vi "Parse BOM Raw Data Array.vi"(8 "Error in":errorcluster caption="Error in (no error)", 11 "BOM JSON String":string="[\n  {\n    \"id\":57,\n    \"order\":\"2.00000000000000000000\",\n    \"Full PN\":\"40-00000 Rev.A\",\n    \"External Part Number\":\"RRJTLR\",\n    \"Manufacturer\":[\n      {\n        \"id\":2,\n        \"value\":\"Schlegel Electrokontakt GMBH\",\n        \"order\":\"2.00000000000000000000\"\n      }\n    ],\n    \"System\":{\n      \"id\":2963,\n      \"value\":\"DC Power Supply\",\n      \"color\":\"orange\"\n    },\n    \"Item description\":\"Silver pushbutton with illuminated ring\",\n    \"Price per unit\":\"0.00\",\n    \"Image\":[\n      {\n        \"url\":\"http://localhost/media/user_files/vs8lqWLDz7IiCZOwmtUNUbGmxWH526uQ_3725ba00b9b12365f0e4d102f8b4c18b09270bde56499f1310e5468db4989185.jpg\",\n        \"thumbnails\":{\n          \"tiny\":{\n            \"url\":\"http://localhost/media/thumbnails/tiny/vs8lqWLDz7IiCZOwmtUNUbGmxWH526uQ_3725ba00b9b12365f0e4d102f8b4c18b09270bde56499f1310e5468db4989185.jpg\",\n            \"width\":null,\n            \"height\":21\n          },\n          \"small\":{\n            \"url\":\"http://localhost/media/thumbnails/small/vs8lqWLDz7IiCZOwmtUNUbGmxWH526uQ_3725ba00b9b12365f0e4d102f8b4c18b09270bde56499f1310e5468db4989185.jpg\",\n            \"width\":48,\n            \"height\":48\n          },\n          \"card_cover\":{\n            \"url\":\"http://localhost/media/thumbnails/card_cover/vs8lqWLDz7IiCZOwmtUNUbGmxWH526uQ_3725ba00b9b12365f0e4d102f8b4c18b09270bde56499f1310e5468db4989185.jpg\",\n            \"width\":300,\n            \"height\":160\n          }\n        },\n        \"visible_name\":\"2XATeTQaoip3EBPiJcHf6fjdvHM94na...de56499f1310e5468db4989185.jpg\",\n        \"name\":\"vs8lqWLDz7IiCZOwmtUNUbGmxWH526uQ_3725ba00b9b12365f0e4d102f8b4c18b09270bde56499f1310e5468db4989185.jpg\",\n        \"size\":3722,\n        \"mime_type\":\"image/jpeg\",\n        \"is_image\":true,\n        \"image_width\":300,\n        \"image_height\":168,\n        \"uploaded_at\":\"2025-05-04T14:40:33.054106+00:00\"\n      }\n    ],\n    \"Source\":\"kahane.co.il\",\n    \"Order Items\":[\n      {\n        \"id\":1,\n        \"value\":\"8e1b2002-0c82-4bb7-87aa-3665b154ad1b\",\n        \"order\":\"1.00000000000000000000\"\n      }\n    ],\n    \"Datasheet\":[],\n    \"Part of a set\":[\n      {\n        \"id\":57,\n        \"value\":\"40-00000 Rev.A\",\n        \"order\":\"2.00000000000000000000\"\n      },\n      {\n        \"id\":58,\n        \"value\":\"40-00001 Rev.A\",\n        \"order\":\"3.00000000000000000000\"\n      },\n      {\n        \"id\":59,\n        \"value\":\"40-00002 Rev.A\",\n        \"order\":\"4.00000000000000000000\"\n      }\n    ],\n    \"State\":{\n      \"id\":3001,\n      \"value\":\"Unknown\",\n      \"color\":\"dark-orange\"\n    },\n    \"Part Number\":\"40-00000\",\n    \"Revision\":\"A\",\n    \"Notes\":null,\n    \"Sourced By\":null,\n    \"Containing\":[],\n    \"Contained by\":[]\n  },\n  {\n    \"id\":58,\n    \"order\":\"3.00000000000000000000\",\n    \"Full PN\":\"40-00001 Rev.A\",\n    \"External Part Number\":\"BFL5\",\n    \"Manufacturer\":[\n      {\n        \"id\":2,\n        \"value\":\"Schlegel Electrokontakt GMBH\",\n        \"order\":\"2.00000000000000000000\"\n      }\n    ],\n    \"System\":{\n      \"id\":2963,\n      \"value\":\"DC Power Supply\",\n      \"color\":\"orange\"\n    },\n    \"Item description\":\"lluminated contact block, maintained (latching), fits W2x4,6d light bulb\",\n    \"Price per unit\":\"0.00\",\n    \"Image\":[\n      {\n        \"url\":\"http://localhost/media/user_files/xij9XnHAyoORm72XwG7yoW01mk4UuKpd_da0cb6cb7c3498cd2d6cf9448262cb0dac37b09af222fbe05ff221e70527cfe5.jpg\",\n        \"thumbnails\":{\n          \"tiny\":{\n            \"url\":\"http://localhost/media/thumbnails/tiny/xij9XnHAyoORm72XwG7yoW01mk4UuKpd_da0cb6cb7c3498cd2d6cf9448262cb0dac37b09af222fbe05ff221e70527cfe5.jpg\",\n            \"width\":null,\n            \"height\":21\n          },\n          \"small\":{\n            \"url\":\"http://localhost/media/thumbnails/small/xij9XnHAyoORm72XwG7yoW01mk4UuKpd_da0cb6cb7c3498cd2d6cf9448262cb0dac37b09af222fbe05ff221e70527cfe5.jpg\",\n            \"width\":48,\n            \"height\":48\n          },\n          \"card_cover\":{\n            \"url\":\"http://localhost/media/thumbnails/card_cover/xij9XnHAyoORm72XwG7yoW01mk4UuKpd_da0cb6cb7c3498cd2d6cf9448262cb0dac37b09af222fbe05ff221e70527cfe5.jpg\",\n            \"width\":300,\n            \"height\":160\n          }\n        },\n        \"visible_name\":\"YoEUw7VMUVzghdb1WstSkFV6s8zxhqv...9af222fbe05ff221e70527cfe5.jpg\",\n        \"name\":\"xij9XnHAyoORm72XwG7yoW01mk4UuKpd_da0cb6cb7c3498cd2d6cf9448262cb0dac37b09af222fbe05ff221e70527cfe5.jpg\",\n        \"size\":91279,\n        \"mime_type\":\"image/jpeg\",\n        \"is_image\":true,\n        \"image_width\":1500,\n        \"image_height\":1500,\n        \"uploaded_at\":\"2025-05-04T14:40:36.115953+00:00\"\n      }\n    ],\n    \"Source\":\"kahane.co.il\",\n    \"Order Items\":[\n      {\n        \"id\":1,\n        \"value\":\"8e1b2002-0c82-4bb7-87aa-3665b154ad1b\",\n        \"order\":\"1.00000000000000000000\"\n      }\n    ],\n    \"Datasheet\":[],\n    \"Part of a set\":[\n      {\n        \"id\":57,\n        \"value\":\"40-00000 Rev.A\",\n        \"order\":\"2.00000000000000000000\"\n      },\n      {\n        \"id\":58,\n        \"value\":\"40-00001 Rev.A\",\n        \"order\":\"3.00000000000000000000\"\n      },\n      {\n        \"id\":59,\n        \"value\":\"40-00002 Rev.A\",\n        \"order\":\"4.00000000000000000000\"\n      }\n    ],\n    \"State\":{\n      \"id\":3001,\n      \"value\":\"Unknown\",\n      \"color\":\"dark-orange\"\n    },\n    \"Part Number\":\"40-00001\",\n    \"Revision\":\"A\",\n    \"Notes\":null,\n    \"Sourced By\":null,\n    \"Containing\":[\n      {\n        \"id\":1,\n        \"value\":\"1\",\n        \"order\":\"1.00000000000000000000\"\n      }\n    ],\n    \"Contained by\":[]\n  },\n  {\n    \"id\":60,\n    \"order\":\"5.00000000000000000000\",\n    \"Full PN\":\"40-00003 Rev.A\",\n    \"External Part Number\":\"DD11.0124.1111\",\n    \"Manufacturer\":[\n      {\n        \"id\":12,\n        \"value\":\"SCHURTER Inc.\",\n        \"order\":\"12.00000000000000000000\"\n      }\n    ],\n    \"System\":{\n      \"id\":2964,\n      \"value\":\"AC-Mains Compartment\",\n      \"color\":\"dark-gray\"\n    },\n    \"Item description\":\"PEM (Power Entry Module)\",\n    \"Price per unit\":\"22.34\",\n    \"Image\":[\n      {\n        \"url\":\"http://localhost/media/user_files/pcnZZdvA6PzNm2eRl6mPykJmRlUZAuwe_2c494bbc853f7bcd2029a34fd083a93657d536910bba6dd04ab3ca52d19aafe1.jpg\",\n        \"thumbnails\":{\n          \"tiny\":{\n            \"url\":\"http://localhost/media/thumbnails/tiny/pcnZZdvA6PzNm2eRl6mPykJmRlUZAuwe_2c494bbc853f7bcd2029a34fd083a93657d536910bba6dd04ab3ca52d19aafe1.jpg\",\n            \"width\":null,\n            \"height\":21\n          },\n          \"small\":{\n            \"url\":\"http://localhost/media/thumbnails/small/pcnZZdvA6PzNm2eRl6mPykJmRlUZAuwe_2c494bbc853f7bcd2029a34fd083a93657d536910bba6dd04ab3ca52d19aafe1.jpg\",\n            \"width\":48,\n            \"height\":48\n          },\n          \"card_cover\":{\n            \"url\":\"http://localhost/media/thumbnails/card_cover/pcnZZdvA6PzNm2eRl6mPykJmRlUZAuwe_2c494bbc853f7bcd2029a34fd083a93657d536910bba6dd04ab3ca52d19aafe1.jpg\",\n            \"width\":300,\n            \"height\":160\n          }\n        },\n        \"visible_name\":\"X6i6bjQqts9wxYk1SHMpfwGuSOBZfP8...910bba6dd04ab3ca52d19aafe1.jpg\",\n        \"name\":\"pcnZZdvA6PzNm2eRl6mPykJmRlUZAuwe_2c494bbc853f7bcd2029a34fd083a93657d536910bba6dd04ab3ca52d19aafe1.jpg\",\n        \"size\":155114,\n        \"mime_type\":\"image/jpeg\",\n        \"is_image\":true,\n        \"image_width\":640,\n        \"image_height\":640,\n        \"uploaded_at\":\"2025-05-04T14:42:05.140492+00:00\"\n      }\n    ],\n    \"Source\":\"https://www.mouser.co.il/ProductDetail/Schurter/DD11.0124.1111?qs=PdaBPmf3Bciq6aQ7pgA2rg%3D%3D\",\n    \"Order Items\":[\n      {\n        \"id\":4,\n        \"value\":\"d10ecc9b-78da-4c78-a469-db714dbc25c0\",\n        \"order\":\"4.00000000000000000000\"\n      }\n    ],\n    \"Datasheet\":[\n      {\n        \"url\":\"http://localhost/media/user_files/vbbFIILhHm3KXHES6rOyYGhSZbqZZKmr_1db97cff0daf3ff16140aba71b86a4556479dc26ed8a657b23d7a6a0d3ea0fe7.pdf\",\n        \"thumbnails\":null,\n        \"visible_name\":\"typ_DD11.pdf\",\n        \"name\":\"vbbFIILhHm3KXHES6rOyYGhSZbqZZKmr_1db97cff0daf3ff16140aba71b86a4556479dc26ed8a657b23d7a6a0d3ea0fe7.pdf\",\n        \"size\":450651,\n        \"mime_type\":\"application/pdf\",\n        \"is_image\":false,\n        \"image_width\":null,\n        \"image_height\":null,\n        \"uploaded_at\":\"2025-09-16T13:54:47.399442+00:00\"\n      }\n    ],\n    \"Part of a set\":[\n      {\n        \"id\":88,\n        \"value\":\"40-00004 Rev.A\",\n        \"order\":\"5.50000000000000000000\"\n      },\n      {\n        \"id\":106,\n        \"value\":\"40-00036 Rev.A\",\n        \"order\":\"49.00000000000000000000\"\n      }\n    ],\n    \"State\":{\n      \"id\":3004,\n      \"value\":\"Not Used\",\n      \"color\":\"darker-red\"\n    },\n    \"Part Number\":\"40-00003\",\n    \"Revision\":\"A\",\n    \"Notes\":\"https://www.schurter.com/en/datasheet/DD11\",\n    \"Sourced By\":null,\n    \"Containing\":[],\n    \"Contained by\":[]\n  },\n  {\n    \"id\":88,\n    \"order\":\"5.50000000000000000000\",\n    \"Full PN\":\"40-00004 Rev.A\",\n    \"External Part Number\":\"4301.1403\",\n    \"Manufacturer\":[\n      {\n        \"id\":12,\n        \"value\":\"SCHURTER Inc.\",\n        \"order\":\"12.00000000000000000000\"\n      }\n    ],\n    \"System\":{\n      \"id\":2964,\n      \"value\":\"AC-Mains Compartment\",\n      \"color\":\"dark-gray\"\n    },\n    \"Item description\":\"X-SAFE - fuse drawer for PEM, with a safety latch\",\n    \"Price per unit\":\"5.92\",\n    \"Image\":[\n      {\n        \"url\":\"http://localhost/media/user_files/b9PQ9D2agU90lk8fiJHKVdbJgYuHDrxA_0a269b6470f77db68892e544b9f09636c05bce2a87623908e77a63c21f095bb1.jpg\",\n        \"thumbnails\":{\n          \"tiny\":{\n            \"url\":\"http://localhost/media/thumbnails/tiny/b9PQ9D2agU90lk8fiJHKVdbJgYuHDrxA_0a269b6470f77db68892e544b9f09636c05bce2a87623908e77a63c21f095bb1.jpg\",\n            \"width\":null,\n            \"height\":21\n          },\n          \"small\":{\n            \"url\":\"http://localhost/media/thumbnails/small/b9PQ9D2agU90lk8fiJHKVdbJgYuHDrxA_0a269b6470f77db68892e544b9f09636c05bce2a87623908e77a63c21f095bb1.jpg\",\n            \"width\":48,\n            \"height\":48\n          },\n          \"card_cover\":{\n            \"url\":\"http://localhost/media/thumbnails/card_cover/b9PQ9D2agU90lk8fiJHKVdbJgYuHDrxA_0a269b6470f77db68892e544b9f09636c05bce2a87623908e77a63c21f095bb1.jpg\",\n            \"width\":300,\n            \"height\":160\n          }\n        },\n        \"visible_name\":\"zSFjHSVLACFgVfaKKjybtbyaMGODCr1...2a87623908e77a63c21f095bb1.jpg\",\n        \"name\":\"b9PQ9D2agU90lk8fiJHKVdbJgYuHDrxA_0a269b6470f77db68892e544b9f09636c05bce2a87623908e77a63c21f095bb1.jpg\",\n        \"size\":36754,\n        \"mime_type\":\"image/jpeg\",\n        \"is_image\":true,\n        \"image_width\":640,\n        \"image_height\":640,\n        \"uploaded_at\":\"2025-05-04T14:42:13.530897+00:00\"\n      }\n    ],\n    \"Source\":\"https://www.mouser.co.il/ProductDetail/Schurter/43011403?qs=fxxZwZgTYwA8B4fs8Del4g%3D%3D\",\n    \"Order Items\":[\n      {\n        \"id\":26,\n        \"value\":\"ed936862-b2ea-4a92-bcf3-415caf9fd1b8\",\n        \"order\":\"24.00000000000000000000\"\n      }\n    ],\n    \"Datasheet\":[\n      {\n        \"url\":\"http://localhost/media/user_files/IaXoEoXXF770q5qdPQ7veQXPOSUxfc2Z_c8cd0e02514c181b789db27b58a6af8b96eac526016ed074cd766ec4178ae1ca.pdf\",\n        \"thumbnails\":null,\n        \"visible_name\":\"typ_Fusedrawer_2.pdf\",\n        \"name\":\"IaXoEoXXF770q5qdPQ7veQXPOSUxfc2Z_c8cd0e02514c181b789db27b58a6af8b96eac526016ed074cd766ec4178ae1ca.pdf\",\n        \"size\":324458,\n        \"mime_type\":\"application/pdf\",\n        \"is_image\":false,\n        \"image_width\":null,\n        \"image_height\":null,\n        \"uploaded_at\":\"2025-04-21T07:07:31.672129+00:00\"\n      }\n    ],\n    \"Part of a set\":[\n      {\n        \"id\":60,\n        \"value\":\"40-00003 Rev.A\",\n        \"order\":\"5.00000000000000000000\"\n      }\n    ],\n    \"State\":{\n      \"id\":3004,\n      \"value\":\"Not Used\",\n      \"color\":\"darker-red\"\n    },\n    \"Part Number\":\"40-00004\",\n    \"Revision\":\"A\",\n    \"Notes\":null,\n    \"Sourced By\":null,\n    \"Containing\":[],\n    \"Contained by\":[]\n  },\n  {\n    \"id\":89,\n    \"order\":\"5.66666666666666696273\",\n    \"Full PN\":\"40-00005 Rev.A\",\n    \"External Part Number\":\"4301.1401\",\n    \"Manufacturer\":[\n      {\n        \"id\":12,\n        \"value\":\"SCHURTER Inc.\",\n        \"order\":\"12.00000000000000000000\"\n      }\n    ],\n    \"System\":{\n      \"id\":2964,\n      \"value\":\"AC-Mains Compartment\",\n      \"color\":\"dark-gray\"\n    },\n    \"Item description\":\"Regular fuse drawer for PEM\",\n    \"Price per unit\":\"5.92\",\n    \"Image\":[\n      {\n        \"url\":\"http://localhost/media/user_files/TiX48LEpV2v5fHHt86AamKWUkJS227LT_4736367127e316354bec99c45b1098f4beba6f8b61afc6189c041e5d23bb62d5.jpg\",\n        \"thumbnails\":{\n          \"tiny\":{\n            \"url\":\"http://localhost/media/thumbnails/tiny/TiX48LEpV2v5fHHt86AamKWUkJS227LT_4736367127e316354bec99c45b1098f4beba6f8b61afc6189c041e5d23bb62d5.jpg\",\n            \"width\":null,\n            \"height\":21\n          },\n          \"small\":{\n            \"url\":\"http://localhost/media/thumbnails/small/TiX48LEpV2v5fHHt86AamKWUkJS227LT_4736367127e316354bec99c45b1098f4beba6f8b61afc6189c041e5d23bb62d5.jpg\",\n            \"width\":48,\n            \"height\":48\n          },\n          \"card_cover\":{\n            \"url\":\"http://localhost/media/thumbnails/card_cover/TiX48LEpV2v5fHHt86AamKWUkJS227LT_4736367127e316354bec99c45b1098f4beba6f8b61afc6189c041e5d23bb62d5.jpg\",\n            \"width\":300,\n            \"height\":160\n          }\n        },\n        \"visible_name\":\"782JdDNozjC5G03DKBOyyDdqBnQ7tux...8b61afc6189c041e5d23bb62d5.jpg\",\n        \"name\":\"TiX48LEpV2v5fHHt86AamKWUkJS227LT_4736367127e316354bec99c45b1098f4beba6f8b61afc6189c041e5d23bb62d5.jpg\",\n        \"size\":135847,\n        \"mime_type\":\"image/jpeg\",\n        \"is_image\":true,\n        \"image_width\":640,\n        \"image_height\":640,\n        \"uploaded_at\":\"2025-05-04T14:42:23.334111+00:00\"\n      }\n    ],\n    \"Source\":\"https://www.digikey.com/en/products/detail/schurter-inc/4301-1401/569920\",\n    \"Order Items\":[],\n    \"Datasheet\":[\n      {\n        \"url\":\"http://localhost/media/user_files/IaXoEoXXF770q5qdPQ7veQXPOSUxfc2Z_c8cd0e02514c181b789db27b58a6af8b96eac526016ed074cd766ec4178ae1ca.pdf\",\n        \"thumbnails\":null,\n        \"visible_name\":\"typ_Fusedrawer_2.pdf\",\n        \"name\":\"IaXoEoXXF770q5qdPQ7veQXPOSUxfc2Z_c8cd0e02514c181b789db27b58a6af8b96eac526016ed074cd766ec4178ae1ca.pdf\",\n        \"size\":324458,\n        \"mime_type\":\"application/pdf\",\n        \"is_image\":false,\n        \"image_width\":null,\n        \"image_height\":null,\n        \"uploaded_at\":\"2025-04-21T07:07:31.672129+00:00\"\n      }\n    ],\n    \"Part of a set\":[\n      {\n        \"id\":60,\n        \"value\":\"40-00003 Rev.A\",\n        \"order\":\"5.00000000000000000000\"\n      }\n    ],\n    \"State\":{\n      \"id\":3004,\n      \"value\":\"Not Used\",\n      \"color\":\"darker-red\"\n    },\n    \"Part Number\":\"40-00005\",\n    \"Revision\":\"A\",\n    \"Notes\":null,\n    \"Sourced By\":null,\n    \"Containing\":[],\n    \"Contained by\":[]\n  },\n  {\n    \"id\":61,\n    \"order\":\"6.00000000000000000000\",\n    \"Full PN\":\"40-00006 Rev.A\",\n    \"External Part Number\":\"7-6609089-9\",\n    \"Manufacturer\":[\n      {\n        \"id\":7,\n        \"value\":\"Corcom\",\n        \"order\":\"7.00000000000000000000\"\n      }\n    ],\n    \"System\":{\n      \"id\":2964,\n      \"value\":\"AC-Mains Compartment\",\n      \"color\":\"dark-gray\"\n    },\n    \"Item description\":\"Power Line Filters 16WGD3=F8248C\",\n    \"Price per unit\":\"8.51\",\n    \"Image\":[\n      {\n        \"url\":\"http://localhost/media/user_files/6RdTE1D7KRHhgbWpSWzu2EscwZCoaqpR_46837f9a5495f70d14a252a3a134dac612f8d6cae1d84484480ca4b83f8fd42c.jpg\",\n        \"thumbnails\":{\n          \"tiny\":{\n            \"url\":\"http://localhost/media/thumbnails/tiny/6RdTE1D7KRHhgbWpSWzu2EscwZCoaqpR_46837f9a5495f70d14a252a3a134dac612f8d6cae1d84484480ca4b83f8fd42c.jpg\",\n            \"width\":null,\n            \"height\":21\n          },\n          \"small\":{\n            \"url\":\"http://localhost/media/thumbnails/small/6RdTE1D7KRHhgbWpSWzu2EscwZCoaqpR_46837f9a5495f70d14a252a3a134dac612f8d6cae1d84484480ca4b83f8fd42c.jpg\",\n            \"width\":48,\n            \"height\":48\n          },\n          \"card_cover\":{\n            \"url\":\"http://localhost/media/thumbnails/card_cover/6RdTE1D7KRHhgbWpSWzu2EscwZCoaqpR_46837f9a5495f70d14a252a3a134dac612f8d6cae1d84484480ca4b83f8fd42c.jpg\",\n            \"width\":300,\n            \"height\":160\n          }\n        },\n        \"visible_name\":\"YG0CuAis4PEFZ6jV2wikXzNOD9JQJj9...cae1d84484480ca4b83f8fd42c.jpg\",\n        \"name\":\"6RdTE1D7KRHhgbWpSWzu2EscwZCoaqpR_46837f9a5495f70d14a252a3a134dac612f8d6cae1d84484480ca4b83f8fd42c.jpg\",\n        \"size\":13433,\n        \"mime_type\":\"image/jpeg\",\n        \"is_image\":true,\n        \"image_width\":200,\n        \"image_height\":200,\n        \"uploaded_at\":\"2025-05-04T14:42:28.459727+00:00\"\n      }\n    ],\n    \"Source\":\"\",\n    \"Order Items\":[\n      {\n        \"id\":5,\n        \"value\":\"24f0c6de-95f2-4a56-a6d7-d3f0d7cedeeb\",\n        \"order\":\"5.00000000000000000000\"\n      }\n    ],\n    \"Datasheet\":[],\n    \"Part of a set\":[],\n    \"State\":{\n      \"id\":3003,\n      \"value\":\"EOL\",\n      \"color\":\"darker-red\"\n    },\n    \"Part Number\":\"40-00006\",\n    \"Revision\":\"A\",\n    \"Notes\":null,\n    \"Sourced By\":null,\n    \"Containing\":[],\n    \"Contained by\":[]\n  },\n  {\n    \"id\":62,\n    \"order\":\"7.00000000000000000000\",\n    \"Full PN\":\"20-00005 Rev.A\",\n    \"External Part Number\":\"6225-NAAA-BZZZ-000\",\n    \"Manufacturer\":[\n      {\n        \"id\":3,\n        \"value\":\"Herga\",\n        \"order\":\"3.00000000000000000000\"\n      }\n    ],\n    \"System\":{\n      \"id\":2965,\n      \"value\":\"Foot Switch\",\n      \"color\":\"deep-dark-orange\"\n    },\n    \"Item description\":\"Herga IPX2 Foot switch & Cover\",\n    \"Price per unit\":\"130.00\",\n    \"Image\":[\n      {\n        \"url\":\"http://localhost/media/user_files/Ur7CwAS4qUFcIgKpFr5Ltb20DF3wbEPg_2bdf504d87814b9a76fd2f3ceaa877b83abc5920820db879d613f6fb6b1b03dd.png\",\n        \"thumbnails\":{\n          \"tiny\":{\n            \"url\":\"http://localhost/media/thumbnails/tiny/Ur7CwAS4qUFcIgKpFr5Ltb20DF3wbEPg_2bdf504d87814b9a76fd2f3ceaa877b83abc5920820db879d613f6fb6b1b03dd.png\",\n            \"width\":null,\n            \"height\":21\n          },\n          \"small\":{\n            \"url\":\"http://localhost/media/thumbnails/small/Ur7CwAS4qUFcIgKpFr5Ltb20DF3wbEPg_2bdf504d87814b9a76fd2f3ceaa877b83abc5920820db879d613f6fb6b1b03dd.png\",\n            \"width\":48,\n            \"height\":48\n          },\n          \"card_cover\":{\n            \"url\":\"http://localhost/media/thumbnails/card_cover/Ur7CwAS4qUFcIgKpFr5Ltb20DF3wbEPg_2bdf504d87814b9a76fd2f3ceaa877b83abc5920820db879d613f6fb6b1b03dd.png\",\n            \"width\":300,\n            \"height\":160\n          }\n        },\n        \"visible_name\":\"image.png\",\n        \"name\":\"Ur7CwAS4qUFcIgKpFr5Ltb20DF3wbEPg_2bdf504d87814b9a76fd2f3ceaa877b83abc5920820db879d613f6fb6b1b03dd.png\",\n        \"size\":57867,\n        \"mime_type\":\"image/png\",\n        \"is_image\":true,\n        \"image_width\":308,\n        \"image_height\":271,\n        \"uploaded_at\":\"2025-05-04T14:44:15.118370+00:00\"\n      }\n    ],\n    \"Source\":\"https://amironic.co.il/products/footswitches/medical/62256-footswitch/\",\n    \"Order Items\":[\n      {\n        \"id\":9,\n        \"value\":\"e004d451-8317-4ca6-9c7c-2ea5634e1e14\",\n        \"order\":\"7.00000000000000000000\"\n      }\n    ],\n    \"Datasheet\":[],\n    \"Part of a set\":[],\n    \"State\":{\n      \"id\":3001,\n      \"value\":\"Unknown\",\n      \"color\":\"dark-orange\"\n    },\n    \"Part Number\":\"20-00005\",\n    \"Revision\":\"A\",\n    \"Notes\":null,\n    \"Sourced By\":null,\n    \"Containing\":[],\n    \"Contained by\":[]\n  },\n  {\n    \"id\":63,\n    \"order\":\"8.00000000000000000000\",\n    \"Full PN\":\"40-00015 Rev.A\",\n    \"External Part Number\":\"NC3FP-1\",\n    \"Manufacturer\":[\n      {\n        \"id\":4,\n        \"value\":\"Neutrik\",\n        \"order\":\"4.00000000000000000000\"\n      }\n    ],\n    \"System\":{\n      \"id\":2965,\n      \"value\":\"Foot Switch\",\n      \"color\":\"deep-dark-orange\"\n    },\n    \"Item description\":\"Neutrik XLR Connector,\\n3 Contacts,\\nSocket,\\nPanel Mount,\\nSilver Plated Contacts,\\nMetal Body,\\nP Series\",\n    \"Price per unit\":\"4.25\",\n    \"Image\":[\n      {\n        \"url\":\"http://localhost/media/user_files/gUVNeCX8zQ8SSPJcR9UdpAhg1PoZhF7d_56a38d39cc9a2180d9773965e248738ecdbe8260c8f2740c123a37b2e6af85eb.jpg\",\n        \"thumbnails\":{\n          \"tiny\":{\n            \"url\":\"http://localhost/media/thumbnails/tiny/gUVNeCX8zQ8SSPJcR9UdpAhg1PoZhF7d_56a38d39cc9a2180d9773965e248738ecdbe8260c8f2740c123a37b2e6af85eb.jpg\",\n            \"width\":null,\n            \"height\":21\n          },\n          \"small\":{\n            \"url\":\"http://localhost/media/thumbnails/small/gUVNeCX8zQ8SSPJcR9UdpAhg1PoZhF7d_56a38d39cc9a2180d9773965e248738ecdbe8260c8f2740c123a37b2e6af85eb.jpg\",\n            \"width\":48,\n            \"height\":48\n          },\n          \"card_cover\":{\n            \"url\":\"http://localhost/media/thumbnails/card_cover/gUVNeCX8zQ8SSPJcR9UdpAhg1PoZhF7d_56a38d39cc9a2180d9773965e248738ecdbe8260c8f2740c123a37b2e6af85eb.jpg\",\n            \"width\":300,\n            \"height\":160\n          }\n        },\n        \"visible_name\":\"lbjyVtrCSiIL4WZBQ6F2smMsktHr2Wk...60c8f2740c123a37b2e6af85eb.jpg\",\n        \"name\":\"gUVNeCX8zQ8SSPJcR9UdpAhg1PoZhF7d_56a38d39cc9a2180d9773965e248738ecdbe8260c8f2740c123a37b2e6af85eb.jpg\",\n        \"size\":3574,\n        \"mime_type\":\"image/jpeg\",\n        \"is_image\":true,\n        \"image_width\":260,\n        \"image_height\":194,\n        \"uploaded_at\":\"2025-05-04T14:44:26.977753+00:00\"\n      }\n    ],\n    \"Source\":\"https://il.farnell.com/neutrik/nc3fp1/socket-xlr-panel-3pole/dp/308780\",\n    \"Order Items\":[\n      {\n        \"id\":6,\n        \"value\":\"75dcac69-1638-43b1-99f2-3190100396e9\",\n        \"order\":\"6.00000000000000000000\"\n      }\n    ],\n    \"Datasheet\":[],\n    \"Part of a set\":[],\n    \"State\":{\n      \"id\":3004,\n      \"value\":\"Not Used\",\n      \"color\":\"darker-red\"\n    },\n    \"Part Number\":\"40-00015\",\n    \"Revision\":\"A\",\n    \"Notes\":null,\n    \"Sourced By\":null,\n    \"Containing\":[],\n    \"Contained by\":[]\n  },\n  {\n    \"id\":64,\n    \"order\":\"9.00000000000000000000\",\n    \"Full PN\":\"40-00016 Rev.A\",\n    \"External Part Number\":\"NC3MX-B-D\",\n    \"Manufacturer\":[\n      {\n        \"id\":4,\n        \"value\":\"Neutrik\",\n        \"order\":\"4.00000000000000000000\"\n      }\n    ],\n    \"System\":{\n      \"id\":2965,\n      \"value\":\"Foot Switch\",\n      \"color\":\"deep-dark-orange\"\n    },\n    \"Item description\":\"Neutrik XLR Connector,\\n3 Contacts,\\nPlug,\\nCable Mount,\\nBrass solder contacts\\nZinc Body,\\nX Series?\",\n    \"Price per unit\":\"5.90\",\n    \"Image\":[\n      {\n        \"url\":\"http://localhost/media/user_files/0QC5oIpDGIjk3EeU0WKW3j5PQFF4XAyD_67d096909fd028081e4a59b945eb0190b656a8a284d6ee2babffa76f1e448c43.jpg\",\n        \"thumbnails\":{\n          \"tiny\":{\n            \"url\":\"http://localhost/media/thumbnails/tiny/0QC5oIpDGIjk3EeU0WKW3j5PQFF4XAyD_67d096909fd028081e4a59b945eb0190b656a8a284d6ee2babffa76f1e448c43.jpg\",\n            \"width\":null,\n            \"height\":21\n          },\n          \"small\":{\n            \"url\":\"http://localhost/media/thumbnails/small/0QC5oIpDGIjk3EeU0WKW3j5PQFF4XAyD_67d096909fd028081e4a59b945eb0190b656a8a284d6ee2babffa76f1e448c43.jpg\",\n            \"width\":48,\n            \"height\":48\n          },\n          \"card_cover\":{\n            \"url\":\"http://localhost/media/thumbnails/card_cover/0QC5oIpDGIjk3EeU0WKW3j5PQFF4XAyD_67d096909fd028081e4a59b945eb0190b656a8a284d6ee2babffa76f1e448c43.jpg\",\n            \"width\":300,\n            \"height\":160\n          }\n        },\n        \"visible_name\":\"rnl7CYMo71cGT2v9kbxSgXmQtQuDqv5...a284d6ee2babffa76f1e448c43.jpg\",\n        \"name\":\"0QC5oIpDGIjk3EeU0WKW3j5PQFF4XAyD_67d096909fd028081e4a59b945eb0190b656a8a284d6ee2babffa76f1e448c43.jpg\",\n        \"size\":21672,\n        \"mime_type\":\"image/jpeg\",\n        \"is_image\":true,\n        \"image_width\":500,\n        \"image_height\":338,\n        \"uploaded_at\":\"2025-05-04T14:44:37.621115+00:00\"\n      }\n    ],\n    \"Source\":\"https://il.farnell.com/neutrik/nc3mx/conn-xlr-audio-plug-3pos-cable/dp/308766\",\n    \"Order Items\":[\n      {\n        \"id\":28,\n        \"value\":\"c19f1736-8a8a-433e-970a-e07ab82f5ef1\",\n        \"order\":\"26.00000000000000000000\"\n      }\n    ],\n    \"Datasheet\":[\n      {\n        \"url\":\"http://localhost/media/user_files/5kcFh2mTKdRSIZxGYdAHyUonOHY6sHbP_988d346e9c249430ca176266ef5fa3d7a70e07d4628adfdcac1a2db683ca6182.pdf\",\n        \"thumbnails\":null,\n        \"visible_name\":\"NC3MX-B-D.pdf\",\n        \"name\":\"5kcFh2mTKdRSIZxGYdAHyUonOHY6sHbP_988d346e9c249430ca176266ef5fa3d7a70e07d4628adfdcac1a2db683ca6182.pdf\",\n        \"size\":110744,\n        \"mime_type\":\"application/pdf\",\n        \"is_image\":false,\n        \"image_width\":null,\n        \"image_height\":null,\n        \"uploaded_at\":\"2025-04-22T07:41:51.422070+00:00\"\n      }\n    ],\n    \"Part of a set\":[],\n    \"State\":{\n      \"id\":3003,\n      \"value\":\"EOL\",\n      \"color\":\"darker-red\"\n    },\n    \"Part Number\":\"40-00016\",\n    \"Revision\":\"A\",\n    \"Notes\":null,\n    \"Sourced By\":null,\n    \"Containing\":[],\n    \"Contained by\":[]\n  },\n  {\n    \"id\":67,\n    \"order\":\"12.00000000000000000000\",\n    \"Full PN\":\"20-00006 Rev.A\",\n    \"External Part Number\":\"PC4-M6M\",\n    \"Manufacturer\":[\n      {\n        \"id\":6,\n        \"value\":\"Pisco\",\n        \"order\":\"6.00000000000000000000\"\n      }\n    ],\n    \"System\":{\n      \"id\":2966,\n      \"value\":\"Gas supply\",\n      \"color\":\"darker-brown\"\n    },\n    \"Item description\":\"Straight Fitting M6\",\n    \"Price per unit\":\"1.62\",\n    \"Image\":[\n      {\n        \"url\":\"http://localhost/media/user_files/Zv7h0kB5KKhKWky0H3PHyZQLJB1n8Z99_9309ddc96dedec59da725e14ca74acc95e98e5a36262b77648ca3188cbea6f6e.jpg\",\n        \"thumbnails\":{\n          \"tiny\":{\n            \"url\":\"http://localhost/media/thumbnails/tiny/Zv7h0kB5KKhKWky0H3PHyZQLJB1n8Z99_9309ddc96dedec59da725e14ca74acc95e98e5a36262b77648ca3188cbea6f6e.jpg\",\n            \"width\":null,\n            \"height\":21\n          },\n          \"small\":{\n            \"url\":\"http://localhost/media/thumbnails/small/Zv7h0kB5KKhKWky0H3PHyZQLJB1n8Z99_9309ddc96dedec59da725e14ca74acc95e98e5a36262b77648ca3188cbea6f6e.jpg\",\n            \"width\":48,\n            \"height\":48\n          },\n          \"card_cover\":{\n            \"url\":\"http://localhost/media/thumbnails/card_cover/Zv7h0kB5KKhKWky0H3PHyZQLJB1n8Z99_9309ddc96dedec59da725e14ca74acc95e98e5a36262b77648ca3188cbea6f6e.jpg\",\n            \"width\":300,\n            \"height\":160\n          }\n        },\n        \"visible_name\":\"LtvSOv4XvnJ3XiuAteI39jNUG1nJKE1...a36262b77648ca3188cbea6f6e.jpg\",\n        \"name\":\"Zv7h0kB5KKhKWky0H3PHyZQLJB1n8Z99_9309ddc96dedec59da725e14ca74acc95e98e5a36262b77648ca3188cbea6f6e.jpg\",\n        \"size\":65155,\n        \"mime_type\":\"image/jpeg\",\n        \"is_image\":true,\n        \"image_width\":768,\n        \"image_height\":768,\n        \"uploaded_at\":\"2025-05-04T14:45:03.166187+00:00\"\n      }\n    ],\n    \"Source\":\"https://www.conlog.co.il/pisco/\",\n    \"Order Items\":[\n      {\n        \"id\":10,\n        \"value\":\"b36e1465-c33b-4277-b59c-cc84afdc6479\",\n        \"order\":\"8.00000000000000000000\"\n      }\n    ],\n    \"Datasheet\":[],\n    \"Part of a set\":[],\n    \"State\":{\n      \"id\":3002,\n      \"value\":\"Production & Used\",\n      \"color\":\"darker-green\"\n    },\n    \"Part Number\":\"20-00006\",\n    \"Revision\":\"A\",\n    \"Notes\":null,\n    \"Sourced By\":null,\n    \"Containing\":[],\n    \"Contained by\":[]\n  },\n  {\n    \"id\":68,\n    \"order\":\"13.00000000000000000000\",\n    \"Full PN\":\"20-00007 Rev.A\",\n    \"External Part Number\":\"PC4-M5M\",\n    \"Manufacturer\":[\n      {\n        \"id\":6,\n        \"value\":\"Pisco\",\n        \"order\":\"6.00000000000000000000\"\n      }\n    ],\n    \"System\":{\n      \"id\":2966,\n      \"value\":\"Gas supply\",\n      \"color\":\"darker-brown\"\n    },\n    \"Item description\":\"Straight Fitting M5\",\n    \"Price per unit\":\"1.33\",\n    \"Image\":[\n      {\n        \"url\":\"http://localhost/media/user_files/Zv7h0kB5KKhKWky0H3PHyZQLJB1n8Z99_9309ddc96dedec59da725e14ca74acc95e98e5a36262b77648ca3188cbea6f6e.jpg\",\n        \"thumbnails\":{\n          \"tiny\":{\n            \"url\":\"http://localhost/media/thumbnails/tiny/Zv7h0kB5KKhKWky0H3PHyZQLJB1n8Z99_9309ddc96dedec59da725e14ca74acc95e98e5a36262b77648ca3188cbea6f6e.jpg\",\n            \"width\":null,\n            \"height\":21\n          },\n          \"small\":{\n            \"url\":\"http://localhost/media/thumbnails/small/Zv7h0kB5KKhKWky0H3PHyZQLJB1n8Z99_9309ddc96dedec59da725e14ca74acc95e98e5a36262b77648ca3188cbea6f6e.jpg\",\n            \"width\":48,\n            \"height\":48\n          },\n          \"card_cover\":{\n            \"url\":\"http://localhost/media/thumbnails/card_cover/Zv7h0kB5KKhKWky0H3PHyZQLJB1n8Z99_9309ddc96dedec59da725e14ca74acc95e98e5a36262b77648ca3188cbea6f6e.jpg\",\n            \"width\":300,\n            \"height\":160\n          }\n        },\n        \"visible_name\":\"LtvSOv4XvnJ3XiuAteI39jNUG1nJKE1...a36262b77648ca3188cbea6f6e.jpg\",\n        \"name\":\"Zv7h0kB5KKhKWky0H3PHyZQLJB1n8Z99_9309ddc96dedec59da725e14ca74acc95e98e5a36262b77648ca3188cbea6f6e.jpg\",\n        \"size\":65155,\n        \"mime_type\":\"image/jpeg\",\n        \"is_image\":true,\n        \"image_width\":768,\n        \"image_height\":768,\n        \"uploaded_at\":\"2025-05-04T14:45:03.166187+00:00\"\n      }\n    ],\n    \"Source\":\"\",\n    \"Order Items\":[],\n    \"Datasheet\":[],\n    \"Part of a set\":[],\n    \"State\":{\n      \"id\":3002,\n      \"value\":\"Production & Used\",\n      \"color\":\"darker-green\"\n    },\n    \"Part Number\":\"20-00007\",\n    \"Revision\":\"A\",\n    \"Notes\":null,\n    \"Sourced By\":null,\n    \"Containing\":[],\n    \"Contained by\":[]\n  },\n  {\n    \"id\":69,\n    \"order\":\"14.00000000000000000000\",\n    \"Full PN\":\"20-00008 Rev.A\",\n    \"External Part Number\":\"PC4-01M\",\n    \"Manufacturer\":[\n      {\n        \"id\":6,\n        \"value\":\"Pisco\",\n        \"order\":\"6.00000000000000000000\"\n      }\n    ],\n    \"System\":{\n      \"id\":2966,\n      \"value\":\"Gas supply\",\n      \"color\":\"darker-brown\"\n    },\n    \"Item description\":\"Straight Fitting 1/8\\\"\",\n    \"Price per unit\":\"1.05\",\n    \"Image\":[\n      {\n        \"url\":\"http://localhost/media/user_files/Zv7h0kB5KKhKWky0H3PHyZQLJB1n8Z99_9309ddc96dedec59da725e14ca74acc95e98e5a36262b77648ca3188cbea6f6e.jpg\",\n        \"thumbnails\":{\n          \"tiny\":{\n            \"url\":\"http://localhost/media/thumbnails/tiny/Zv7h0kB5KKhKWky0H3PHyZQLJB1n8Z99_9309ddc96dedec59da725e14ca74acc95e98e5a36262b77648ca3188cbea6f6e.jpg\",\n            \"width\":null,\n            \"height\":21\n          },\n          \"small\":{\n            \"url\":\"http://localhost/media/thumbnails/small/Zv7h0kB5KKhKWky0H3PHyZQLJB1n8Z99_9309ddc96dedec59da725e14ca74acc95e98e5a36262b77648ca3188cbea6f6e.jpg\",\n            \"width\":48,\n            \"height\":48\n          },\n          \"card_cover\":{\n            \"url\":\"http://localhost/media/thumbnails/card_cover/Zv7h0kB5KKhKWky0H3PHyZQLJB1n8Z99_9309ddc96dedec59da725e14ca74acc95e98e5a36262b77648ca3188cbea6f6e.jpg\",\n            \"width\":300,\n            \"height\":160\n          }\n        },\n        \"visible_name\":\"LtvSOv4XvnJ3XiuAteI39jNUG1nJKE1...a36262b77648ca3188cbea6f6e.jpg\",\n        \"name\":\"Zv7h0kB5KKhKWky0H3PHyZQLJB1n8Z99_9309ddc96dedec59da725e14ca74acc95e98e5a36262b77648ca3188cbea6f6e.jpg\",\n        \"size\":65155,\n        \"mime_type\":\"image/jpeg\",\n        \"is_image\":true,\n        \"image_width\":768,\n        \"image_height\":768,\n        \"uploaded_at\":\"2025-05-04T14:45:03.166187+00:00\"\n      }\n    ],\n    \"Source\":\"https://www.conlog.co.il/pisco/\",\n    \"Order Items\":[\n      {\n        \"id\":12,\n        \"value\":\"b9ae33d0-c356-41b4-ad98-58e00620cdd5\",\n        \"order\":\"10.00000000000000000000\"\n      }\n    ],\n    \"Datasheet\":[],\n    \"Part of a set\":[],\n    \"State\":{\n      \"id\":3001,\n      \"value\":\"Unknown\",\n      \"color\":\"dark-orange\"\n    },\n    \"Part Number\":\"20-00008\",\n    \"Revision\":\"A\",\n    \"Notes\":null,\n    \"Sourced By\":null,\n    \"Containing\":[],\n    \"Contained by\":[]\n  },\n  {\n    \"id\":70,\n    \"order\":\"15.00000000000000000000\",\n    \"Full PN\":\"20-00009 Rev.A\",\n    \"External Part Number\":\"PL4-M6M\",\n    \"Manufacturer\":[\n      {\n        \"id\":6,\n        \"value\":\"Pisco\",\n        \"order\":\"6.00000000000000000000\"\n      }\n    ],\n    \"System\":{\n      \"id\":2966,\n      \"value\":\"Gas supply\",\n      \"color\":\"darker-brown\"\n    },\n    \"Item description\":\"Elbow Fitting\",\n    \"Price per unit\":null,\n    \"Image\":[\n      {\n        \"url\":\"http://localhost/media/user_files/bO8U2MHvSWluVp6JKOM11SakLzF0VktS_b377f4e44014f155d52983b2813253a6bedd0bd1a78d4001d422339f4dc3835e.jpg\",\n        \"thumbnails\":{\n          \"tiny\":{\n            \"url\":\"http://localhost/media/thumbnails/tiny/bO8U2MHvSWluVp6JKOM11SakLzF0VktS_b377f4e44014f155d52983b2813253a6bedd0bd1a78d4001d422339f4dc3835e.jpg\",\n            \"width\":null,\n            \"height\":21\n          },\n          \"small\":{\n            \"url\":\"http://localhost/media/thumbnails/small/bO8U2MHvSWluVp6JKOM11SakLzF0VktS_b377f4e44014f155d52983b2813253a6bedd0bd1a78d4001d422339f4dc3835e.jpg\",\n            \"width\":48,\n            \"height\":48\n          },\n          \"card_cover\":{\n            \"url\":\"http://localhost/media/thumbnails/card_cover/bO8U2MHvSWluVp6JKOM11SakLzF0VktS_b377f4e44014f155d52983b2813253a6bedd0bd1a78d4001d422339f4dc3835e.jpg\",\n            \"width\":300,\n            \"height\":160\n          }\n        },\n        \"visible_name\":\"lVhAuvaaN2wSqESE9vW6hTyExEgLUS0...d1a78d4001d422339f4dc3835e.jpg\",\n        \"name\":\"bO8U2MHvSWluVp6JKOM11SakLzF0VktS_b377f4e44014f155d52983b2813253a6bedd0bd1a78d4001d422339f4dc3835e.jpg\",\n        \"size\":71988,\n        \"mime_type\":\"image/jpeg\",\n        \"is_image\":true,\n        \"image_width\":768,\n        \"image_height\":768,\n        \"uploaded_at\":\"2025-05-04T14:45:13.916154+00:00\"\n      }\n    ],\n    \"Source\":\"https://www.conlog.co.il/pisco/\",\n    \"Order Items\":[],\n    \"Datasheet\":[],\n    \"Part of a set\":[],\n    \"State\":{\n      \"id\":3002,\n      \"value\":\"Production & Used\",\n      \"color\":\"darker-green\"\n    },\n    \"Part Number\":\"20-00009\",\n    \"Revision\":\"A\",\n    \"Notes\":null,\n    \"Sourced By\":null,\n    \"Containing\":[],\n    \"Contained by\":[]\n  },\n  {\n    \"id\":71,\n    \"order\":\"16.00000000000000000000\",\n    \"Full PN\":\"20-00010 Rev.A\",\n    \"External Part Number\":\"PML4\",\n    \"Manufacturer\":[\n      {\n        \"id\":6,\n        \"value\":\"Pisco\",\n        \"order\":\"6.00000000000000000000\"\n      }\n    ],\n    \"System\":{\n      \"id\":2966,\n      \"value\":\"Gas supply\",\n      \"color\":\"darker-brown\"\n    },\n    \"Item description\":\"Bulkhead Union Elbow\",\n    \"Price per unit\":\"2.95\",\n    \"Image\":[\n      {\n        \"url\":\"http://localhost/media/user_files/lHUcxxfYUYcOKvDWhmyyR4uhcV11PER7_e6feb76d2cfc05650132bc8ee7d9cd88ef38a73993dd5498a4522857ca901533.png\",\n        \"thumbnails\":{\n          \"tiny\":{\n            \"url\":\"http://localhost/media/thumbnails/tiny/lHUcxxfYUYcOKvDWhmyyR4uhcV11PER7_e6feb76d2cfc05650132bc8ee7d9cd88ef38a73993dd5498a4522857ca901533.png\",\n            \"width\":null,\n            \"height\":21\n          },\n          \"small\":{\n            \"url\":\"http://localhost/media/thumbnails/small/lHUcxxfYUYcOKvDWhmyyR4uhcV11PER7_e6feb76d2cfc05650132bc8ee7d9cd88ef38a73993dd5498a4522857ca901533.png\",\n            \"width\":48,\n            \"height\":48\n          },\n          \"card_cover\":{\n            \"url\":\"http://localhost/media/thumbnails/card_cover/lHUcxxfYUYcOKvDWhmyyR4uhcV11PER7_e6feb76d2cfc05650132bc8ee7d9cd88ef38a73993dd5498a4522857ca901533.png\",\n            \"width\":300,\n            \"height\":160\n          }\n        },\n        \"visible_name\":\"image.png\",\n        \"name\":\"lHUcxxfYUYcOKvDWhmyyR4uhcV11PER7_e6feb76d2cfc05650132bc8ee7d9cd88ef38a73993dd5498a4522857ca901533.png\",\n        \"size\":353161,\n        \"mime_type\":\"image/png\",\n        \"is_image\":true,\n        \"image_width\":768,\n        \"image_height\":768,\n        \"uploaded_at\":\"2025-05-11T10:08:09.284107+00:00\"\n      }\n    ],\n    \"Source\":\"https://www.conlog.co.il/pisco/\",\n    \"Order Items\":[\n      {\n        \"id\":13,\n        \"value\":\"4355c0fa-c579-4d59-a138-8f60a6995b23\",\n        \"order\":\"11.00000000000000000000\"\n      }\n    ],\n    \"Datasheet\":[],\n    \"Part of a set\":[],\n    \"State\":{\n      \"id\":3001,\n      \"value\":\"Unknown\",\n      \"color\":\"dark-orange\"\n    },\n    \"Part Number\":\"20-00010\",\n    \"Revision\":\"A\",\n    \"Notes\":null,\n    \"Sourced By\":null,\n    \"Containing\":[],\n    \"Contained by\":[]\n  },\n  {\n    \"id\":72,\n    \"order\":\"17.00000000000000000000\",\n    \"Full PN\":\"20-00011 Rev.A\",\n    \"External Part Number\":\"PLJ4M\",\n    \"Manufacturer\":[\n      {\n        \"id\":6,\n        \"value\":\"Pisco\",\n        \"order\":\"6.00000000000000000000\"\n      }\n    ],\n    \"System\":{\n      \"id\":2966,\n      \"value\":\"Gas supply\",\n      \"color\":\"darker-brown\"\n    },\n    \"Item description\":\"Plug-in Elbow\",\n    \"Price per unit\":\"1.47\",\n    \"Image\":[\n      {\n        \"url\":\"http://localhost/media/user_files/31DmbNws9U3eVgrNsfB1BTZBnLl6Jt3o_e3889edc2ff59571da4e5a5823c3f01ccd6dff270370fe4022895388b9dfd390.jpg\",\n        \"thumbnails\":{\n          \"tiny\":{\n            \"url\":\"http://localhost/media/thumbnails/tiny/31DmbNws9U3eVgrNsfB1BTZBnLl6Jt3o_e3889edc2ff59571da4e5a5823c3f01ccd6dff270370fe4022895388b9dfd390.jpg\",\n            \"width\":null,\n            \"height\":21\n          },\n          \"small\":{\n            \"url\":\"http://localhost/media/thumbnails/small/31DmbNws9U3eVgrNsfB1BTZBnLl6Jt3o_e3889edc2ff59571da4e5a5823c3f01ccd6dff270370fe4022895388b9dfd390.jpg\",\n            \"width\":48,\n            \"height\":48\n          },\n          \"card_cover\":{\n            \"url\":\"http://localhost/media/thumbnails/card_cover/31DmbNws9U3eVgrNsfB1BTZBnLl6Jt3o_e3889edc2ff59571da4e5a5823c3f01ccd6dff270370fe4022895388b9dfd390.jpg\",\n            \"width\":300,\n            \"height\":160\n          }\n        },\n        \"visible_name\":\"kX7jHKKvLz7kX0kWmItB2MRWsASLFih...270370fe4022895388b9dfd390.jpg\",\n        \"name\":\"31DmbNws9U3eVgrNsfB1BTZBnLl6Jt3o_e3889edc2ff59571da4e5a5823c3f01ccd6dff270370fe4022895388b9dfd390.jpg\",\n        \"size\":46270,\n        \"mime_type\":\"image/jpeg\",\n        \"is_image\":true,\n        \"image_width\":768,\n        \"image_height\":768,\n        \"uploaded_at\":\"2025-05-04T14:46:18.078725+00:00\"\n      }\n    ],\n    \"Source\":\"https://www.conlog.co.il/pisco/\",\n    \"Order Items\":[\n      {\n        \"id\":14,\n        \"value\":\"1e903c1b-479d-4931-8050-c251507ccecf\",\n        \"order\":\"12.00000000000000000000\"\n      }\n    ],\n    \"Datasheet\":[],\n    \"Part of a set\":[],\n    \"State\":{\n      \"id\":3002,\n      \"value\":\"Production & Used\",\n      \"color\":\"darker-green\"\n    },\n    \"Part Number\":\"20-00011\",\n    \"Revision\":\"A\",\n    \"Notes\":null,\n    \"Sourced By\":null,\n    \"Containing\":[],\n    \"Contained by\":[]\n  },\n  {\n    \"id\":73,\n    \"order\":\"18.00000000000000000000\",\n    \"Full PN\":\"40-00007 Rev.A\",\n    \"External Part Number\":\"KP43P-030-F1\",\n    \"Manufacturer\":[\n      {\n        \"id\":8,\n        \"value\":\"Kita\",\n        \"order\":\"8.00000000000000000000\"\n      }\n    ],\n    \"System\":{\n      \"id\":2966,\n      \"value\":\"Gas supply\",\n      \"color\":\"darker-brown\"\n    },\n    \"Item description\":\"Electronic pressure gauge (R1/8\\\" or M5 thread, PNP + 1v~5v output)\",\n    \"Price per unit\":\"39.00\",\n    \"Image\":[\n      {\n        \"url\":\"http://localhost/media/user_files/Ytrsu9SIBU6Yy3yx86ldD9PEGmiLfTgV_77db93f3110563fc330a2ec70130aa94bdbaeb8579d8575764ab6fd001926dde.webp\",\n        \"thumbnails\":{\n          \"tiny\":{\n            \"url\":\"http://localhost/media/thumbnails/tiny/Ytrsu9SIBU6Yy3yx86ldD9PEGmiLfTgV_77db93f3110563fc330a2ec70130aa94bdbaeb8579d8575764ab6fd001926dde.webp\",\n            \"width\":null,\n            \"height\":21\n          },\n          \"small\":{\n            \"url\":\"http://localhost/media/thumbnails/small/Ytrsu9SIBU6Yy3yx86ldD9PEGmiLfTgV_77db93f3110563fc330a2ec70130aa94bdbaeb8579d8575764ab6fd001926dde.webp\",\n            \"width\":48,\n            \"height\":48\n          },\n          \"card_cover\":{\n            \"url\":\"http://localhost/media/thumbnails/card_cover/Ytrsu9SIBU6Yy3yx86ldD9PEGmiLfTgV_77db93f3110563fc330a2ec70130aa94bdbaeb8579d8575764ab6fd001926dde.webp\",\n            \"width\":300,\n            \"height\":160\n          }\n        },\n        \"visible_name\":\"ehW3H4PECOm4Jmdhk82JgFl6KYn5Yx7...579d8575764ab6fd001926dde.webp\",\n        \"name\":\"Ytrsu9SIBU6Yy3yx86ldD9PEGmiLfTgV_77db93f3110563fc330a2ec70130aa94bdbaeb8579d8575764ab6fd001926dde.webp\",\n        \"size\":11728,\n        \"mime_type\":\"image/webp\",\n        \"is_image\":true,\n        \"image_width\":515,\n        \"image_height\":303,\n        \"uploaded_at\":\"2025-05-04T14:50:31.097919+00:00\"\n      }\n    ],\n    \"Source\":\"https://www.conlog.co.il/kita-sensor-tech/\",\n    \"Order Items\":[\n      {\n        \"id\":15,\n        \"value\":\"d8c27e36-8f10-452d-b8fb-41abeb87284a\",\n        \"order\":\"13.00000000000000000000\"\n      }\n    ],\n    \"Datasheet\":[\n      {\n        \"url\":\"http://localhost/media/user_files/z58VjyTRNDXL3p9D0P7RHxZBbcXRJUc6_49661d864c4038f4b67a4e350ecf9f2d03aebfa4dd057b0664d1dfdbdf01ccd9.pdf\",\n        \"thumbnails\":null,\n        \"visible_name\":\"KP43+Catalog.pdf\",\n        \"name\":\"z58VjyTRNDXL3p9D0P7RHxZBbcXRJUc6_49661d864c4038f4b67a4e350ecf9f2d03aebfa4dd057b0664d1dfdbdf01ccd9.pdf\",\n        \"size\":487545,\n        \"mime_type\":\"application/pdf\",\n        \"is_image\":false,\n        \"image_width\":null,\n        \"image_height\":null,\n        \"uploaded_at\":\"2025-09-09T08:59:37.612163+00:00\"\n      }\n    ],\n    \"Part of a set\":[],\n    \"State\":{\n      \"id\":3001,\n      \"value\":\"Unknown\",\n      \"color\":\"dark-orange\"\n    },\n    \"Part Number\":\"40-00007\",\n    \"Revision\":\"A\",\n    \"Notes\":null,\n    \"Sourced By\":null,\n    \"Containing\":[],\n    \"Contained by\":[]\n  },\n  {\n    \"id\":74,\n    \"order\":\"19.00000000000000000000\",\n    \"Full PN\":\"20-00012 Rev.A\",\n    \"External Part Number\":\"PB4-01M\",\n    \"Manufacturer\":[\n      {\n        \"id\":6,\n        \"value\":\"Pisco\",\n        \"order\":\"6.00000000000000000000\"\n      }\n    ],\n    \"System\":{\n      \"id\":2966,\n      \"value\":\"Gas supply\",\n      \"color\":\"darker-brown\"\n    },\n    \"Item description\":\"Branch Tee with r1/8 male thread tail\",\n    \"Price per unit\":null,\n    \"Image\":[\n      {\n        \"url\":\"http://localhost/media/user_files/YkXq3jS38CHXYj1xSmYTYMUzvAKG4lFY_b9b6dd2db76c81dec8780a6b323401cfabf073d010a67408ad9abba35b957c01.png\",\n        \"thumbnails\":{\n          \"tiny\":{\n            \"url\":\"http://localhost/media/thumbnails/tiny/YkXq3jS38CHXYj1xSmYTYMUzvAKG4lFY_b9b6dd2db76c81dec8780a6b323401cfabf073d010a67408ad9abba35b957c01.png\",\n            \"width\":null,\n            \"height\":21\n          },\n          \"small\":{\n            \"url\":\"http://localhost/media/thumbnails/small/YkXq3jS38CHXYj1xSmYTYMUzvAKG4lFY_b9b6dd2db76c81dec8780a6b323401cfabf073d010a67408ad9abba35b957c01.png\",\n            \"width\":48,\n            \"height\":48\n          },\n          \"card_cover\":{\n            \"url\":\"http://localhost/media/thumbnails/card_cover/YkXq3jS38CHXYj1xSmYTYMUzvAKG4lFY_b9b6dd2db76c81dec8780a6b323401cfabf073d010a67408ad9abba35b957c01.png\",\n            \"width\":300,\n            \"height\":160\n          }\n        },\n        \"visible_name\":\"image.png\",\n        \"name\":\"YkXq3jS38CHXYj1xSmYTYMUzvAKG4lFY_b9b6dd2db76c81dec8780a6b323401cfabf073d010a67408ad9abba35b957c01.png\",\n        \"size\":539319,\n        \"mime_type\":\"image/png\",\n        \"is_image\":true,\n        \"image_width\":768,\n        \"image_height\":768,\n        \"uploaded_at\":\"2025-05-11T10:07:00.275994+00:00\"\n      }\n    ],\n    \"Source\":\"https://www.conlog.co.il/pisco/\",\n    \"Order Items\":[],\n    \"Datasheet\":[],\n    \"Part of a set\":[],\n    \"State\":{\n      \"id\":3002,\n      \"value\":\"Production & Used\",\n      \"color\":\"darker-green\"\n    },\n    \"Part Number\":\"20-00012\",\n    \"Revision\":\"A\",\n    \"Notes\":null,\n    \"Sourced By\":null,\n    \"Containing\":[],\n    \"Contained by\":[]\n  },\n  {\n    \"id\":75,\n    \"order\":\"20.00000000000000000000\",\n    \"Full PN\":\"20-00013 Rev.A\",\n    \"External Part Number\":\"04050 00 01 02 NB\",\n    \"Manufacturer\":[\n      {\n        \"id\":9,\n        \"value\":\"Aignep\",\n        \"order\":\"9.00000000000000000000\"\n      }\n    ],\n    \"System\":{\n      \"id\":2966,\n      \"value\":\"Gas supply\",\n      \"color\":\"darker-brown\"\n    },\n    \"Item description\":\"Off set male tee (MFF 1/8\\\")\",\n    \"Price per unit\":\"1.10\",\n    \"Image\":[\n      {\n        \"url\":\"http://localhost/media/user_files/lmrXolSKFr5cscXQZ5MpgGLI6KBFOmMF_e1c0518c28b31d63a52f4ff7f36dda38ddd09aabcf233b2335824103e8f65df2.jpg\",\n        \"thumbnails\":{\n          \"tiny\":{\n            \"url\":\"http://localhost/media/thumbnails/tiny/lmrXolSKFr5cscXQZ5MpgGLI6KBFOmMF_e1c0518c28b31d63a52f4ff7f36dda38ddd09aabcf233b2335824103e8f65df2.jpg\",\n            \"width\":null,\n            \"height\":21\n          },\n          \"small\":{\n            \"url\":\"http://localhost/media/thumbnails/small/lmrXolSKFr5cscXQZ5MpgGLI6KBFOmMF_e1c0518c28b31d63a52f4ff7f36dda38ddd09aabcf233b2335824103e8f65df2.jpg\",\n            \"width\":48,\n            \"height\":48\n          },\n          \"card_cover\":{\n            \"url\":\"http://localhost/media/thumbnails/card_cover/lmrXolSKFr5cscXQZ5MpgGLI6KBFOmMF_e1c0518c28b31d63a52f4ff7f36dda38ddd09aabcf233b2335824103e8f65df2.jpg\",\n            \"width\":300,\n            \"height\":160\n          }\n        },\n        \"visible_name\":\"hpA1mO6bBHopKOgs6FH1fTzSbpnkqDU...abcf233b2335824103e8f65df2.jpg\",\n        \"name\":\"lmrXolSKFr5cscXQZ5MpgGLI6KBFOmMF_e1c0518c28b31d63a52f4ff7f36dda38ddd09aabcf233b2335824103e8f65df2.jpg\",\n        \"size\":7735,\n        \"mime_type\":\"image/jpeg\",\n        \"is_image\":true,\n        \"image_width\":375,\n        \"image_height\":243,\n        \"uploaded_at\":\"2025-05-04T14:51:08.268754+00:00\"\n      },\n      {\n        \"url\":\"http://localhost/media/user_files/bzpSBAPvaIzsaWOqCU6cudkliE6ZDaxX_0e55e8f3dd2ef41333436613d9fdfce56de95c22c4d55736d4bfd285d163d46b.jpg\",\n        \"thumbnails\":{\n          \"tiny\":{\n            \"url\":\"http://localhost/media/thumbnails/tiny/bzpSBAPvaIzsaWOqCU6cudkliE6ZDaxX_0e55e8f3dd2ef41333436613d9fdfce56de95c22c4d55736d4bfd285d163d46b.jpg\",\n            \"width\":null,\n            \"height\":21\n          },\n          \"small\":{\n            \"url\":\"http://localhost/media/thumbnails/small/bzpSBAPvaIzsaWOqCU6cudkliE6ZDaxX_0e55e8f3dd2ef41333436613d9fdfce56de95c22c4d55736d4bfd285d163d46b.jpg\",\n            \"width\":48,\n            \"height\":48\n          },\n          \"card_cover\":{\n            \"url\":\"http://localhost/media/thumbnails/card_cover/bzpSBAPvaIzsaWOqCU6cudkliE6ZDaxX_0e55e8f3dd2ef41333436613d9fdfce56de95c22c4d55736d4bfd285d163d46b.jpg\",\n            \"width\":300,\n            \"height\":160\n          }\n        },\n        \"visible_name\":\"Aignep-04050000102NB-image.jpg\",\n        \"name\":\"bzpSBAPvaIzsaWOqCU6cudkliE6ZDaxX_0e55e8f3dd2ef41333436613d9fdfce56de95c22c4d55736d4bfd285d163d46b.jpg\",\n        \"size\":16260,\n        \"mime_type\":\"image/jpeg\",\n        \"is_image\":true,\n        \"image_width\":444,\n        \"image_height\":372,\n        \"uploaded_at\":\"2025-05-12T07:55:06.184150+00:00\"\n      }\n    ],\n    \"Source\":\"https://www.conlog.co.il/aignep/\",\n    \"Order Items\":[\n      {\n        \"id\":16,\n        \"value\":\"fc36026a-a828-4504-ae88-e0ef256fed5c\",\n        \"order\":\"14.00000000000000000000\"\n      }\n    ],\n    \"Datasheet\":[],\n    \"Part of a set\":[],\n    \"State\":{\n      \"id\":3002,\n      \"value\":\"Production & Used\",\n      \"color\":\"darker-green\"\n    },\n    \"Part Number\":\"20-00013\",\n    \"Revision\":\"A\",\n    \"Notes\":null,\n    \"Sourced By\":null,\n    \"Containing\":[],\n    \"Contained by\":[]\n  },\n  {\n    \"id\":76,\n    \"order\":\"21.00000000000000000000\",\n    \"Full PN\":\"20-00014 Rev.A\",\n    \"External Part Number\":\"04000 00 01 02 NB\",\n    \"Manufacturer\":[\n      {\n        \"id\":9,\n        \"value\":\"Aignep\",\n        \"order\":\"9.00000000000000000000\"\n      }\n    ],\n    \"System\":{\n      \"id\":2966,\n      \"value\":\"Gas supply\",\n      \"color\":\"darker-brown\"\n    },\n    \"Item description\":\"Female tee (FFF 1/8\\\")\",\n    \"Price per unit\":\"1.25\",\n    \"Image\":[\n      {\n        \"url\":\"http://localhost/media/user_files/VSaRYEZUhx7Tu5SkamOZsGm1VwmkIaTN_909788723c0ea56f0143d0ac4ad7e21892fb60d5c619c106a3dc19d8b79a94be.jpg\",\n        \"thumbnails\":{\n          \"tiny\":{\n            \"url\":\"http://localhost/media/thumbnails/tiny/VSaRYEZUhx7Tu5SkamOZsGm1VwmkIaTN_909788723c0ea56f0143d0ac4ad7e21892fb60d5c619c106a3dc19d8b79a94be.jpg\",\n            \"width\":null,\n            \"height\":21\n          },\n          \"small\":{\n            \"url\":\"http://localhost/media/thumbnails/small/VSaRYEZUhx7Tu5SkamOZsGm1VwmkIaTN_909788723c0ea56f0143d0ac4ad7e21892fb60d5c619c106a3dc19d8b79a94be.jpg\",\n            \"width\":48,\n            \"height\":48\n          },\n          \"card_cover\":{\n            \"url\":\"http://localhost/media/thumbnails/card_cover/VSaRYEZUhx7Tu5SkamOZsGm1VwmkIaTN_909788723c0ea56f0143d0ac4ad7e21892fb60d5c619c106a3dc19d8b79a94be.jpg\",\n            \"width\":300,\n            \"height\":160\n          }\n        },\n        \"visible_name\":\"Aignep-04000000102NB-image.jpg\",\n        \"name\":\"VSaRYEZUhx7Tu5SkamOZsGm1VwmkIaTN_909788723c0ea56f0143d0ac4ad7e21892fb60d5c619c106a3dc19d8b79a94be.jpg\",\n        \"size\":17064,\n        \"mime_type\":\"image/jpeg\",\n        \"is_image\":true,\n        \"image_width\":444,\n        \"image_height\":357,\n        \"uploaded_at\":\"2025-05-12T07:55:12.069450+00:00\"\n      }\n    ],\n    \"Source\":\"https://www.conlog.co.il/aignep/\",\n    \"Order Items\":[\n      {\n        \"id\":17,\n        \"value\":\"e70c65d6-975e-4434-9150-1fcc38942b28\",\n        \"order\":\"15.00000000000000000000\"\n      }\n    ],\n    \"Datasheet\":[],\n    \"Part of a set\":[],\n    \"State\":{\n      \"id\":3004,\n      \"value\":\"Not Used\",\n      \"color\":\"darker-red\"\n    },\n    \"Part Number\":\"20-00014\",\n    \"Revision\":\"A\",\n    \"Notes\":null,\n    \"Sourced By\":null,\n    \"Containing\":[],\n    \"Contained by\":[]\n  },\n  {\n    \"id\":77,\n    \"order\":\"22.00000000000000000000\",\n    \"Full PN\":\"20-00015 Rev.A\",\n    \"External Part Number\":\"01F 02 1 25 N0\",\n    \"Manufacturer\":[\n      {\n        \"id\":9,\n        \"value\":\"Aignep\",\n        \"order\":\"9.00000000000000000000\"\n      }\n    ],\n    \"System\":{\n      \"id\":2966,\n      \"value\":\"Gas supply\",\n      \"color\":\"darker-brown\"\n    },\n    \"Item description\":\"Solenoid Valve 2.5mm\",\n    \"Price per unit\":\"20.47\",\n    \"Image\":[],\n    \"Source\":\"https://www.conlog.co.il/aignep/\",\n    \"Order Items\":[\n      {\n        \"id\":18,\n        \"value\":\"75409d4b-c7c8-4272-874a-e2d7151c5300\",\n        \"order\":\"16.00000000000000000000\"\n      }\n    ],\n    \"Datasheet\":[],\n    \"Part of a set\":[],\n    \"State\":{\n      \"id\":3001,\n      \"value\":\"Unknown\",\n      \"color\":\"dark-orange\"\n    },\n    \"Part Number\":\"20-00015\",\n    \"Revision\":\"A\",\n    \"Notes\":null,\n    \"Sourced By\":null,\n    \"Containing\":[],\n    \"Contained by\":[]\n  },\n  {\n    \"id\":78,\n    \"order\":\"23.00000000000000000000\",\n    \"Full PN\":\"40-00008 Rev.A\",\n    \"External Part Number\":\"SOL10024C4000\",\n    \"Manufacturer\":[\n      {\n        \"id\":9,\n        \"value\":\"Aignep\",\n        \"order\":\"9.00000000000000000000\"\n      }\n    ],\n    \"System\":{\n      \"id\":2966,\n      \"value\":\"Gas supply\",\n      \"color\":\"darker-brown\"\n    },\n    \"Item description\":\"Solenoid Valve Coil 24v\",\n    \"Price per unit\":\"7.39\",\n    \"Image\":[\n      {\n        \"url\":\"http://localhost/media/user_files/cglmT3ontEC2BVvQqWLn59i5PEd7KITB_2178aa74bf7670e98a9fc782a13458d9d8748ba1d9ecd969f53c8f9968b10c20.jpg\",\n        \"thumbnails\":{\n          \"tiny\":{\n            \"url\":\"http://localhost/media/thumbnails/tiny/cglmT3ontEC2BVvQqWLn59i5PEd7KITB_2178aa74bf7670e98a9fc782a13458d9d8748ba1d9ecd969f53c8f9968b10c20.jpg\",\n            \"width\":null,\n            \"height\":21\n          },\n          \"small\":{\n            \"url\":\"http://localhost/media/thumbnails/small/cglmT3ontEC2BVvQqWLn59i5PEd7KITB_2178aa74bf7670e98a9fc782a13458d9d8748ba1d9ecd969f53c8f9968b10c20.jpg\",\n            \"width\":48,\n            \"height\":48\n          },\n          \"card_cover\":{\n            \"url\":\"http://localhost/media/thumbnails/card_cover/cglmT3ontEC2BVvQqWLn59i5PEd7KITB_2178aa74bf7670e98a9fc782a13458d9d8748ba1d9ecd969f53c8f9968b10c20.jpg\",\n            \"width\":300,\n            \"height\":160\n          }\n        },\n        \"visible_name\":\"Aignep-SOL10024C4000-image.jpg\",\n        \"name\":\"cglmT3ontEC2BVvQqWLn59i5PEd7KITB_2178aa74bf7670e98a9fc782a13458d9d8748ba1d9ecd969f53c8f9968b10c20.jpg\",\n        \"size\":18402,\n        \"mime_type\":\"image/jpeg\",\n        \"is_image\":true,\n        \"image_width\":322,\n        \"image_height\":444,\n        \"uploaded_at\":\"2025-05-12T07:55:49.240482+00:00\"\n      }\n    ],\n    \"Source\":\"https://www.conlog.co.il/aignep/\",\n    \"Order Items\":[\n      {\n        \"id\":19,\n        \"value\":\"e999bae5-1815-43ea-ae80-3ee181411b02\",\n        \"order\":\"17.00000000000000000000\"\n      }\n    ],\n    \"Datasheet\":[],\n    \"Part of a set\":[],\n    \"State\":{\n      \"id\":3001,\n      \"value\":\"Unknown\",\n      \"color\":\"dark-orange\"\n    },\n    \"Part Number\":\"40-00008\",\n    \"Revision\":\"A\",\n    \"Notes\":null,\n    \"Sourced By\":null,\n    \"Containing\":[],\n    \"Contained by\":[]\n  },\n  {\n    \"id\":79,\n    \"order\":\"24.00000000000000000000\",\n    \"Full PN\":\"40-00009 Rev.A\",\n    \"External Part Number\":\"CON02 024 00\",\n    \"Manufacturer\":[\n      {\n        \"id\":9,\n        \"value\":\"Aignep\",\n        \"order\":\"9.00000000000000000000\"\n      }\n    ],\n    \"System\":{\n      \"id\":2966,\n      \"value\":\"Gas supply\",\n      \"color\":\"darker-brown\"\n    },\n    \"Item description\":\"Solenoid terminals cover with LED\",\n    \"Price per unit\":\"6.25\",\n    \"Image\":[],\n    \"Source\":\"https://www.conlog.co.il/aignep/\",\n    \"Order Items\":[\n      {\n        \"id\":20,\n        \"value\":\"0dea69a4-39a9-4c0c-b85f-317e66b85b0e\",\n        \"order\":\"18.00000000000000000000\"\n      }\n    ],\n    \"Datasheet\":[],\n    \"Part of a set\":[],\n    \"State\":{\n      \"id\":3002,\n      \"value\":\"Production & Used\",\n      \"color\":\"darker-green\"\n    },\n    \"Part Number\":\"40-00009\",\n    \"Revision\":\"A\",\n    \"Notes\":null,\n    \"Sourced By\":null,\n    \"Containing\":[],\n    \"Contained by\":[]\n  },\n  {\n    \"id\":80,\n    \"order\":\"25.00000000000000000000\",\n    \"Full PN\":\"40-00010 Rev.A\",\n    \"External Part Number\":\"CON02 000 01\",\n    \"Manufacturer\":[\n      {\n        \"id\":9,\n        \"value\":\"Aignep\",\n        \"order\":\"9.00000000000000000000\"\n      }\n    ],\n    \"System\":{\n      \"id\":2966,\n      \"value\":\"Gas supply\",\n      \"color\":\"darker-brown\"\n    },\n    \"Item description\":\"Solenoid terminals cover\",\n    \"Price per unit\":null,\n    \"Image\":[],\n    \"Source\":\"https://www.conlog.co.il/aignep/\",\n    \"Order Items\":[],\n    \"Datasheet\":[],\n    \"Part of a set\":[],\n    \"State\":{\n      \"id\":3004,\n      \"value\":\"Not Used\",\n      \"color\":\"darker-red\"\n    },\n    \"Part Number\":\"40-00010\",\n    \"Revision\":\"A\",\n    \"Notes\":null,\n    \"Sourced By\":null,\n    \"Containing\":[],\n    \"Contained by\":[]\n  },\n  {\n    \"id\":81,\n    \"order\":\"26.00000000000000000000\",\n    \"Full PN\":\"20-00016 Rev.A\",\n    \"External Part Number\":\"111.12.40-10\",\n    \"Manufacturer\":[],\n    \"System\":{\n      \"id\":2966,\n      \"value\":\"Gas supply\",\n      \"color\":\"darker-brown\"\n    },\n    \"Item description\":\"Simple pressure gauge 10 bar 1/8\\\"\",\n    \"Price per unit\":\"13.65\",\n    \"Image\":[\n      {\n        \"url\":\"http://localhost/media/user_files/AoPGcRziSjFA46pH2r2ZdpLkZROG7g0A_f1d343ad61273ac0df18d1d30023bc13e8b25eb01df460f25c84088ea6259c8d.png\",\n        \"thumbnails\":{\n          \"tiny\":{\n            \"url\":\"http://localhost/media/thumbnails/tiny/AoPGcRziSjFA46pH2r2ZdpLkZROG7g0A_f1d343ad61273ac0df18d1d30023bc13e8b25eb01df460f25c84088ea6259c8d.png\",\n            \"width\":null,\n            \"height\":21\n          },\n          \"small\":{\n            \"url\":\"http://localhost/media/thumbnails/small/AoPGcRziSjFA46pH2r2ZdpLkZROG7g0A_f1d343ad61273ac0df18d1d30023bc13e8b25eb01df460f25c84088ea6259c8d.png\",\n            \"width\":48,\n            \"height\":48\n          },\n          \"card_cover\":{\n            \"url\":\"http://localhost/media/thumbnails/card_cover/AoPGcRziSjFA46pH2r2ZdpLkZROG7g0A_f1d343ad61273ac0df18d1d30023bc13e8b25eb01df460f25c84088ea6259c8d.png\",\n            \"width\":300,\n            \"height\":160\n          }\n        },\n        \"visible_name\":\"SjTJiRXxgPKHVJhUYq2G5Urg7IzqY3Q...b01df460f25c84088ea6259c8d.png\",\n        \"name\":\"AoPGcRziSjFA46pH2r2ZdpLkZROG7g0A_f1d343ad61273ac0df18d1d30023bc13e8b25eb01df460f25c84088ea6259c8d.png\",\n        \"size\":12534,\n        \"mime_type\":\"image/png\",\n        \"is_image\":true,\n        \"image_width\":103,\n        \"image_height\":92,\n        \"uploaded_at\":\"2025-05-04T14:46:38.288871+00:00\"\n      }\n    ],\n    \"Source\":\"https://www.conlog.co.il/aignep/\",\n    \"Order Items\":[\n      {\n        \"id\":22,\n        \"value\":\"44358639-80a0-4420-a170-4b5103a14f0e\",\n        \"order\":\"20.00000000000000000000\"\n      }\n    ],\n    \"Datasheet\":[],\n    \"Part of a set\":[],\n    \"State\":{\n      \"id\":3004,\n      \"value\":\"Not Used\",\n      \"color\":\"darker-red\"\n    },\n    \"Part Number\":\"20-00016\",\n    \"Revision\":\"A\",\n    \"Notes\":null,\n    \"Sourced By\":null,\n    \"Containing\":[],\n    \"Contained by\":[]\n  },\n  {\n    \"id\":82,\n    \"order\":\"27.00000000000000000000\",\n    \"Full PN\":\"20-00017 Rev.A\",\n    \"External Part Number\":\"111.12.40-4\",\n    \"Manufacturer\":[],\n    \"System\":{\n      \"id\":2966,\n      \"value\":\"Gas supply\",\n      \"color\":\"darker-brown\"\n    },\n    \"Item description\":\"Simple pressure gauge 4 bar 1/8\\\"\",\n    \"Price per unit\":\"13.65\",\n    \"Image\":[\n      {\n        \"url\":\"http://localhost/media/user_files/AoPGcRziSjFA46pH2r2ZdpLkZROG7g0A_f1d343ad61273ac0df18d1d30023bc13e8b25eb01df460f25c84088ea6259c8d.png\",\n        \"thumbnails\":{\n          \"tiny\":{\n            \"url\":\"http://localhost/media/thumbnails/tiny/AoPGcRziSjFA46pH2r2ZdpLkZROG7g0A_f1d343ad61273ac0df18d1d30023bc13e8b25eb01df460f25c84088ea6259c8d.png\",\n            \"width\":null,\n            \"height\":21\n          },\n          \"small\":{\n            \"url\":\"http://localhost/media/thumbnails/small/AoPGcRziSjFA46pH2r2ZdpLkZROG7g0A_f1d343ad61273ac0df18d1d30023bc13e8b25eb01df460f25c84088ea6259c8d.png\",\n            \"width\":48,\n            \"height\":48\n          },\n          \"card_cover\":{\n            \"url\":\"http://localhost/media/thumbnails/card_cover/AoPGcRziSjFA46pH2r2ZdpLkZROG7g0A_f1d343ad61273ac0df18d1d30023bc13e8b25eb01df460f25c84088ea6259c8d.png\",\n            \"width\":300,\n            \"height\":160\n          }\n        },\n        \"visible_name\":\"SjTJiRXxgPKHVJhUYq2G5Urg7IzqY3Q...b01df460f25c84088ea6259c8d.png\",\n        \"name\":\"AoPGcRziSjFA46pH2r2ZdpLkZROG7g0A_f1d343ad61273ac0df18d1d30023bc13e8b25eb01df460f25c84088ea6259c8d.png\",\n        \"size\":12534,\n        \"mime_type\":\"image/png\",\n        \"is_image\":true,\n        \"image_width\":103,\n        \"image_height\":92,\n        \"uploaded_at\":\"2025-05-04T14:46:38.288871+00:00\"\n      }\n    ],\n    \"Source\":\"https://www.conlog.co.il/aignep/\",\n    \"Order Items\":[\n      {\n        \"id\":23,\n        \"value\":\"7b9dfccd-e4fd-4ceb-b2ca-f615cd2064db\",\n        \"order\":\"21.00000000000000000000\"\n      }\n    ],\n    \"Datasheet\":[],\n    \"Part of a set\":[],\n    \"State\":{\n      \"id\":3004,\n      \"value\":\"Not Used\",\n      \"color\":\"darker-red\"\n    },\n    \"Part Number\":\"20-00017\",\n    \"Revision\":\"A\",\n    \"Notes\":null,\n    \"Sourced By\":null,\n    \"Containing\":[],\n    \"Contained by\":[]\n  },\n  {\n    \"id\":83,\n    \"order\":\"28.00000000000000000000\",\n    \"Full PN\":\"20-00018 Rev.A\",\n    \"External Part Number\":\"A14 - 3-7 bar - 1/8\\\"\",\n    \"Manufacturer\":[\n      {\n        \"id\":1,\n        \"value\":\"Nostrali\",\n        \"order\":\"1.00000000000000000000\"\n      }\n    ],\n    \"System\":{\n      \"id\":2966,\n      \"value\":\"Gas supply\",\n      \"color\":\"darker-brown\"\n    },\n    \"Item description\":\"Safety Valve 3bar ~ 7bar\",\n    \"Price per unit\":\"7.96\",\n    \"Image\":[],\n    \"Source\":\"https://www.conlog.co.il/\",\n    \"Order Items\":[\n      {\n        \"id\":24,\n        \"value\":\"375d9f3d-dd6a-4912-b759-397e9b373a87\",\n        \"order\":\"22.00000000000000000000\"\n      }\n    ],\n    \"Datasheet\":[],\n    \"Part of a set\":[],\n    \"State\":{\n      \"id\":3001,\n      \"value\":\"Unknown\",\n      \"color\":\"dark-orange\"\n    },\n    \"Part Number\":\"20-00018\",\n    \"Revision\":\"A\",\n    \"Notes\":null,\n    \"Sourced By\":null,\n    \"Containing\":[],\n    \"Contained by\":[]\n  },\n  {\n    \"id\":84,\n    \"order\":\"29.00000000000000000000\",\n    \"Full PN\":\"20-00019 Rev.A\",\n    \"External Part Number\":\"JNMU6\",\n    \"Manufacturer\":[\n      {\n        \"id\":6,\n        \"value\":\"Pisco\",\n        \"order\":\"6.00000000000000000000\"\n      }\n    ],\n    \"System\":{\n      \"id\":2966,\n      \"value\":\"Gas supply\",\n      \"color\":\"darker-brown\"\n    },\n    \"Item description\":\"Small Union Straight Throttle (Needle) Valve\",\n    \"Price per unit\":\"4.57\",\n    \"Image\":[\n      {\n        \"url\":\"http://localhost/media/user_files/CqhvkdMv1ydqwWtSZB6HT2ClLJxYWg1V_df4bbb22aa563bea1e684073dc0f97f996cfc454804fa13a4569133f3c5d7f50.png\",\n        \"thumbnails\":{\n          \"tiny\":{\n            \"url\":\"http://localhost/media/thumbnails/tiny/CqhvkdMv1ydqwWtSZB6HT2ClLJxYWg1V_df4bbb22aa563bea1e684073dc0f97f996cfc454804fa13a4569133f3c5d7f50.png\",\n            \"width\":null,\n            \"height\":21\n          },\n          \"small\":{\n            \"url\":\"http://localhost/media/thumbnails/small/CqhvkdMv1ydqwWtSZB6HT2ClLJxYWg1V_df4bbb22aa563bea1e684073dc0f97f996cfc454804fa13a4569133f3c5d7f50.png\",\n            \"width\":48,\n            \"height\":48\n          },\n          \"card_cover\":{\n            \"url\":\"http://localhost/media/thumbnails/card_cover/CqhvkdMv1ydqwWtSZB6HT2ClLJxYWg1V_df4bbb22aa563bea1e684073dc0f97f996cfc454804fa13a4569133f3c5d7f50.png\",\n            \"width\":300,\n            \"height\":160\n          }\n        },\n        \"visible_name\":\"image.png\",\n        \"name\":\"CqhvkdMv1ydqwWtSZB6HT2ClLJxYWg1V_df4bbb22aa563bea1e684073dc0f97f996cfc454804fa13a4569133f3c5d7f50.png\",\n        \"size\":16423,\n        \"mime_type\":\"image/png\",\n        \"is_image\":true,\n        \"image_width\":189,\n        \"image_height\":148,\n        \"uploaded_at\":\"2025-04-20T12:36:39.961423+00:00\"\n      }\n    ],\n    \"Source\":\"https://www.pisco.co.jp/media/pdf_en/b09-01.pdf\",\n    \"Order Items\":[\n      {\n        \"id\":25,\n        \"value\":\"7283c113-33af-44d2-a8d2-55cf2c30f9ec\",\n        \"order\":\"23.00000000000000000000\"\n      }\n    ],\n    \"Datasheet\":[\n      {\n        \"url\":\"http://localhost/media/user_files/HhPqR7Ufh3I9naJyUmoA0EVCiKeXYAbZ_e9da0d3523f5060d635560696f5003fd3d7d4b5e1646bcc0cb698ef25700aea4.pdf\",\n        \"thumbnails\":null,\n        \"visible_name\":\"JNMU.pdf\",\n        \"name\":\"HhPqR7Ufh3I9naJyUmoA0EVCiKeXYAbZ_e9da0d3523f5060d635560696f5003fd3d7d4b5e1646bcc0cb698ef25700aea4.pdf\",\n        \"size\":4927888,\n        \"mime_type\":\"application/pdf\",\n        \"is_image\":false,\n        \"image_width\":null,\n        \"image_height\":null,\n        \"uploaded_at\":\"2025-04-20T12:41:43.540787+00:00\"\n      }\n    ],\n    \"Part of a set\":[],\n    \"State\":{\n      \"id\":3002,\n      \"value\":\"Production & Used\",\n      \"color\":\"darker-green\"\n    },\n    \"Part Number\":\"20-00019\",\n    \"Revision\":\"A\",\n    \"Notes\":null,\n    \"Sourced By\":null,\n    \"Containing\":[],\n    \"Contained by\":[]\n  },\n  {\n    \"id\":85,\n    \"order\":\"30.00000000000000000000\",\n    \"Full PN\":\"40-00017 Rev.A\",\n    \"External Part Number\":\"MMBF 5486\",\n    \"Manufacturer\":[\n      {\n        \"id\":11,\n        \"value\":\"Onsemi\",\n        \"order\":\"11.00000000000000000000\"\n      }\n    ],\n    \"System\":{\n      \"id\":2967,\n      \"value\":\"Pre-amplifier\",\n      \"color\":\"dark-blue\"\n    },\n    \"Item description\":\"Q1 JFET\",\n    \"Price per unit\":null,\n    \"Image\":[\n      {\n        \"url\":\"http://localhost/media/user_files/cVPRnJU92oN82w9KxBTdfUwXtnrnmwps_24c65f362f804a7e6cbdc4a516fb1699a3b5ba31371eddd7ae367dd7b2a9862f.png\",\n        \"thumbnails\":{\n          \"tiny\":{\n            \"url\":\"http://localhost/media/thumbnails/tiny/cVPRnJU92oN82w9KxBTdfUwXtnrnmwps_24c65f362f804a7e6cbdc4a516fb1699a3b5ba31371eddd7ae367dd7b2a9862f.png\",\n            \"width\":null,\n            \"height\":21\n          },\n          \"small\":{\n            \"url\":\"http://localhost/media/thumbnails/small/cVPRnJU92oN82w9KxBTdfUwXtnrnmwps_24c65f362f804a7e6cbdc4a516fb1699a3b5ba31371eddd7ae367dd7b2a9862f.png\",\n            \"width\":48,\n            \"height\":48\n          },\n          \"card_cover\":{\n            \"url\":\"http://localhost/media/thumbnails/card_cover/cVPRnJU92oN82w9KxBTdfUwXtnrnmwps_24c65f362f804a7e6cbdc4a516fb1699a3b5ba31371eddd7ae367dd7b2a9862f.png\",\n            \"width\":300,\n            \"height\":160\n          }\n        },\n        \"visible_name\":\"Screenshot from 2025-04-20 16-00-28.png\",\n        \"name\":\"cVPRnJU92oN82w9KxBTdfUwXtnrnmwps_24c65f362f804a7e6cbdc4a516fb1699a3b5ba31371eddd7ae367dd7b2a9862f.png\",\n        \"size\":4027,\n        \"mime_type\":\"image/png\",\n        \"is_image\":true,\n        \"image_width\":119,\n        \"image_height\":83,\n        \"uploaded_at\":\"2025-04-20T13:01:01.307552+00:00\"\n      }\n    ],\n    \"Source\":\"http://www.onsemi.com/\",\n    \"Order Items\":[],\n    \"Datasheet\":[\n      {\n        \"url\":\"http://localhost/media/user_files/E3LGElXqSeBxejCnDa0wloo4TFLlbtJI_db8263db5968eb690e7d50a4b0e73ee7229157d2055ce384c7728b02cc1e1965.pdf\",\n        \"thumbnails\":null,\n        \"visible_name\":\"mmbf5486-d.pdf\",\n        \"name\":\"E3LGElXqSeBxejCnDa0wloo4TFLlbtJI_db8263db5968eb690e7d50a4b0e73ee7229157d2055ce384c7728b02cc1e1965.pdf\",\n        \"size\":266000,\n        \"mime_type\":\"application/pdf\",\n        \"is_image\":false,\n        \"image_width\":null,\n        \"image_height\":null,\n        \"uploaded_at\":\"2025-04-20T12:59:54.690046+00:00\"\n      }\n    ],\n    \"Part of a set\":[],\n    \"State\":{\n      \"id\":3001,\n      \"value\":\"Unknown\",\n      \"color\":\"dark-orange\"\n    },\n    \"Part Number\":\"40-00017\",\n    \"Revision\":\"A\",\n    \"Notes\":null,\n    \"Sourced By\":null,\n    \"Containing\":[],\n    \"Contained by\":[]\n  },\n  {\n    \"id\":86,\n    \"order\":\"31.00000000000000000000\",\n    \"Full PN\":\"40-00018 Rev.A\",\n    \"External Part Number\":\"MRF 134\",\n    \"Manufacturer\":[\n      {\n        \"id\":10,\n        \"value\":\"Macom\",\n        \"order\":\"10.00000000000000000000\"\n      }\n    ],\n    \"System\":{\n      \"id\":2967,\n      \"value\":\"Pre-amplifier\",\n      \"color\":\"dark-blue\"\n    },\n    \"Item description\":\"Q2 MOSFET\",\n    \"Price per unit\":null,\n    \"Image\":[],\n    \"Source\":\"\",\n    \"Order Items\":[],\n    \"Datasheet\":[],\n    \"Part of a set\":[],\n    \"State\":{\n      \"id\":3001,\n      \"value\":\"Unknown\",\n      \"color\":\"dark-orange\"\n    },\n    \"Part Number\":\"40-00018\",\n    \"Revision\":\"A\",\n    \"Notes\":null,\n    \"Sourced By\":null,\n    \"Containing\":[],\n    \"Contained by\":[]\n  },\n  {\n    \"id\":87,\n    \"order\":\"32.00000000000000000000\",\n    \"Full PN\":\"40-00019 Rev.A\",\n    \"External Part Number\":\"MRF 150\",\n    \"Manufacturer\":[\n      {\n        \"id\":10,\n        \"value\":\"Macom\",\n        \"order\":\"10.00000000000000000000\"\n      }\n    ],\n    \"System\":{\n      \"id\":2967,\n      \"value\":\"Pre-amplifier\",\n      \"color\":\"dark-blue\"\n    },\n    \"Item description\":\"Q3 MOSFET\",\n    \"Price per unit\":null,\n    \"Image\":[\n      {\n        \"url\":\"http://localhost/media/user_files/9TrjLzSark8ccBsZ8goKgU9SqfIM2w5Q_6625e1ad885d82b98a2285e3192ab2a1ee023686beffe81fd7072e2a7db8360f.png\",\n        \"thumbnails\":{\n          \"tiny\":{\n            \"url\":\"http://localhost/media/thumbnails/tiny/9TrjLzSark8ccBsZ8goKgU9SqfIM2w5Q_6625e1ad885d82b98a2285e3192ab2a1ee023686beffe81fd7072e2a7db8360f.png\",\n            \"width\":null,\n            \"height\":21\n          },\n          \"small\":{\n            \"url\":\"http://localhost/media/thumbnails/small/9TrjLzSark8ccBsZ8goKgU9SqfIM2w5Q_6625e1ad885d82b98a2285e3192ab2a1ee023686beffe81fd7072e2a7db8360f.png\",\n            \"width\":48,\n            \"height\":48\n          },\n          \"card_cover\":{\n            \"url\":\"http://localhost/media/thumbnails/card_cover/9TrjLzSark8ccBsZ8goKgU9SqfIM2w5Q_6625e1ad885d82b98a2285e3192ab2a1ee023686beffe81fd7072e2a7db8360f.png\",\n            \"width\":300,\n            \"height\":160\n          }\n        },\n        \"visible_name\":\"Screenshot from 2025-04-20 16-20-56.png\",\n        \"name\":\"9TrjLzSark8ccBsZ8goKgU9SqfIM2w5Q_6625e1ad885d82b98a2285e3192ab2a1ee023686beffe81fd7072e2a7db8360f.png\",\n        \"size\":9794,\n        \"mime_type\":\"image/png\",\n        \"is_image\":true,\n        \"image_width\":165,\n        \"image_height\":132,\n        \"uploaded_at\":\"2025-04-20T13:21:16.226326+00:00\"\n      }\n    ],\n    \"Source\":\"https://www.macom.com/products/product-detail/MRF150\",\n    \"Order Items\":[],\n    \"Datasheet\":[\n      {\n        \"url\":\"http://localhost/media/user_files/LMrK5NIqFdiuVDDtiNweVlZ8FOIr6bgV_1a34b5d222782b2efd20af6543442e306c497366c294672f9b4373bf8f1d5588.pdf\",\n        \"thumbnails\":null,\n        \"visible_name\":\"MRF150.pdf\",\n        \"name\":\"LMrK5NIqFdiuVDDtiNweVlZ8FOIr6bgV_1a34b5d222782b2efd20af6543442e306c497366c294672f9b4373bf8f1d5588.pdf\",\n        \"size\":742544,\n        \"mime_type\":\"application/pdf\",\n        \"is_image\":false,\n        \"image_width\":null,\n        \"image_height\":null,\n        \"uploaded_at\":\"2025-04-20T13:20:37.868448+00:00\"\n      }\n    ],\n    \"Part of a set\":[],\n    \"State\":{\n      \"id\":3001,\n      \"value\":\"Unknown\",\n      \"color\":\"dark-orange\"\n    },\n    \"Part Number\":\"40-00019\",\n    \"Revision\":\"A\",\n    \"Notes\":null,\n    \"Sourced By\":null,\n    \"Containing\":[],\n    \"Contained by\":[]\n  },\n  {\n    \"id\":90,\n    \"order\":\"33.00000000000000000000\",\n    \"Full PN\":\"40-00020 Rev.A\",\n    \"External Part Number\":\"Potentiometer 10kΩ\",\n    \"Manufacturer\":[],\n    \"System\":{\n      \"id\":2967,\n      \"value\":\"Pre-amplifier\",\n      \"color\":\"dark-blue\"\n    },\n    \"Item description\":\"PT1 SMT 0.5W\",\n    \"Price per unit\":null,\n    \"Image\":[],\n    \"Source\":\"\",\n    \"Order Items\":[],\n    \"Datasheet\":[],\n    \"Part of a set\":[],\n    \"State\":{\n      \"id\":3001,\n      \"value\":\"Unknown\",\n      \"color\":\"dark-orange\"\n    },\n    \"Part Number\":\"40-00020\",\n    \"Revision\":\"A\",\n    \"Notes\":null,\n    \"Sourced By\":null,\n    \"Containing\":[],\n    \"Contained by\":[]\n  },\n  {\n    \"id\":91,\n    \"order\":\"34.00000000000000000000\",\n    \"Full PN\":\"40-00021 Rev.A\",\n    \"External Part Number\":\"Potentiometer 11kΩ\",\n    \"Manufacturer\":[],\n    \"System\":{\n      \"id\":2967,\n      \"value\":\"Pre-amplifier\",\n      \"color\":\"dark-blue\"\n    },\n    \"Item description\":\"PT2 SMT 0.5W\",\n    \"Price per unit\":null,\n    \"Image\":[],\n    \"Source\":\"\",\n    \"Order Items\":[],\n    \"Datasheet\":[],\n    \"Part of a set\":[],\n    \"State\":{\n      \"id\":3001,\n      \"value\":\"Unknown\",\n      \"color\":\"dark-orange\"\n    },\n    \"Part Number\":\"40-00021\",\n    \"Revision\":\"A\",\n    \"Notes\":null,\n    \"Sourced By\":null,\n    \"Containing\":[],\n    \"Contained by\":[]\n  },\n  {\n    \"id\":92,\n    \"order\":\"35.00000000000000000000\",\n    \"Full PN\":\"40-00022 Rev.A\",\n    \"External Part Number\":\"Resistor 1MΩ\",\n    \"Manufacturer\":[],\n    \"System\":{\n      \"id\":2967,\n      \"value\":\"Pre-amplifier\",\n      \"color\":\"dark-blue\"\n    },\n    \"Item description\":\"R1 SMT 0.125W\",\n    \"Price per unit\":null,\n    \"Image\":[],\n    \"Source\":\"\",\n    \"Order Items\":[],\n    \"Datasheet\":[],\n    \"Part of a set\":[],\n    \"State\":{\n      \"id\":3001,\n      \"value\":\"Unknown\",\n      \"color\":\"dark-orange\"\n    },\n    \"Part Number\":\"40-00022\",\n    \"Revision\":\"A\",\n    \"Notes\":null,\n    \"Sourced By\":null,\n    \"Containing\":[],\n    \"Contained by\":[]\n  },\n  {\n    \"id\":93,\n    \"order\":\"36.00000000000000000000\",\n    \"Full PN\":\"40-00023 Rev.A\",\n    \"External Part Number\":\"Resistor 150Ω\",\n    \"Manufacturer\":[],\n    \"System\":{\n      \"id\":2967,\n      \"value\":\"Pre-amplifier\",\n      \"color\":\"dark-blue\"\n    },\n    \"Item description\":\"R2 SMT 0.125W\",\n    \"Price per unit\":null,\n    \"Image\":[],\n    \"Source\":\"\",\n    \"Order Items\":[],\n    \"Datasheet\":[],\n    \"Part of a set\":[],\n    \"State\":{\n      \"id\":3001,\n      \"value\":\"Unknown\",\n      \"color\":\"dark-orange\"\n    },\n    \"Part Number\":\"40-00023\",\n    \"Revision\":\"A\",\n    \"Notes\":null,\n    \"Sourced By\":null,\n    \"Containing\":[],\n    \"Contained by\":[]\n  },\n  {\n    \"id\":94,\n    \"order\":\"37.00000000000000000000\",\n    \"Full PN\":\"40-00024 Rev.A\",\n    \"External Part Number\":\"Resistor 22Ω\",\n    \"Manufacturer\":[],\n    \"System\":{\n      \"id\":2967,\n      \"value\":\"Pre-amplifier\",\n      \"color\":\"dark-blue\"\n    },\n    \"Item description\":\"R3 SMT 0.125W\",\n    \"Price per unit\":null,\n    \"Image\":[],\n    \"Source\":\"\",\n    \"Order Items\":[],\n    \"Datasheet\":[],\n    \"Part of a set\":[],\n    \"State\":{\n      \"id\":3001,\n      \"value\":\"Unknown\",\n      \"color\":\"dark-orange\"\n    },\n    \"Part Number\":\"40-00024\",\n    \"Revision\":\"A\",\n    \"Notes\":null,\n    \"Sourced By\":null,\n    \"Containing\":[],\n    \"Contained by\":[]\n  },\n  {\n    \"id\":95,\n    \"order\":\"38.00000000000000000000\",\n    \"Full PN\":\"40-00025 Rev.A\",\n    \"External Part Number\":\"Resistor 220Ω\",\n    \"Manufacturer\":[],\n    \"System\":{\n      \"id\":2967,\n      \"value\":\"Pre-amplifier\",\n      \"color\":\"dark-blue\"\n    },\n    \"Item description\":\"R4 SMT 0.25W\",\n    \"Price per unit\":null,\n    \"Image\":[],\n    \"Source\":\"\",\n    \"Order Items\":[],\n    \"Datasheet\":[],\n    \"Part of a set\":[],\n    \"State\":{\n      \"id\":3001,\n      \"value\":\"Unknown\",\n      \"color\":\"dark-orange\"\n    },\n    \"Part Number\":\"40-00025\",\n    \"Revision\":\"A\",\n    \"Notes\":null,\n    \"Sourced By\":null,\n    \"Containing\":[],\n    \"Contained by\":[]\n  },\n  {\n    \"id\":96,\n    \"order\":\"39.00000000000000000000\",\n    \"Full PN\":\"40-00026 Rev.A\",\n    \"External Part Number\":\"Resisitor 10kΩ\",\n    \"Manufacturer\":[],\n    \"System\":{\n      \"id\":2967,\n      \"value\":\"Pre-amplifier\",\n      \"color\":\"dark-blue\"\n    },\n    \"Item description\":\"R5 SMT 0.25W\",\n    \"Price per unit\":null,\n    \"Image\":[],\n    \"Source\":\"\",\n    \"Order Items\":[],\n    \"Datasheet\":[],\n    \"Part of a set\":[],\n    \"State\":{\n      \"id\":3001,\n      \"value\":\"Unknown\",\n      \"color\":\"dark-orange\"\n    },\n    \"Part Number\":\"40-00026\",\n    \"Revision\":\"A\",\n    \"Notes\":null,\n    \"Sourced By\":null,\n    \"Containing\":[],\n    \"Contained by\":[]\n  },\n  {\n    \"id\":97,\n    \"order\":\"40.00000000000000000000\",\n    \"Full PN\":\"40-00027 Rev.A\",\n    \"External Part Number\":\"Resistor 10Ω\",\n    \"Manufacturer\":[],\n    \"System\":{\n      \"id\":2967,\n      \"value\":\"Pre-amplifier\",\n      \"color\":\"dark-blue\"\n    },\n    \"Item description\":\"R6 SMT 0.5W\",\n    \"Price per unit\":null,\n    \"Image\":[],\n    \"Source\":\"\",\n    \"Order Items\":[],\n    \"Datasheet\":[],\n    \"Part of a set\":[],\n    \"State\":{\n      \"id\":3001,\n      \"value\":\"Unknown\",\n      \"color\":\"dark-orange\"\n    },\n    \"Part Number\":\"40-00027\",\n    \"Revision\":\"A\",\n    \"Notes\":null,\n    \"Sourced By\":null,\n    \"Containing\":[],\n    \"Contained by\":[]\n  },\n  {\n    \"id\":98,\n    \"order\":\"41.00000000000000000000\",\n    \"Full PN\":\"40-00028 Rev.A\",\n    \"External Part Number\":\"Resistor 220Ω\",\n    \"Manufacturer\":[],\n    \"System\":{\n      \"id\":2967,\n      \"value\":\"Pre-amplifier\",\n      \"color\":\"dark-blue\"\n    },\n    \"Item description\":\"R7 SMT 2W\",\n    \"Price per unit\":null,\n    \"Image\":[],\n    \"Source\":\"\",\n    \"Order Items\":[],\n    \"Datasheet\":[],\n    \"Part of a set\":[],\n    \"State\":{\n      \"id\":3001,\n      \"value\":\"Unknown\",\n      \"color\":\"dark-orange\"\n    },\n    \"Part Number\":\"40-00028\",\n    \"Revision\":\"A\",\n    \"Notes\":null,\n    \"Sourced By\":null,\n    \"Containing\":[],\n    \"Contained by\":[]\n  },\n  {\n    \"id\":99,\n    \"order\":\"42.00000000000000000000\",\n    \"Full PN\":\"40-00029 Rev.A\",\n    \"External Part Number\":\"Cap 1 nF\",\n    \"Manufacturer\":[],\n    \"System\":{\n      \"id\":2967,\n      \"value\":\"Pre-amplifier\",\n      \"color\":\"dark-blue\"\n    },\n    \"Item description\":\"C1 SMT\",\n    \"Price per unit\":null,\n    \"Image\":[],\n    \"Source\":\"\",\n    \"Order Items\":[],\n    \"Datasheet\":[],\n    \"Part of a set\":[],\n    \"State\":{\n      \"id\":3001,\n      \"value\":\"Unknown\",\n      \"color\":\"dark-orange\"\n    },\n    \"Part Number\":\"40-00029\",\n    \"Revision\":\"A\",\n    \"Notes\":null,\n    \"Sourced By\":null,\n    \"Containing\":[],\n    \"Contained by\":[]\n  },\n  {\n    \"id\":100,\n    \"order\":\"43.00000000000000000000\",\n    \"Full PN\":\"40-00030 Rev.A\",\n    \"External Part Number\":\"Variable Cap 4~25 nF\",\n    \"Manufacturer\":[],\n    \"System\":{\n      \"id\":2967,\n      \"value\":\"Pre-amplifier\",\n      \"color\":\"dark-blue\"\n    },\n    \"Item description\":\"C2 SMT\",\n    \"Price per unit\":null,\n    \"Image\":[],\n    \"Source\":\"\",\n    \"Order Items\":[],\n    \"Datasheet\":[],\n    \"Part of a set\":[],\n    \"State\":{\n      \"id\":3001,\n      \"value\":\"Unknown\",\n      \"color\":\"dark-orange\"\n    },\n    \"Part Number\":\"40-00030\",\n    \"Revision\":\"A\",\n    \"Notes\":null,\n    \"Sourced By\":null,\n    \"Containing\":[],\n    \"Contained by\":[]\n  },\n  {\n    \"id\":101,\n    \"order\":\"44.00000000000000000000\",\n    \"Full PN\":\"40-00031 Rev.A\",\n    \"External Part Number\":\"Cap 100 pF\",\n    \"Manufacturer\":[],\n    \"System\":{\n      \"id\":2967,\n      \"value\":\"Pre-amplifier\",\n      \"color\":\"dark-blue\"\n    },\n    \"Item description\":\"C3 SMT\",\n    \"Price per unit\":null,\n    \"Image\":[],\n    \"Source\":\"\",\n    \"Order Items\":[],\n    \"Datasheet\":[],\n    \"Part of a set\":[],\n    \"State\":{\n      \"id\":3001,\n      \"value\":\"Unknown\",\n      \"color\":\"dark-orange\"\n    },\n    \"Part Number\":\"40-00031\",\n    \"Revision\":\"A\",\n    \"Notes\":null,\n    \"Sourced By\":null,\n    \"Containing\":[],\n    \"Contained by\":[]\n  },\n  {\n    \"id\":102,\n    \"order\":\"45.00000000000000000000\",\n    \"Full PN\":\"40-00032 Rev.A\",\n    \"External Part Number\":\"Cap 10 nF\",\n    \"Manufacturer\":[],\n    \"System\":{\n      \"id\":2967,\n      \"value\":\"Pre-amplifier\",\n      \"color\":\"dark-blue\"\n    },\n    \"Item description\":\"C4 C5 C6 C8 C10 SMT\",\n    \"Price per unit\":null,\n    \"Image\":[],\n    \"Source\":\"\",\n    \"Order Items\":[],\n    \"Datasheet\":[],\n    \"Part of a set\":[],\n    \"State\":{\n      \"id\":3001,\n      \"value\":\"Unknown\",\n      \"color\":\"dark-orange\"\n    },\n    \"Part Number\":\"40-00032\",\n    \"Revision\":\"A\",\n    \"Notes\":null,\n    \"Sourced By\":null,\n    \"Containing\":[],\n    \"Contained by\":[]\n  },\n  {\n    \"id\":103,\n    \"order\":\"46.00000000000000000000\",\n    \"Full PN\":\"40-00033 Rev.A\",\n    \"External Part Number\":\"Cap 100 nF\",\n    \"Manufacturer\":[],\n    \"System\":{\n      \"id\":2967,\n      \"value\":\"Pre-amplifier\",\n      \"color\":\"dark-blue\"\n    },\n    \"Item description\":\"C7 SMT\",\n    \"Price per unit\":null,\n    \"Image\":[],\n    \"Source\":\"\",\n    \"Order Items\":[],\n    \"Datasheet\":[],\n    \"Part of a set\":[],\n    \"State\":{\n      \"id\":3001,\n      \"value\":\"Unknown\",\n      \"color\":\"dark-orange\"\n    },\n    \"Part Number\":\"40-00033\",\n    \"Revision\":\"A\",\n    \"Notes\":null,\n    \"Sourced By\":null,\n    \"Containing\":[],\n    \"Contained by\":[]\n  },\n  {\n    \"id\":104,\n    \"order\":\"47.00000000000000000000\",\n    \"Full PN\":\"40-00034 Rev.A\",\n    \"External Part Number\":\"Cap 10 nF ATC\",\n    \"Manufacturer\":[\n      {\n        \"id\":13,\n        \"value\":\"ATC (AVX (Kyocera))\",\n        \"order\":\"13.00000000000000000000\"\n      }\n    ],\n    \"System\":{\n      \"id\":2967,\n      \"value\":\"Pre-amplifier\",\n      \"color\":\"dark-blue\"\n    },\n    \"Item description\":\"C9 C15 SMT\",\n    \"Price per unit\":null,\n    \"Image\":[],\n    \"Source\":\"\",\n    \"Order Items\":[],\n    \"Datasheet\":[],\n    \"Part of a set\":[],\n    \"State\":{\n      \"id\":3001,\n      \"value\":\"Unknown\",\n      \"color\":\"dark-orange\"\n    },\n    \"Part Number\":\"40-00034\",\n    \"Revision\":\"A\",\n    \"Notes\":null,\n    \"Sourced By\":null,\n    \"Containing\":[],\n    \"Contained by\":[]\n  },\n  {\n    \"id\":105,\n    \"order\":\"48.00000000000000000000\",\n    \"Full PN\":\"40-00035 Rev.A\",\n    \"External Part Number\":\"Cap 100 µF\",\n    \"Manufacturer\":[],\n    \"System\":{\n      \"id\":2967,\n      \"value\":\"Pre-amplifier\",\n      \"color\":\"dark-blue\"\n    },\n    \"Item description\":\"C10 C21 C23 SMT Electrolyte\",\n    \"Price per unit\":null,\n    \"Image\":[],\n    \"Source\":\"\",\n    \"Order Items\":[],\n    \"Datasheet\":[],\n    \"Part of a set\":[],\n    \"State\":{\n      \"id\":3001,\n      \"value\":\"Unknown\",\n      \"color\":\"dark-orange\"\n    },\n    \"Part Number\":\"40-00035\",\n    \"Revision\":\"A\",\n    \"Notes\":null,\n    \"Sourced By\":null,\n    \"Containing\":[],\n    \"Contained by\":[]\n  },\n  {\n    \"id\":106,\n    \"order\":\"49.00000000000000000000\",\n    \"Full PN\":\"40-00036 Rev.A\",\n    \"External Part Number\":\"486-1226-ND\",\n    \"Manufacturer\":[\n      {\n        \"id\":12,\n        \"value\":\"SCHURTER Inc.\",\n        \"order\":\"12.00000000000000000000\"\n      }\n    ],\n    \"System\":{\n      \"id\":2964,\n      \"value\":\"AC-Mains Compartment\",\n      \"color\":\"dark-gray\"\n    },\n    \"Item description\":\"250V 10A Fuse\",\n    \"Price per unit\":\"0.76\",\n    \"Image\":[\n      {\n        \"url\":\"http://localhost/media/user_files/8RIBbdPBuMIlD7PsZrCLfYGR6ASk0Clb_12f6e287509ad64284981bedf005d74c0c1bb5beaf223dcda5b5384b222eb06e.jpg\",\n        \"thumbnails\":{\n          \"tiny\":{\n            \"url\":\"http://localhost/media/thumbnails/tiny/8RIBbdPBuMIlD7PsZrCLfYGR6ASk0Clb_12f6e287509ad64284981bedf005d74c0c1bb5beaf223dcda5b5384b222eb06e.jpg\",\n            \"width\":null,\n            \"height\":21\n          },\n          \"small\":{\n            \"url\":\"http://localhost/media/thumbnails/small/8RIBbdPBuMIlD7PsZrCLfYGR6ASk0Clb_12f6e287509ad64284981bedf005d74c0c1bb5beaf223dcda5b5384b222eb06e.jpg\",\n            \"width\":48,\n            \"height\":48\n          },\n          \"card_cover\":{\n            \"url\":\"http://localhost/media/thumbnails/card_cover/8RIBbdPBuMIlD7PsZrCLfYGR6ASk0Clb_12f6e287509ad64284981bedf005d74c0c1bb5beaf223dcda5b5384b222eb06e.jpg\",\n            \"width\":300,\n            \"height\":160\n          }\n        },\n        \"visible_name\":\"DIi10BC9EB3kdFeBv9ANtCG0l9Y61hW...beaf223dcda5b5384b222eb06e.jpg\",\n        \"name\":\"8RIBbdPBuMIlD7PsZrCLfYGR6ASk0Clb_12f6e287509ad64284981bedf005d74c0c1bb5beaf223dcda5b5384b222eb06e.jpg\",\n        \"size\":93598,\n        \"mime_type\":\"image/jpeg\",\n        \"is_image\":true,\n        \"image_width\":640,\n        \"image_height\":640,\n        \"uploaded_at\":\"2025-05-04T13:45:11.889081+00:00\"\n      }\n    ],\n    \"Source\":\"https://www.digikey.co.il/he/products/detail/schurter-inc/0034-3127/640142\",\n    \"Order Items\":[\n      {\n        \"id\":27,\n        \"value\":\"5e7ffbeb-6c94-43f0-8047-aa3610987c6e\",\n        \"order\":\"25.00000000000000000000\"\n      }\n    ],\n    \"Datasheet\":[\n      {\n        \"url\":\"http://localhost/media/user_files/R41kJUQPfN7DAuAytGjrQX3P29dCBYAg_5169f408200b5edf4e5c6703f18cef53850f83d151e78161311ce463a77a3eb2.pdf\",\n        \"thumbnails\":null,\n        \"visible_name\":\"typ_FST_5x20.pdf\",\n        \"name\":\"R41kJUQPfN7DAuAytGjrQX3P29dCBYAg_5169f408200b5edf4e5c6703f18cef53850f83d151e78161311ce463a77a3eb2.pdf\",\n        \"size\":309755,\n        \"mime_type\":\"application/pdf\",\n        \"is_image\":false,\n        \"image_width\":null,\n        \"image_height\":null,\n        \"uploaded_at\":\"2025-04-22T06:42:01.068758+00:00\"\n      }\n    ],\n    \"Part of a set\":[],\n    \"State\":{\n      \"id\":3001,\n      \"value\":\"Unknown\",\n      \"color\":\"dark-orange\"\n    },\n    \"Part Number\":\"40-00036\",\n    \"Revision\":\"A\",\n    \"Notes\":null,\n    \"Sourced By\":null,\n    \"Containing\":[],\n    \"Contained by\":[]\n  },\n  {\n    \"id\":107,\n    \"order\":\"50.00000000000000000000\",\n    \"Full PN\":\"40-00037 Rev.A\",\n    \"External Part Number\":\"Cap 1 nF ATC\",\n    \"Manufacturer\":[\n      {\n        \"id\":13,\n        \"value\":\"ATC (AVX (Kyocera))\",\n        \"order\":\"13.00000000000000000000\"\n      }\n    ],\n    \"System\":{\n      \"id\":2967,\n      \"value\":\"Pre-amplifier\",\n      \"color\":\"dark-blue\"\n    },\n    \"Item description\":\"C12 C14 C19 SMT\",\n    \"Price per unit\":null,\n    \"Image\":[],\n    \"Source\":\"\",\n    \"Order Items\":[],\n    \"Datasheet\":[],\n    \"Part of a set\":[],\n    \"State\":{\n      \"id\":3001,\n      \"value\":\"Unknown\",\n      \"color\":\"dark-orange\"\n    },\n    \"Part Number\":\"40-00037\",\n    \"Revision\":\"A\",\n    \"Notes\":null,\n    \"Sourced By\":null,\n    \"Containing\":[],\n    \"Contained by\":[]\n  },\n  {\n    \"id\":108,\n    \"order\":\"51.00000000000000000000\",\n    \"Full PN\":\"40-00038 Rev.A\",\n    \"External Part Number\":\"Cap 140 pF ATC\",\n    \"Manufacturer\":[\n      {\n        \"id\":13,\n        \"value\":\"ATC (AVX (Kyocera))\",\n        \"order\":\"13.00000000000000000000\"\n      }\n    ],\n    \"System\":{\n      \"id\":2967,\n      \"value\":\"Pre-amplifier\",\n      \"color\":\"dark-blue\"\n    },\n    \"Item description\":\"C13 SMT\",\n    \"Price per unit\":null,\n    \"Image\":[],\n    \"Source\":\"\",\n    \"Order Items\":[],\n    \"Datasheet\":[],\n    \"Part of a set\":[],\n    \"State\":{\n      \"id\":3001,\n      \"value\":\"Unknown\",\n      \"color\":\"dark-orange\"\n    },\n    \"Part Number\":\"40-00038\",\n    \"Revision\":\"A\",\n    \"Notes\":null,\n    \"Sourced By\":null,\n    \"Containing\":[],\n    \"Contained by\":[]\n  },\n  {\n    \"id\":109,\n    \"order\":\"52.00000000000000000000\",\n    \"Full PN\":\"40-00039 Rev.A\",\n    \"External Part Number\":\"Cap 220 µF\",\n    \"Manufacturer\":[],\n    \"System\":{\n      \"id\":2967,\n      \"value\":\"Pre-amplifier\",\n      \"color\":\"dark-blue\"\n    },\n    \"Item description\":\"C16 SMT Electrolyte\",\n    \"Price per unit\":null,\n    \"Image\":[],\n    \"Source\":\"\",\n    \"Order Items\":[],\n    \"Datasheet\":[],\n    \"Part of a set\":[],\n    \"State\":{\n      \"id\":3001,\n      \"value\":\"Unknown\",\n      \"color\":\"dark-orange\"\n    },\n    \"Part Number\":\"40-00039\",\n    \"Revision\":\"A\",\n    \"Notes\":null,\n    \"Sourced By\":null,\n    \"Containing\":[],\n    \"Contained by\":[]\n  },\n  {\n    \"id\":110,\n    \"order\":\"53.00000000000000000000\",\n    \"Full PN\":\"40-00040 Rev.A\",\n    \"External Part Number\":\"Cap 100 nF ATC\",\n    \"Manufacturer\":[\n      {\n        \"id\":13,\n        \"value\":\"ATC (AVX (Kyocera))\",\n        \"order\":\"13.00000000000000000000\"\n      }\n    ],\n    \"System\":{\n      \"id\":2967,\n      \"value\":\"Pre-amplifier\",\n      \"color\":\"dark-blue\"\n    },\n    \"Item description\":\"C17 C20 C22 SMT\",\n    \"Price per unit\":null,\n    \"Image\":[],\n    \"Source\":\"\",\n    \"Order Items\":[],\n    \"Datasheet\":[],\n    \"Part of a set\":[],\n    \"State\":{\n      \"id\":3001,\n      \"value\":\"Unknown\",\n      \"color\":\"dark-orange\"\n    },\n    \"Part Number\":\"40-00040\",\n    \"Revision\":\"A\",\n    \"Notes\":null,\n    \"Sourced By\":null,\n    \"Containing\":[],\n    \"Contained by\":[]\n  },\n  {\n    \"id\":111,\n    \"order\":\"54.00000000000000000000\",\n    \"Full PN\":\"40-00041 Rev.A\",\n    \"External Part Number\":\"Cap 200 pF ATC\",\n    \"Manufacturer\":[\n      {\n        \"id\":13,\n        \"value\":\"ATC (AVX (Kyocera))\",\n        \"order\":\"13.00000000000000000000\"\n      }\n    ],\n    \"System\":{\n      \"id\":2967,\n      \"value\":\"Pre-amplifier\",\n      \"color\":\"dark-blue\"\n    },\n    \"Item description\":\"C18\",\n    \"Price per unit\":null,\n    \"Image\":[],\n    \"Source\":\"\",\n    \"Order Items\":[],\n    \"Datasheet\":[],\n    \"Part of a set\":[],\n    \"State\":{\n      \"id\":3001,\n      \"value\":\"Unknown\",\n      \"color\":\"dark-orange\"\n    },\n    \"Part Number\":\"40-00041\",\n    \"Revision\":\"A\",\n    \"Notes\":null,\n    \"Sourced By\":null,\n    \"Containing\":[],\n    \"Contained by\":[]\n  },\n  {\n    \"id\":113,\n    \"order\":\"55.00000000000000000000\",\n    \"Full PN\":\"40-00042 Rev.A\",\n    \"External Part Number\":\"Coil 5 µH 0805 2mm\",\n    \"Manufacturer\":[\n      {\n        \"id\":14,\n        \"value\":\"Fastron Group\",\n        \"order\":\"14.00000000000000000000\"\n      }\n    ],\n    \"System\":{\n      \"id\":2967,\n      \"value\":\"Pre-amplifier\",\n      \"color\":\"dark-blue\"\n    },\n    \"Item description\":\"L1 L2 L8 SMT\",\n    \"Price per unit\":\"0.23\",\n    \"Image\":[\n      {\n        \"url\":\"http://localhost/media/user_files/iX1PPC27cYZMOgxhd0QlL3MrfGK93nbu_9d5c299cf85f1c81e1958820ff3cfd37221b56cb72b1cd3e8abdff0c0b302d1f.png\",\n        \"thumbnails\":{\n          \"tiny\":{\n            \"url\":\"http://localhost/media/thumbnails/tiny/iX1PPC27cYZMOgxhd0QlL3MrfGK93nbu_9d5c299cf85f1c81e1958820ff3cfd37221b56cb72b1cd3e8abdff0c0b302d1f.png\",\n            \"width\":null,\n            \"height\":21\n          },\n          \"small\":{\n            \"url\":\"http://localhost/media/thumbnails/small/iX1PPC27cYZMOgxhd0QlL3MrfGK93nbu_9d5c299cf85f1c81e1958820ff3cfd37221b56cb72b1cd3e8abdff0c0b302d1f.png\",\n            \"width\":48,\n            \"height\":48\n          },\n          \"card_cover\":{\n            \"url\":\"http://localhost/media/thumbnails/card_cover/iX1PPC27cYZMOgxhd0QlL3MrfGK93nbu_9d5c299cf85f1c81e1958820ff3cfd37221b56cb72b1cd3e8abdff0c0b302d1f.png\",\n            \"width\":300,\n            \"height\":160\n          }\n        },\n        \"visible_name\":\"image.png\",\n        \"name\":\"iX1PPC27cYZMOgxhd0QlL3MrfGK93nbu_9d5c299cf85f1c81e1958820ff3cfd37221b56cb72b1cd3e8abdff0c0b302d1f.png\",\n        \"size\":97380,\n        \"mime_type\":\"image/png\",\n        \"is_image\":true,\n        \"image_width\":407,\n        \"image_height\":369,\n        \"uploaded_at\":\"2025-05-04T14:36:51.005974+00:00\"\n      }\n    ],\n    \"Source\":\"https://www.reichelt.com/de/en/shop/product/smd_inductor_0805_ceramic_5_6_h-255502?CCTYPE=business\",\n    \"Order Items\":[],\n    \"Datasheet\":[\n      {\n        \"url\":\"http://localhost/media/user_files/a8ru8FUUbe7yA1oxBygoW8RdggymmHkj_67e0ab4d1a55cd6f145a1ee97d10983fd5fe13f9a1eda33ad13099d78218340e.pdf\",\n        \"thumbnails\":null,\n        \"visible_name\":\"0805AS.pdf\",\n        \"name\":\"a8ru8FUUbe7yA1oxBygoW8RdggymmHkj_67e0ab4d1a55cd6f145a1ee97d10983fd5fe13f9a1eda33ad13099d78218340e.pdf\",\n        \"size\":231437,\n        \"mime_type\":\"application/pdf\",\n        \"is_image\":false,\n        \"image_width\":null,\n        \"image_height\":null,\n        \"uploaded_at\":\"2025-05-04T14:35:47.949632+00:00\"\n      }\n    ],\n    \"Part of a set\":[],\n    \"State\":{\n      \"id\":3001,\n      \"value\":\"Unknown\",\n      \"color\":\"dark-orange\"\n    },\n    \"Part Number\":\"40-00042\",\n    \"Revision\":\"A\",\n    \"Notes\":null,\n    \"Sourced By\":null,\n    \"Containing\":[],\n    \"Contained by\":[]\n  },\n  {\n    \"id\":114,\n    \"order\":\"56.00000000000000000000\",\n    \"Full PN\":\"40-00043 Rev.A\",\n    \"External Part Number\":\"Coil 45 µH\",\n    \"Manufacturer\":[],\n    \"System\":{\n      \"id\":2967,\n      \"value\":\"Pre-amplifier\",\n      \"color\":\"dark-blue\"\n    },\n    \"Item description\":\"L3, SMT\",\n    \"Price per unit\":null,\n    \"Image\":[],\n    \"Source\":\"\",\n    \"Order Items\":[],\n    \"Datasheet\":[],\n    \"Part of a set\":[],\n    \"State\":{\n      \"id\":3001,\n      \"value\":\"Unknown\",\n      \"color\":\"dark-orange\"\n    },\n    \"Part Number\":\"40-00043\",\n    \"Revision\":\"A\",\n    \"Notes\":null,\n    \"Sourced By\":null,\n    \"Containing\":[],\n    \"Contained by\":[]\n  },\n  {\n    \"id\":115,\n    \"order\":\"57.00000000000000000000\",\n    \"Full PN\":\"40-00044 Rev.A\",\n    \"External Part Number\":\"Coil 0.1 µH 20 mm\",\n    \"Manufacturer\":[],\n    \"System\":{\n      \"id\":2967,\n      \"value\":\"Pre-amplifier\",\n      \"color\":\"dark-blue\"\n    },\n    \"Item description\":\"L4 L7, Solid conductor, Cu 1.2mm, \\nǾ 9mm, 5 turns\",\n    \"Price per unit\":null,\n    \"Image\":[],\n    \"Source\":\"\",\n    \"Order Items\":[],\n    \"Datasheet\":[],\n    \"Part of a set\":[],\n    \"State\":{\n      \"id\":3001,\n      \"value\":\"Unknown\",\n      \"color\":\"dark-orange\"\n    },\n    \"Part Number\":\"40-00044\",\n    \"Revision\":\"A\",\n    \"Notes\":null,\n    \"Sourced By\":null,\n    \"Containing\":[],\n    \"Contained by\":[]\n  },\n  {\n    \"id\":116,\n    \"order\":\"58.00000000000000000000\",\n    \"Full PN\":\"40-00045 Rev.A\",\n    \"External Part Number\":\"Coil 1.2 µH 25 mm\",\n    \"Manufacturer\":[],\n    \"System\":{\n      \"id\":2967,\n      \"value\":\"Pre-amplifier\",\n      \"color\":\"dark-blue\"\n    },\n    \"Item description\":\"L5, Solid conductor, Cu 1.2 mm\\nǾ 15 mm, 13 turns\",\n    \"Price per unit\":null,\n    \"Image\":[],\n    \"Source\":\"\",\n    \"Order Items\":[],\n    \"Datasheet\":[],\n    \"Part of a set\":[],\n    \"State\":{\n      \"id\":3001,\n      \"value\":\"Unknown\",\n      \"color\":\"dark-orange\"\n    },\n    \"Part Number\":\"40-00045\",\n    \"Revision\":\"A\",\n    \"Notes\":null,\n    \"Sourced By\":null,\n    \"Containing\":[],\n    \"Contained by\":[]\n  },\n  {\n    \"id\":117,\n    \"order\":\"59.00000000000000000000\",\n    \"Full PN\":\"40-00046 Rev.A\",\n    \"External Part Number\":\"Coil 45 µH 18 mm\",\n    \"Manufacturer\":[],\n    \"System\":{\n      \"id\":2967,\n      \"value\":\"Pre-amplifier\",\n      \"color\":\"dark-blue\"\n    },\n    \"Item description\":\"L6, Balun\",\n    \"Price per unit\":null,\n    \"Image\":[],\n    \"Source\":\"\",\n    \"Order Items\":[],\n    \"Datasheet\":[],\n    \"Part of a set\":[],\n    \"State\":{\n      \"id\":3001,\n      \"value\":\"Unknown\",\n      \"color\":\"dark-orange\"\n    },\n    \"Part Number\":\"40-00046\",\n    \"Revision\":\"A\",\n    \"Notes\":null,\n    \"Sourced By\":null,\n    \"Containing\":[],\n    \"Contained by\":[]\n  },\n  {\n    \"id\":118,\n    \"order\":\"60.00000000000000000000\",\n    \"Full PN\":\"40-00047 Rev.A\",\n    \"External Part Number\":\"40.68 MHz Quatz Crystal\",\n    \"Manufacturer\":[],\n    \"System\":{\n      \"id\":2967,\n      \"value\":\"Pre-amplifier\",\n      \"color\":\"dark-blue\"\n    },\n    \"Item description\":\"Y1, CB619 or equivalent\",\n    \"Price per unit\":null,\n    \"Image\":[],\n    \"Source\":\"\",\n    \"Order Items\":[],\n    \"Datasheet\":[],\n    \"Part of a set\":[],\n    \"State\":{\n      \"id\":3001,\n      \"value\":\"Unknown\",\n      \"color\":\"dark-orange\"\n    },\n    \"Part Number\":\"40-00047\",\n    \"Revision\":\"A\",\n    \"Notes\":null,\n    \"Sourced By\":null,\n    \"Containing\":[],\n    \"Contained by\":[]\n  },\n  {\n    \"id\":119,\n    \"order\":\"61.00000000000000000000\",\n    \"Full PN\":\"40-00048 Rev.A\",\n    \"External Part Number\":\"LM2940S\",\n    \"Manufacturer\":[],\n    \"System\":{\n      \"id\":2967,\n      \"value\":\"Pre-amplifier\",\n      \"color\":\"dark-blue\"\n    },\n    \"Item description\":\"Voltage Regulator, 24V in, 10V out.\",\n    \"Price per unit\":\"2.46\",\n    \"Image\":[\n      {\n        \"url\":\"http://localhost/media/user_files/6Iutt4iYU2VHMnPbfYPsIVqJPWo0iDHw_ca640dccf594369b70295a22f4fca745a0b59680963fdc3394c29529b24f9ac8.png\",\n        \"thumbnails\":{\n          \"tiny\":{\n            \"url\":\"http://localhost/media/thumbnails/tiny/6Iutt4iYU2VHMnPbfYPsIVqJPWo0iDHw_ca640dccf594369b70295a22f4fca745a0b59680963fdc3394c29529b24f9ac8.png\",\n            \"width\":null,\n            \"height\":21\n          },\n          \"small\":{\n            \"url\":\"http://localhost/media/thumbnails/small/6Iutt4iYU2VHMnPbfYPsIVqJPWo0iDHw_ca640dccf594369b70295a22f4fca745a0b59680963fdc3394c29529b24f9ac8.png\",\n            \"width\":48,\n            \"height\":48\n          },\n          \"card_cover\":{\n            \"url\":\"http://localhost/media/thumbnails/card_cover/6Iutt4iYU2VHMnPbfYPsIVqJPWo0iDHw_ca640dccf594369b70295a22f4fca745a0b59680963fdc3394c29529b24f9ac8.png\",\n            \"width\":300,\n            \"height\":160\n          }\n        },\n        \"visible_name\":\"image.png\",\n        \"name\":\"6Iutt4iYU2VHMnPbfYPsIVqJPWo0iDHw_ca640dccf594369b70295a22f4fca745a0b59680963fdc3394c29529b24f9ac8.png\",\n        \"size\":16697,\n        \"mime_type\":\"image/png\",\n        \"is_image\":true,\n        \"image_width\":150,\n        \"image_height\":150,\n        \"uploaded_at\":\"2025-05-12T06:56:18.053364+00:00\"\n      }\n    ],\n    \"Source\":\"https://www.mouser.co.il/ProductDetail/Texas-Instruments/LM2940S-10-NOPB?qs=X1J7HmVL2ZEk%252BMh0AmJl0Q%3D%3D\",\n    \"Order Items\":[],\n    \"Datasheet\":[\n      {\n        \"url\":\"http://localhost/media/user_files/rfffAAwdH5BCOF9sX4xXRA0xLR0P8gW4_18cf431eca45d321eecd2290bf1e01d8e2fb8789b6a5f1a25da1559ffc1eb1dc.\",\n        \"thumbnails\":null,\n        \"visible_name\":\"lm2940c\",\n        \"name\":\"rfffAAwdH5BCOF9sX4xXRA0xLR0P8gW4_18cf431eca45d321eecd2290bf1e01d8e2fb8789b6a5f1a25da1559ffc1eb1dc.\",\n        \"size\":2144138,\n        \"mime_type\":\"application/pdf\",\n        \"is_image\":false,\n        \"image_width\":null,\n        \"image_height\":null,\n        \"uploaded_at\":\"2025-05-12T06:56:56.818253+00:00\"\n      }\n    ],\n    \"Part of a set\":[],\n    \"State\":{\n      \"id\":3001,\n      \"value\":\"Unknown\",\n      \"color\":\"dark-orange\"\n    },\n    \"Part Number\":\"40-00048\",\n    \"Revision\":\"A\",\n    \"Notes\":null,\n    \"Sourced By\":null,\n    \"Containing\":[],\n    \"Contained by\":[]\n  },\n  {\n    \"id\":120,\n    \"order\":\"62.00000000000000000000\",\n    \"Full PN\":\"40-00049 Rev.A\",\n    \"External Part Number\":\"Cap 100pF ±5%\",\n    \"Manufacturer\":[\n      {\n        \"id\":15,\n        \"value\":\"AVX (Kyocera)\",\n        \"order\":\"15.00000000000000000000\"\n      }\n    ],\n    \"System\":{\n      \"id\":2990,\n      \"value\":\"Amplifier\",\n      \"color\":\"darker-cyan\"\n    },\n    \"Item description\":\"C1, C2, C21, C22 800B101JW500X\",\n    \"Price per unit\":null,\n    \"Image\":[],\n    \"Source\":\"\",\n    \"Order Items\":[],\n    \"Datasheet\":[\n      {\n        \"url\":\"http://localhost/media/user_files/KlloGZLbiZiUnONMj4tTiRjMZVs6XXSO_b0193ac0a3fea42aada5039f50ddbf65d726ad7d9439cbb07e8a0213a1ce5c54.pdf\",\n        \"thumbnails\":null,\n        \"visible_name\":\"800B.pdf\",\n        \"name\":\"KlloGZLbiZiUnONMj4tTiRjMZVs6XXSO_b0193ac0a3fea42aada5039f50ddbf65d726ad7d9439cbb07e8a0213a1ce5c54.pdf\",\n        \"size\":1087810,\n        \"mime_type\":\"application/pdf\",\n        \"is_image\":false,\n        \"image_width\":null,\n        \"image_height\":null,\n        \"uploaded_at\":\"2025-05-06T09:21:53.253018+00:00\"\n      }\n    ],\n    \"Part of a set\":[],\n    \"State\":{\n      \"id\":3001,\n      \"value\":\"Unknown\",\n      \"color\":\"dark-orange\"\n    },\n    \"Part Number\":\"40-00049\",\n    \"Revision\":\"A\",\n    \"Notes\":null,\n    \"Sourced By\":null,\n    \"Containing\":[],\n    \"Contained by\":[]\n  },\n  {\n    \"id\":121,\n    \"order\":\"63.00000000000000000000\",\n    \"Full PN\":\"40-00050 Rev.A\",\n    \"External Part Number\":\"Cap 1nF ±5%\",\n    \"Manufacturer\":[\n      {\n        \"id\":15,\n        \"value\":\"AVX (Kyocera)\",\n        \"order\":\"15.00000000000000000000\"\n      }\n    ],\n    \"System\":{\n      \"id\":2990,\n      \"value\":\"Amplifier\",\n      \"color\":\"darker-cyan\"\n    },\n    \"Item description\":\"C3, C4, C23, C24 800B101JW500X\",\n    \"Price per unit\":null,\n    \"Image\":[],\n    \"Source\":\"\",\n    \"Order Items\":[],\n    \"Datasheet\":[\n      {\n        \"url\":\"http://localhost/media/user_files/KlloGZLbiZiUnONMj4tTiRjMZVs6XXSO_b0193ac0a3fea42aada5039f50ddbf65d726ad7d9439cbb07e8a0213a1ce5c54.pdf\",\n        \"thumbnails\":null,\n        \"visible_name\":\"800B.pdf\",\n        \"name\":\"KlloGZLbiZiUnONMj4tTiRjMZVs6XXSO_b0193ac0a3fea42aada5039f50ddbf65d726ad7d9439cbb07e8a0213a1ce5c54.pdf\",\n        \"size\":1087810,\n        \"mime_type\":\"application/pdf\",\n        \"is_image\":false,\n        \"image_width\":null,\n        \"image_height\":null,\n        \"uploaded_at\":\"2025-05-06T09:21:53.253018+00:00\"\n      }\n    ],\n    \"Part of a set\":[],\n    \"State\":{\n      \"id\":3001,\n      \"value\":\"Unknown\",\n      \"color\":\"dark-orange\"\n    },\n    \"Part Number\":\"40-00050\",\n    \"Revision\":\"A\",\n    \"Notes\":null,\n    \"Sourced By\":null,\n    \"Containing\":[],\n    \"Contained by\":[]\n  },\n  {\n    \"id\":122,\n    \"order\":\"64.00000000000000000000\",\n    \"Full PN\":\"40-00051 Rev.A\",\n    \"External Part Number\":\"Cap 1µF ±10%\",\n    \"Manufacturer\":[\n      {\n        \"id\":16,\n        \"value\":\"TDK (Capacitors division)\",\n        \"order\":\"16.00000000000000000000\"\n      }\n    ],\n    \"System\":{\n      \"id\":2990,\n      \"value\":\"Amplifier\",\n      \"color\":\"darker-cyan\"\n    },\n    \"Item description\":\"C5, C6 C2012X7S2A105K\",\n    \"Price per unit\":\"0.37\",\n    \"Image\":[\n      {\n        \"url\":\"http://localhost/media/user_files/wrTejNjwuHylwfkEtmbapGF5vkwdBzop_af64773f39a6742e2e5840a411e85bb4d261c24f86bdb7022240df483b1748c1.webp\",\n        \"thumbnails\":{\n          \"tiny\":{\n            \"url\":\"http://localhost/media/thumbnails/tiny/wrTejNjwuHylwfkEtmbapGF5vkwdBzop_af64773f39a6742e2e5840a411e85bb4d261c24f86bdb7022240df483b1748c1.webp\",\n            \"width\":null,\n            \"height\":21\n          },\n          \"small\":{\n            \"url\":\"http://localhost/media/thumbnails/small/wrTejNjwuHylwfkEtmbapGF5vkwdBzop_af64773f39a6742e2e5840a411e85bb4d261c24f86bdb7022240df483b1748c1.webp\",\n            \"width\":48,\n            \"height\":48\n          },\n          \"card_cover\":{\n            \"url\":\"http://localhost/media/thumbnails/card_cover/wrTejNjwuHylwfkEtmbapGF5vkwdBzop_af64773f39a6742e2e5840a411e85bb4d261c24f86bdb7022240df483b1748c1.webp\",\n            \"width\":300,\n            \"height\":160\n          }\n        },\n        \"visible_name\":\"c2012jb0j156m085ab_DFI_SPL.webp\",\n        \"name\":\"wrTejNjwuHylwfkEtmbapGF5vkwdBzop_af64773f39a6742e2e5840a411e85bb4d261c24f86bdb7022240df483b1748c1.webp\",\n        \"size\":1502,\n        \"mime_type\":\"image/webp\",\n        \"is_image\":true,\n        \"image_width\":150,\n        \"image_height\":150,\n        \"uploaded_at\":\"2025-05-06T09:33:33.538875+00:00\"\n      }\n    ],\n    \"Source\":\"\",\n    \"Order Items\":[],\n    \"Datasheet\":[\n      {\n        \"url\":\"http://localhost/media/user_files/CYnH5GuGDBRrshrOPJldVSGNqNOJOLrg_34a049855aae7c35613b6056c0252b57ca69ed281abe8984535a99ddd5aa26e7.pdf\",\n        \"thumbnails\":null,\n        \"visible_name\":\"mlcc_commercial_midvoltage_en.pdf\",\n        \"name\":\"CYnH5GuGDBRrshrOPJldVSGNqNOJOLrg_34a049855aae7c35613b6056c0252b57ca69ed281abe8984535a99ddd5aa26e7.pdf\",\n        \"size\":1042083,\n        \"mime_type\":\"application/pdf\",\n        \"is_image\":false,\n        \"image_width\":null,\n        \"image_height\":null,\n        \"uploaded_at\":\"2025-05-06T09:34:48.798973+00:00\"\n      }\n    ],\n    \"Part of a set\":[],\n    \"State\":{\n      \"id\":3001,\n      \"value\":\"Unknown\",\n      \"color\":\"dark-orange\"\n    },\n    \"Part Number\":\"40-00051\",\n    \"Revision\":\"A\",\n    \"Notes\":null,\n    \"Sourced By\":null,\n    \"Containing\":[],\n    \"Contained by\":[]\n  },\n  {\n    \"id\":123,\n    \"order\":\"65.00000000000000000000\",\n    \"Full PN\":\"40-00052 Rev.A\",\n    \"External Part Number\":\"Cap 10µF ±10%\",\n    \"Manufacturer\":[\n      {\n        \"id\":17,\n        \"value\":\"Murata\",\n        \"order\":\"17.00000000000000000000\"\n      }\n    ],\n    \"System\":{\n      \"id\":2990,\n      \"value\":\"Amplifier\",\n      \"color\":\"darker-cyan\"\n    },\n    \"Item description\":\"C7, C8 GRM32EC72A106KE05L\",\n    \"Price per unit\":null,\n    \"Image\":[],\n    \"Source\":\"\",\n    \"Order Items\":[],\n    \"Datasheet\":[],\n    \"Part of a set\":[],\n    \"State\":{\n      \"id\":3001,\n      \"value\":\"Unknown\",\n      \"color\":\"dark-orange\"\n    },\n    \"Part Number\":\"40-00052\",\n    \"Revision\":\"A\",\n    \"Notes\":null,\n    \"Sourced By\":null,\n    \"Containing\":[],\n    \"Contained by\":[]\n  },\n  {\n    \"id\":124,\n    \"order\":\"66.00000000000000000000\",\n    \"Full PN\":\"40-00053 Rev.A\",\n    \"External Part Number\":\"Cap 470µF ±10%\",\n    \"Manufacturer\":[],\n    \"System\":{\n      \"id\":2990,\n      \"value\":\"Amplifier\",\n      \"color\":\"darker-cyan\"\n    },\n    \"Item description\":\"C9, C10\",\n    \"Price per unit\":null,\n    \"Image\":[],\n    \"Source\":\"\",\n    \"Order Items\":[],\n    \"Datasheet\":[],\n    \"Part of a set\":[],\n    \"State\":{\n      \"id\":3001,\n      \"value\":\"Unknown\",\n      \"color\":\"dark-orange\"\n    },\n    \"Part Number\":\"40-00053\",\n    \"Revision\":\"A\",\n    \"Notes\":null,\n    \"Sourced By\":null,\n    \"Containing\":[],\n    \"Contained by\":[]\n  },\n  {\n    \"id\":125,\n    \"order\":\"67.00000000000000000000\",\n    \"Full PN\":\"40-00054 Rev.A\",\n    \"External Part Number\":\"Cap 100nF ±10%\",\n    \"Manufacturer\":[\n      {\n        \"id\":18,\n        \"value\":\"Kemet\",\n        \"order\":\"18.00000000000000000000\"\n      }\n    ],\n    \"System\":{\n      \"id\":2990,\n      \"value\":\"Amplifier\",\n      \"color\":\"darker-cyan\"\n    },\n    \"Item description\":\"C25, C26 C1206C104K1RAC\",\n    \"Price per unit\":\"0.02\",\n    \"Image\":[\n      {\n        \"url\":\"http://localhost/media/user_files/R04i7J3M4femCQZ28nS5PtJfGrg1a0qW_ad233113f6644e2f23e4a88858d8314586f41041bc62fb402f3ba28fbcc64599.avif\",\n        \"thumbnails\":null,\n        \"visible_name\":\"KEMET-C1206C104K1RACTU.avif\",\n        \"name\":\"R04i7J3M4femCQZ28nS5PtJfGrg1a0qW_ad233113f6644e2f23e4a88858d8314586f41041bc62fb402f3ba28fbcc64599.avif\",\n        \"size\":4126,\n        \"mime_type\":\"image/avif\",\n        \"is_image\":false,\n        \"image_width\":null,\n        \"image_height\":null,\n        \"uploaded_at\":\"2025-05-06T09:46:27.671841+00:00\"\n      }\n    ],\n    \"Source\":\"\",\n    \"Order Items\":[],\n    \"Datasheet\":[\n      {\n        \"url\":\"http://localhost/media/user_files/SVVmITdiSgrQKTcL9YixyeDAOzlalM2q_1c6bc2fcb337990900b8ae7ec37e00ec3b663b04b195514ed1dbf69fa3152d48.pdf\",\n        \"thumbnails\":null,\n        \"visible_name\":\"C1206C104K1RACTU.pdf\",\n        \"name\":\"SVVmITdiSgrQKTcL9YixyeDAOzlalM2q_1c6bc2fcb337990900b8ae7ec37e00ec3b663b04b195514ed1dbf69fa3152d48.pdf\",\n        \"size\":1067466,\n        \"mime_type\":\"application/pdf\",\n        \"is_image\":false,\n        \"image_width\":null,\n        \"image_height\":null,\n        \"uploaded_at\":\"2025-05-06T09:47:03.007010+00:00\"\n      }\n    ],\n    \"Part of a set\":[],\n    \"State\":{\n      \"id\":3001,\n      \"value\":\"Unknown\",\n      \"color\":\"dark-orange\"\n    },\n    \"Part Number\":\"40-00054\",\n    \"Revision\":\"A\",\n    \"Notes\":null,\n    \"Sourced By\":null,\n    \"Containing\":[],\n    \"Contained by\":[]\n  },\n  {\n    \"id\":126,\n    \"order\":\"68.00000000000000000000\",\n    \"Full PN\":\"40-00055 Rev.A\",\n    \"External Part Number\":\"Cap 1µF ±10%\",\n    \"Manufacturer\":[\n      {\n        \"id\":18,\n        \"value\":\"Kemet\",\n        \"order\":\"18.00000000000000000000\"\n      }\n    ],\n    \"System\":{\n      \"id\":2990,\n      \"value\":\"Amplifier\",\n      \"color\":\"darker-cyan\"\n    },\n    \"Item description\":\"C27, C28 GRM31MR71E105KA01L\",\n    \"Price per unit\":null,\n    \"Image\":[],\n    \"Source\":\"\",\n    \"Order Items\":[],\n    \"Datasheet\":[],\n    \"Part of a set\":[],\n    \"State\":{\n      \"id\":3001,\n      \"value\":\"Unknown\",\n      \"color\":\"dark-orange\"\n    },\n    \"Part Number\":\"40-00055\",\n    \"Revision\":\"A\",\n    \"Notes\":null,\n    \"Sourced By\":null,\n    \"Containing\":[],\n    \"Contained by\":[]\n  },\n  {\n    \"id\":127,\n    \"order\":\"69.00000000000000000000\",\n    \"Full PN\":\"40-00056 Rev.A\",\n    \"External Part Number\":\"Cap 10µF ±10%\",\n    \"Manufacturer\":[\n      {\n        \"id\":16,\n        \"value\":\"TDK (Capacitors division)\",\n        \"order\":\"16.00000000000000000000\"\n      }\n    ],\n    \"System\":{\n      \"id\":2990,\n      \"value\":\"Amplifier\",\n      \"color\":\"darker-cyan\"\n    },\n    \"Item description\":\"C29, C30 C3216X5R1E106KAC\",\n    \"Price per unit\":null,\n    \"Image\":[],\n    \"Source\":\"\",\n    \"Order Items\":[],\n    \"Datasheet\":[],\n    \"Part of a set\":[],\n    \"State\":{\n      \"id\":3001,\n      \"value\":\"Unknown\",\n      \"color\":\"dark-orange\"\n    },\n    \"Part Number\":\"40-00056\",\n    \"Revision\":\"A\",\n    \"Notes\":null,\n    \"Sourced By\":null,\n    \"Containing\":[],\n    \"Contained by\":[]\n  },\n  {\n    \"id\":128,\n    \"order\":\"70.00000000000000000000\",\n    \"Full PN\":\"40-00057 Rev.A\",\n    \"External Part Number\":\"Resistor 39R ±1%\",\n    \"Manufacturer\":[\n      {\n        \"id\":19,\n        \"value\":\"TE Connectivity\",\n        \"order\":\"19.00000000000000000000\"\n      }\n    ],\n    \"System\":{\n      \"id\":2990,\n      \"value\":\"Amplifier\",\n      \"color\":\"darker-cyan\"\n    },\n    \"Item description\":\"R1, R2, R3, R4 CRGCQ1206F39R\",\n    \"Price per unit\":\"0.10\",\n    \"Image\":[\n      {\n        \"url\":\"http://localhost/media/user_files/sGuwdMm8kC0iYZ4YmFnScGOk4GmPBuIp_d2c4709712019d204d7bff98f9d659b097add8bbc3bd74007b8b49641fb47b19.webp\",\n        \"thumbnails\":{\n          \"tiny\":{\n            \"url\":\"http://localhost/media/thumbnails/tiny/sGuwdMm8kC0iYZ4YmFnScGOk4GmPBuIp_d2c4709712019d204d7bff98f9d659b097add8bbc3bd74007b8b49641fb47b19.webp\",\n            \"width\":null,\n            \"height\":21\n          },\n          \"small\":{\n            \"url\":\"http://localhost/media/thumbnails/small/sGuwdMm8kC0iYZ4YmFnScGOk4GmPBuIp_d2c4709712019d204d7bff98f9d659b097add8bbc3bd74007b8b49641fb47b19.webp\",\n            \"width\":48,\n            \"height\":48\n          },\n          \"card_cover\":{\n            \"url\":\"http://localhost/media/thumbnails/card_cover/sGuwdMm8kC0iYZ4YmFnScGOk4GmPBuIp_d2c4709712019d204d7bff98f9d659b097add8bbc3bd74007b8b49641fb47b19.webp\",\n            \"width\":300,\n            \"height\":160\n          }\n        },\n        \"visible_name\":\"CRGCQ_series_DSL.webp\",\n        \"name\":\"sGuwdMm8kC0iYZ4YmFnScGOk4GmPBuIp_d2c4709712019d204d7bff98f9d659b097add8bbc3bd74007b8b49641fb47b19.webp\",\n        \"size\":1260,\n        \"mime_type\":\"image/webp\",\n        \"is_image\":true,\n        \"image_width\":150,\n        \"image_height\":150,\n        \"uploaded_at\":\"2025-05-06T09:53:56.156703+00:00\"\n      }\n    ],\n    \"Source\":\"\",\n    \"Order Items\":[],\n    \"Datasheet\":[],\n    \"Part of a set\":[],\n    \"State\":{\n      \"id\":3001,\n      \"value\":\"Unknown\",\n      \"color\":\"dark-orange\"\n    },\n    \"Part Number\":\"40-00057\",\n    \"Revision\":\"A\",\n    \"Notes\":null,\n    \"Sourced By\":null,\n    \"Containing\":[],\n    \"Contained by\":[]\n  },\n  {\n    \"id\":129,\n    \"order\":\"71.00000000000000000000\",\n    \"Full PN\":\"40-00058 Rev.A\",\n    \"External Part Number\":\"Coil 95nH\",\n    \"Manufacturer\":[],\n    \"System\":{\n      \"id\":2990,\n      \"value\":\"Amplifier\",\n      \"color\":\"darker-cyan\"\n    },\n    \"Item description\":\"L1, L2 Cu wire d=1.5mm, 3 turns, inner d=9.9mm\",\n    \"Price per unit\":null,\n    \"Image\":[\n      {\n        \"url\":\"http://localhost/media/user_files/olzuAfeaM0AbnsXM1gC7pCBtEbidPSEY_d3371daa1f67b5e057f6137e73fd9e7ad539446ba3ee1e38a9753d7e21cd6350.png\",\n        \"thumbnails\":{\n          \"tiny\":{\n            \"url\":\"http://localhost/media/thumbnails/tiny/olzuAfeaM0AbnsXM1gC7pCBtEbidPSEY_d3371daa1f67b5e057f6137e73fd9e7ad539446ba3ee1e38a9753d7e21cd6350.png\",\n            \"width\":null,\n            \"height\":21\n          },\n          \"small\":{\n            \"url\":\"http://localhost/media/thumbnails/small/olzuAfeaM0AbnsXM1gC7pCBtEbidPSEY_d3371daa1f67b5e057f6137e73fd9e7ad539446ba3ee1e38a9753d7e21cd6350.png\",\n            \"width\":48,\n            \"height\":48\n          },\n          \"card_cover\":{\n            \"url\":\"http://localhost/media/thumbnails/card_cover/olzuAfeaM0AbnsXM1gC7pCBtEbidPSEY_d3371daa1f67b5e057f6137e73fd9e7ad539446ba3ee1e38a9753d7e21cd6350.png\",\n            \"width\":300,\n            \"height\":160\n          }\n        },\n        \"visible_name\":\"image.png\",\n        \"name\":\"olzuAfeaM0AbnsXM1gC7pCBtEbidPSEY_d3371daa1f67b5e057f6137e73fd9e7ad539446ba3ee1e38a9753d7e21cd6350.png\",\n        \"size\":47675,\n        \"mime_type\":\"image/png\",\n        \"is_image\":true,\n        \"image_width\":119,\n        \"image_height\":166,\n        \"uploaded_at\":\"2025-05-06T09:58:04.416265+00:00\"\n      }\n    ],\n    \"Source\":\"\",\n    \"Order Items\":[],\n    \"Datasheet\":[],\n    \"Part of a set\":[],\n    \"State\":{\n      \"id\":3001,\n      \"value\":\"Unknown\",\n      \"color\":\"dark-orange\"\n    },\n    \"Part Number\":\"40-00058\",\n    \"Revision\":\"A\",\n    \"Notes\":null,\n    \"Sourced By\":null,\n    \"Containing\":[],\n    \"Contained by\":[]\n  },\n  {\n    \"id\":130,\n    \"order\":\"72.00000000000000000000\",\n    \"Full PN\":\"40-00059 Rev.A\",\n    \"External Part Number\":\"Coil 47nH ±5%\",\n    \"Manufacturer\":[\n      {\n        \"id\":20,\n        \"value\":\"Coilcraft\",\n        \"order\":\"20.00000000000000000000\"\n      }\n    ],\n    \"System\":{\n      \"id\":2990,\n      \"value\":\"Amplifier\",\n      \"color\":\"darker-cyan\"\n    },\n    \"Item description\":\"L3, L4 1206CS-470XJE\",\n    \"Price per unit\":\"0.94\",\n    \"Image\":[\n      {\n        \"url\":\"http://localhost/media/user_files/fI9ZrhLt91DAaQEjEu3k0sPGjKQkIRVq_fc45d3e8f9e7e495e37f4680e093bb6e7a16d6f4e175b33c65dfb733d6cac21e.jpg\",\n        \"thumbnails\":{\n          \"tiny\":{\n            \"url\":\"http://localhost/media/thumbnails/tiny/fI9ZrhLt91DAaQEjEu3k0sPGjKQkIRVq_fc45d3e8f9e7e495e37f4680e093bb6e7a16d6f4e175b33c65dfb733d6cac21e.jpg\",\n            \"width\":null,\n            \"height\":21\n          },\n          \"small\":{\n            \"url\":\"http://localhost/media/thumbnails/small/fI9ZrhLt91DAaQEjEu3k0sPGjKQkIRVq_fc45d3e8f9e7e495e37f4680e093bb6e7a16d6f4e175b33c65dfb733d6cac21e.jpg\",\n            \"width\":48,\n            \"height\":48\n          },\n          \"card_cover\":{\n            \"url\":\"http://localhost/media/thumbnails/card_cover/fI9ZrhLt91DAaQEjEu3k0sPGjKQkIRVq_fc45d3e8f9e7e495e37f4680e093bb6e7a16d6f4e175b33c65dfb733d6cac21e.jpg\",\n            \"width\":300,\n            \"height\":160\n          }\n        },\n        \"visible_name\":\"1206cs_dim.jpg\",\n        \"name\":\"fI9ZrhLt91DAaQEjEu3k0sPGjKQkIRVq_fc45d3e8f9e7e495e37f4680e093bb6e7a16d6f4e175b33c65dfb733d6cac21e.jpg\",\n        \"size\":28140,\n        \"mime_type\":\"image/jpeg\",\n        \"is_image\":true,\n        \"image_width\":250,\n        \"image_height\":250,\n        \"uploaded_at\":\"2025-05-06T10:02:11.416092+00:00\"\n      }\n    ],\n    \"Source\":\"https://www.coilcraft.com/en-us/products/rf/ceramic-core-chip-inductors/1206-(3216)/1206cs/1206cs-470/?srsltid=AfmBOoqT6QFQAeUo78Tt_Om7OhLaoopEGJKLwefrUdbUX9Ch30krvT2K\",\n    \"Order Items\":[],\n    \"Datasheet\":[\n      {\n        \"url\":\"http://localhost/media/user_files/p20MPuY5Yu2ua2U2FmuZaPRnw0l6EFvh_f5616f4d2c782ba4903d5ba2ded54e5757a757af98fd91d2a79aff9f7633ed80.pdf\",\n        \"thumbnails\":null,\n        \"visible_name\":\"1206cs.pdf\",\n        \"name\":\"p20MPuY5Yu2ua2U2FmuZaPRnw0l6EFvh_f5616f4d2c782ba4903d5ba2ded54e5757a757af98fd91d2a79aff9f7633ed80.pdf\",\n        \"size\":132760,\n        \"mime_type\":\"application/pdf\",\n        \"is_image\":false,\n        \"image_width\":null,\n        \"image_height\":null,\n        \"uploaded_at\":\"2025-05-06T10:02:37.613046+00:00\"\n      }\n    ],\n    \"Part of a set\":[],\n    \"State\":{\n      \"id\":3001,\n      \"value\":\"Unknown\",\n      \"color\":\"dark-orange\"\n    },\n    \"Part Number\":\"40-00059\",\n    \"Revision\":\"A\",\n    \"Notes\":null,\n    \"Sourced By\":null,\n    \"Containing\":[],\n    \"Contained by\":[]\n  },\n  {\n    \"id\":131,\n    \"order\":\"73.00000000000000000000\",\n    \"Full PN\":\"40-00060 Rev.A\",\n    \"External Part Number\":\"Cap 470pF ±5%\",\n    \"Manufacturer\":[\n      {\n        \"id\":15,\n        \"value\":\"AVX (Kyocera)\",\n        \"order\":\"15.00000000000000000000\"\n      }\n    ],\n    \"System\":{\n      \"id\":2990,\n      \"value\":\"Amplifier\",\n      \"color\":\"darker-cyan\"\n    },\n    \"Item description\":\"C31, C32, C36 800B471JW500X\",\n    \"Price per unit\":null,\n    \"Image\":[],\n    \"Source\":\"\",\n    \"Order Items\":[],\n    \"Datasheet\":[],\n    \"Part of a set\":[],\n    \"State\":{\n      \"id\":3001,\n      \"value\":\"Unknown\",\n      \"color\":\"dark-orange\"\n    },\n    \"Part Number\":\"40-00060\",\n    \"Revision\":\"A\",\n    \"Notes\":null,\n    \"Sourced By\":null,\n    \"Containing\":[],\n    \"Contained by\":[]\n  },\n  {\n    \"id\":132,\n    \"order\":\"74.00000000000000000000\",\n    \"Full PN\":\"40-00061 Rev.A\",\n    \"External Part Number\":\"Cap 30pF ±5%\",\n    \"Manufacturer\":[\n      {\n        \"id\":15,\n        \"value\":\"AVX (Kyocera)\",\n        \"order\":\"15.00000000000000000000\"\n      }\n    ],\n    \"System\":{\n      \"id\":2990,\n      \"value\":\"Amplifier\",\n      \"color\":\"darker-cyan\"\n    },\n    \"Item description\":\"C11 800B471JW500X\",\n    \"Price per unit\":null,\n    \"Image\":[],\n    \"Source\":\"\",\n    \"Order Items\":[],\n    \"Datasheet\":[],\n    \"Part of a set\":[],\n    \"State\":{\n      \"id\":3001,\n      \"value\":\"Unknown\",\n      \"color\":\"dark-orange\"\n    },\n    \"Part Number\":\"40-00061\",\n    \"Revision\":\"A\",\n    \"Notes\":null,\n    \"Sourced By\":null,\n    \"Containing\":[],\n    \"Contained by\":[]\n  },\n  {\n    \"id\":133,\n    \"order\":\"75.00000000000000000000\",\n    \"Full PN\":\"40-00062 Rev.A\",\n    \"External Part Number\":\"Cap 390pF ±5%\",\n    \"Manufacturer\":[\n      {\n        \"id\":15,\n        \"value\":\"AVX (Kyocera)\",\n        \"order\":\"15.00000000000000000000\"\n      }\n    ],\n    \"System\":{\n      \"id\":2990,\n      \"value\":\"Amplifier\",\n      \"color\":\"darker-cyan\"\n    },\n    \"Item description\":\"C12, C13, C14, C15 800B471JW500X\",\n    \"Price per unit\":null,\n    \"Image\":[],\n    \"Source\":\"\",\n    \"Order Items\":[],\n    \"Datasheet\":[],\n    \"Part of a set\":[],\n    \"State\":{\n      \"id\":3001,\n      \"value\":\"Unknown\",\n      \"color\":\"dark-orange\"\n    },\n    \"Part Number\":\"40-00062\",\n    \"Revision\":\"A\",\n    \"Notes\":null,\n    \"Sourced By\":null,\n    \"Containing\":[],\n    \"Contained by\":[]\n  },\n  {\n    \"id\":134,\n    \"order\":\"76.00000000000000000000\",\n    \"Full PN\":\"40-00063 Rev.A\",\n    \"External Part Number\":\"Cap 270pF ±5%\",\n    \"Manufacturer\":[\n      {\n        \"id\":21,\n        \"value\":\"Cornell Dubilier\",\n        \"order\":\"21.00000000000000000000\"\n      }\n    ],\n    \"System\":{\n      \"id\":2990,\n      \"value\":\"Amplifier\",\n      \"color\":\"darker-cyan\"\n    },\n    \"Item description\":\"C16 MCM01-009EF271J-F\",\n    \"Price per unit\":\"9.93\",\n    \"Image\":[\n      {\n        \"url\":\"http://localhost/media/user_files/PxFw9ZVWNVqYDGS9FX7HlyEiHF0PVVGR_c43efb1d51cd507e4629c06f6b1e79e817a1764d474ec18926298362cb5637aa.webp\",\n        \"thumbnails\":{\n          \"tiny\":{\n            \"url\":\"http://localhost/media/thumbnails/tiny/PxFw9ZVWNVqYDGS9FX7HlyEiHF0PVVGR_c43efb1d51cd507e4629c06f6b1e79e817a1764d474ec18926298362cb5637aa.webp\",\n            \"width\":null,\n            \"height\":21\n          },\n          \"small\":{\n            \"url\":\"http://localhost/media/thumbnails/small/PxFw9ZVWNVqYDGS9FX7HlyEiHF0PVVGR_c43efb1d51cd507e4629c06f6b1e79e817a1764d474ec18926298362cb5637aa.webp\",\n            \"width\":48,\n            \"height\":48\n          },\n          \"card_cover\":{\n            \"url\":\"http://localhost/media/thumbnails/card_cover/PxFw9ZVWNVqYDGS9FX7HlyEiHF0PVVGR_c43efb1d51cd507e4629c06f6b1e79e817a1764d474ec18926298362cb5637aa.webp\",\n            \"width\":300,\n            \"height\":160\n          }\n        },\n        \"visible_name\":\"MCM - MIN 300 CMYK.webp\",\n        \"name\":\"PxFw9ZVWNVqYDGS9FX7HlyEiHF0PVVGR_c43efb1d51cd507e4629c06f6b1e79e817a1764d474ec18926298362cb5637aa.webp\",\n        \"size\":2240,\n        \"mime_type\":\"image/webp\",\n        \"is_image\":true,\n        \"image_width\":150,\n        \"image_height\":145,\n        \"uploaded_at\":\"2025-05-06T10:22:03.969508+00:00\"\n      }\n    ],\n    \"Source\":\"https://www.mouser.com/ProductDetail/Cornell-Dubilier-CDE/MCM01-009EF271J-F?qs=eA5gmb%2FfgdQb0G31JRdxHA%3D%3D&srsltid=AfmBOoq4OVh5wqJJhuTQjq5kHVW2NR2sJxYaAqMZxLtCbSaacJdEhxu6\",\n    \"Order Items\":[],\n    \"Datasheet\":[\n      {\n        \"url\":\"http://localhost/media/user_files/p3XEuuv59umeGeH70MdwFkkZRLnlWwQ3_3c9c6f6358a4ccadc351284243e7516085f0201a1f0a0c1bcc24876981a9d8cd.pdf\",\n        \"thumbnails\":null,\n        \"visible_name\":\"MCM-MIN.pdf\",\n        \"name\":\"p3XEuuv59umeGeH70MdwFkkZRLnlWwQ3_3c9c6f6358a4ccadc351284243e7516085f0201a1f0a0c1bcc24876981a9d8cd.pdf\",\n        \"size\":803433,\n        \"mime_type\":\"application/pdf\",\n        \"is_image\":false,\n        \"image_width\":null,\n        \"image_height\":null,\n        \"uploaded_at\":\"2025-05-06T10:22:51.855052+00:00\"\n      }\n    ],\n    \"Part of a set\":[],\n    \"State\":{\n      \"id\":3001,\n      \"value\":\"Unknown\",\n      \"color\":\"dark-orange\"\n    },\n    \"Part Number\":\"40-00063\",\n    \"Revision\":\"A\",\n    \"Notes\":null,\n    \"Sourced By\":null,\n    \"Containing\":[],\n    \"Contained by\":[]\n  },\n  {\n    \"id\":135,\n    \"order\":\"77.00000000000000000000\",\n    \"Full PN\":\"40-00064 Rev.A\",\n    \"External Part Number\":\"Cap 270pF  ±5%\",\n    \"Manufacturer\":[\n      {\n        \"id\":15,\n        \"value\":\"AVX (Kyocera)\",\n        \"order\":\"15.00000000000000000000\"\n      }\n    ],\n    \"System\":{\n      \"id\":2990,\n      \"value\":\"Amplifier\",\n      \"color\":\"darker-cyan\"\n    },\n    \"Item description\":\"C17 800B271JW500X\",\n    \"Price per unit\":null,\n    \"Image\":[],\n    \"Source\":\"\",\n    \"Order Items\":[],\n    \"Datasheet\":[],\n    \"Part of a set\":[],\n    \"State\":{\n      \"id\":3001,\n      \"value\":\"Unknown\",\n      \"color\":\"dark-orange\"\n    },\n    \"Part Number\":\"40-00064\",\n    \"Revision\":\"A\",\n    \"Notes\":null,\n    \"Sourced By\":null,\n    \"Containing\":[],\n    \"Contained by\":[]\n  },\n  {\n    \"id\":137,\n    \"order\":\"77.50000000000000000000\",\n    \"Full PN\":\"40-00065 Rev.A\",\n    \"External Part Number\":\"Cap 200pF  ±5%\",\n    \"Manufacturer\":[\n      {\n        \"id\":15,\n        \"value\":\"AVX (Kyocera)\",\n        \"order\":\"15.00000000000000000000\"\n      }\n    ],\n    \"System\":{\n      \"id\":2990,\n      \"value\":\"Amplifier\",\n      \"color\":\"darker-cyan\"\n    },\n    \"Item description\":\"C18 800B271JW500X\",\n    \"Price per unit\":null,\n    \"Image\":[],\n    \"Source\":\"\",\n    \"Order Items\":[],\n    \"Datasheet\":[],\n    \"Part of a set\":[],\n    \"State\":{\n      \"id\":3001,\n      \"value\":\"Unknown\",\n      \"color\":\"dark-orange\"\n    },\n    \"Part Number\":\"40-00065\",\n    \"Revision\":\"A\",\n    \"Notes\":null,\n    \"Sourced By\":null,\n    \"Containing\":[],\n    \"Contained by\":[]\n  },\n  {\n    \"id\":138,\n    \"order\":\"77.66666666666667140362\",\n    \"Full PN\":\"40-00066 Rev.A\",\n    \"External Part Number\":\"Cap 360pF  ±5%\",\n    \"Manufacturer\":[\n      {\n        \"id\":15,\n        \"value\":\"AVX (Kyocera)\",\n        \"order\":\"15.00000000000000000000\"\n      }\n    ],\n    \"System\":{\n      \"id\":2990,\n      \"value\":\"Amplifier\",\n      \"color\":\"darker-cyan\"\n    },\n    \"Item description\":\"C33 800B271JW500X\",\n    \"Price per unit\":null,\n    \"Image\":[],\n    \"Source\":\"\",\n    \"Order Items\":[],\n    \"Datasheet\":[],\n    \"Part of a set\":[],\n    \"State\":{\n      \"id\":3001,\n      \"value\":\"Unknown\",\n      \"color\":\"dark-orange\"\n    },\n    \"Part Number\":\"40-00066\",\n    \"Revision\":\"A\",\n    \"Notes\":null,\n    \"Sourced By\":null,\n    \"Containing\":[],\n    \"Contained by\":[]\n  },\n  {\n    \"id\":139,\n    \"order\":\"77.75000000000000000000\",\n    \"Full PN\":\"40-00067 Rev.A\",\n    \"External Part Number\":\"Cap 180pF  ±5%\",\n    \"Manufacturer\":[\n      {\n        \"id\":15,\n        \"value\":\"AVX (Kyocera)\",\n        \"order\":\"15.00000000000000000000\"\n      }\n    ],\n    \"System\":{\n      \"id\":2990,\n      \"value\":\"Amplifier\",\n      \"color\":\"darker-cyan\"\n    },\n    \"Item description\":\"C34 800B271JW500X\",\n    \"Price per unit\":null,\n    \"Image\":[],\n    \"Source\":\"\",\n    \"Order Items\":[],\n    \"Datasheet\":[],\n    \"Part of a set\":[],\n    \"State\":{\n      \"id\":3001,\n      \"value\":\"Unknown\",\n      \"color\":\"dark-orange\"\n    },\n    \"Part Number\":\"40-00067\",\n    \"Revision\":\"A\",\n    \"Notes\":null,\n    \"Sourced By\":null,\n    \"Containing\":[],\n    \"Contained by\":[]\n  },\n  {\n    \"id\":140,\n    \"order\":\"77.79999999999999715783\",\n    \"Full PN\":\"40-00068 Rev.A\",\n    \"External Part Number\":\"Cap 82pF  ±5%\",\n    \"Manufacturer\":[\n      {\n        \"id\":15,\n        \"value\":\"AVX (Kyocera)\",\n        \"order\":\"15.00000000000000000000\"\n      }\n    ],\n    \"System\":{\n      \"id\":2990,\n      \"value\":\"Amplifier\",\n      \"color\":\"darker-cyan\"\n    },\n    \"Item description\":\"C35 800B271JW500X\",\n    \"Price per unit\":null,\n    \"Image\":[],\n    \"Source\":\"\",\n    \"Order Items\":[],\n    \"Datasheet\":[],\n    \"Part of a set\":[],\n    \"State\":{\n      \"id\":3001,\n      \"value\":\"Unknown\",\n      \"color\":\"dark-orange\"\n    },\n    \"Part Number\":\"40-00068\",\n    \"Revision\":\"A\",\n    \"Notes\":null,\n    \"Sourced By\":null,\n    \"Containing\":[],\n    \"Contained by\":[]\n  },\n  {\n    \"id\":141,\n    \"order\":\"77.83333333333332859638\",\n    \"Full PN\":\"40-00069 Rev.A\",\n    \"External Part Number\":\"Cap 750pF  ±5%\",\n    \"Manufacturer\":[\n      {\n        \"id\":15,\n        \"value\":\"AVX (Kyocera)\",\n        \"order\":\"15.00000000000000000000\"\n      }\n    ],\n    \"System\":{\n      \"id\":2990,\n      \"value\":\"Amplifier\",\n      \"color\":\"darker-cyan\"\n    },\n    \"Item description\":\"C19 800B271JW500X\",\n    \"Price per unit\":null,\n    \"Image\":[],\n    \"Source\":\"\",\n    \"Order Items\":[],\n    \"Datasheet\":[],\n    \"Part of a set\":[],\n    \"State\":{\n      \"id\":3001,\n      \"value\":\"Unknown\",\n      \"color\":\"dark-orange\"\n    },\n    \"Part Number\":\"40-00069\",\n    \"Revision\":\"A\",\n    \"Notes\":null,\n    \"Sourced By\":null,\n    \"Containing\":[],\n    \"Contained by\":[]\n  },\n  {\n    \"id\":142,\n    \"order\":\"77.85714285714286120310\",\n    \"Full PN\":\"40-00070 Rev.A\",\n    \"External Part Number\":\"Cap 20pF  ±5%\",\n    \"Manufacturer\":[\n      {\n        \"id\":15,\n        \"value\":\"AVX (Kyocera)\",\n        \"order\":\"15.00000000000000000000\"\n      }\n    ],\n    \"System\":{\n      \"id\":2990,\n      \"value\":\"Amplifier\",\n      \"color\":\"darker-cyan\"\n    },\n    \"Item description\":\"C20 800B271JW500X\",\n    \"Price per unit\":null,\n    \"Image\":[],\n    \"Source\":\"\",\n    \"Order Items\":[],\n    \"Datasheet\":[],\n    \"Part of a set\":[],\n    \"State\":{\n      \"id\":3001,\n      \"value\":\"Unknown\",\n      \"color\":\"dark-orange\"\n    },\n    \"Part Number\":\"40-00070\",\n    \"Revision\":\"A\",\n    \"Notes\":null,\n    \"Sourced By\":null,\n    \"Containing\":[],\n    \"Contained by\":[]\n  },\n  {\n    \"id\":136,\n    \"order\":\"78.00000000000000000000\",\n    \"Full PN\":\"40-00071 Rev.A\",\n    \"External Part Number\":\"Coil 9.5nH\",\n    \"Manufacturer\":[],\n    \"System\":{\n      \"id\":2990,\n      \"value\":\"Amplifier\",\n      \"color\":\"darker-cyan\"\n    },\n    \"Item description\":\"L5, L6 Cu wire d=1.5mm, 1 turn, inner d=9.9mm\",\n    \"Price per unit\":null,\n    \"Image\":[],\n    \"Source\":\"\",\n    \"Order Items\":[],\n    \"Datasheet\":[],\n    \"Part of a set\":[],\n    \"State\":{\n      \"id\":3001,\n      \"value\":\"Unknown\",\n      \"color\":\"dark-orange\"\n    },\n    \"Part Number\":\"40-00071\",\n    \"Revision\":\"A\",\n    \"Notes\":null,\n    \"Sourced By\":null,\n    \"Containing\":[],\n    \"Contained by\":[]\n  },\n  {\n    \"id\":144,\n    \"order\":\"79.00000000000000000000\",\n    \"Full PN\":\"40-00072 Rev.A\",\n    \"External Part Number\":\"Transistor\",\n    \"Manufacturer\":[\n      {\n        \"id\":22,\n        \"value\":\"Ampleon\",\n        \"order\":\"22.00000000000000000000\"\n      }\n    ],\n    \"System\":{\n      \"id\":2990,\n      \"value\":\"Amplifier\",\n      \"color\":\"darker-cyan\"\n    },\n    \"Item description\":\"Q1 ART450FE\",\n    \"Price per unit\":null,\n    \"Image\":[],\n    \"Source\":\"\",\n    \"Order Items\":[],\n    \"Datasheet\":[],\n    \"Part of a set\":[],\n    \"State\":{\n      \"id\":3001,\n      \"value\":\"Unknown\",\n      \"color\":\"dark-orange\"\n    },\n    \"Part Number\":\"40-00072\",\n    \"Revision\":\"A\",\n    \"Notes\":null,\n    \"Sourced By\":null,\n    \"Containing\":[],\n    \"Contained by\":[]\n  },\n  {\n    \"id\":177,\n    \"order\":\"80.00000000000000000000\",\n    \"Full PN\":\"10-00000 Rev.A\",\n    \"External Part Number\":\"6000K Cold White LED strip\",\n    \"Manufacturer\":[\n      {\n        \"id\":55,\n        \"value\":\"Epistar\",\n        \"order\":\"23.00000000000000000000\"\n      }\n    ],\n    \"System\":{\n      \"id\":2992,\n      \"value\":\"Main Body Assembly\",\n      \"color\":\"darker-gray\"\n    },\n    \"Item description\":\"15W 24V 6000K 120LED/m IP20 1550Lumen\",\n    \"Price per unit\":\"10.04\",\n    \"Image\":[\n      {\n        \"url\":\"http://localhost/media/user_files/P92OMVlecTwckg2ZdUuQY9gxBENVSSIi_df15488b9454efd53c80ea0120bf47e690217a95f3696154c1c5226b0d7df7fc.png\",\n        \"thumbnails\":{\n          \"tiny\":{\n            \"url\":\"http://localhost/media/thumbnails/tiny/P92OMVlecTwckg2ZdUuQY9gxBENVSSIi_df15488b9454efd53c80ea0120bf47e690217a95f3696154c1c5226b0d7df7fc.png\",\n            \"width\":null,\n            \"height\":21\n          },\n          \"small\":{\n            \"url\":\"http://localhost/media/thumbnails/small/P92OMVlecTwckg2ZdUuQY9gxBENVSSIi_df15488b9454efd53c80ea0120bf47e690217a95f3696154c1c5226b0d7df7fc.png\",\n            \"width\":48,\n            \"height\":48\n          },\n          \"card_cover\":{\n            \"url\":\"http://localhost/media/thumbnails/card_cover/P92OMVlecTwckg2ZdUuQY9gxBENVSSIi_df15488b9454efd53c80ea0120bf47e690217a95f3696154c1c5226b0d7df7fc.png\",\n            \"width\":300,\n            \"height\":160\n          }\n        },\n        \"visible_name\":\"image.png\",\n        \"name\":\"P92OMVlecTwckg2ZdUuQY9gxBENVSSIi_df15488b9454efd53c80ea0120bf47e690217a95f3696154c1c5226b0d7df7fc.png\",\n        \"size\":130985,\n        \"mime_type\":\"image/png\",\n        \"is_image\":true,\n        \"image_width\":458,\n        \"image_height\":217,\n        \"uploaded_at\":\"2025-06-05T07:02:18.677410+00:00\"\n      }\n    ],\n    \"Source\":\"https://enerled.co.il/product/%d7%a4%d7%a1-%d7%9c%d7%93%d7%99%d7%9d-2835-%d7%94%d7%a1%d7%a4%d7%a7-19w-%d7%9e%d7%aa%d7%97-24v-%d7%aa%d7%a0%d7%90%d7%99-%d7%a4%d7%a0%d7%99%d7%9d/\",\n    \"Order Items\":[],\n    \"Datasheet\":[],\n    \"Part of a set\":[],\n    \"State\":{\n      \"id\":3001,\n      \"value\":\"Unknown\",\n      \"color\":\"dark-orange\"\n    },\n    \"Part Number\":\"10-00000\",\n    \"Revision\":\"A\",\n    \"Notes\":null,\n    \"Sourced By\":null,\n    \"Containing\":[],\n    \"Contained by\":[]\n  },\n  {\n    \"id\":179,\n    \"order\":\"82.00000000000000000000\",\n    \"Full PN\":\"20-00020 Rev.A\",\n    \"External Part Number\":\"JSX-1065\",\n    \"Manufacturer\":[\n      {\n        \"id\":57,\n        \"value\":\"Kycon, Inc.\",\n        \"order\":\"25.00000000000000000000\"\n      }\n    ],\n    \"System\":{\n      \"id\":2993,\n      \"value\":\"Controller\",\n      \"color\":\"darker-green\"\n    },\n    \"Item description\":\"6.5mm 4-40(~M3) Jackscrew(Standoff) For D-Sub Connectors\",\n    \"Price per unit\":\"0.37\",\n    \"Image\":[\n      {\n        \"url\":\"http://localhost/media/user_files/FRn1yGODkJN7mR4GObamkbymbmaxS9Sm_ca2e8a13b1c1bdd9b1d94128fecedb32dd2e75242b3451daea17c03211d48dca.png\",\n        \"thumbnails\":{\n          \"tiny\":{\n            \"url\":\"http://localhost/media/thumbnails/tiny/FRn1yGODkJN7mR4GObamkbymbmaxS9Sm_ca2e8a13b1c1bdd9b1d94128fecedb32dd2e75242b3451daea17c03211d48dca.png\",\n            \"width\":null,\n            \"height\":21\n          },\n          \"small\":{\n            \"url\":\"http://localhost/media/thumbnails/small/FRn1yGODkJN7mR4GObamkbymbmaxS9Sm_ca2e8a13b1c1bdd9b1d94128fecedb32dd2e75242b3451daea17c03211d48dca.png\",\n            \"width\":48,\n            \"height\":48\n          },\n          \"card_cover\":{\n            \"url\":\"http://localhost/media/thumbnails/card_cover/FRn1yGODkJN7mR4GObamkbymbmaxS9Sm_ca2e8a13b1c1bdd9b1d94128fecedb32dd2e75242b3451daea17c03211d48dca.png\",\n            \"width\":300,\n            \"height\":160\n          }\n        },\n        \"visible_name\":\"image.png\",\n        \"name\":\"FRn1yGODkJN7mR4GObamkbymbmaxS9Sm_ca2e8a13b1c1bdd9b1d94128fecedb32dd2e75242b3451daea17c03211d48dca.png\",\n        \"size\":10234,\n        \"mime_type\":\"image/png\",\n        \"is_image\":true,\n        \"image_width\":200,\n        \"image_height\":200,\n        \"uploaded_at\":\"2025-06-09T11:36:42.634914+00:00\"\n      }\n    ],\n    \"Source\":\"https://www.digikey.co.il/en/products/detail/kycon-inc/JSX-1065/12809958\",\n    \"Order Items\":[],\n    \"Datasheet\":[\n      {\n        \"url\":\"http://localhost/media/user_files/0XRfhozurgQF0leTBS5xP2KmItyHRlEH_23e73fede45c381d3ebfdc30bf9dcd917401f36e2c10d33c9f83f8ece6e65807.pdf\",\n        \"thumbnails\":null,\n        \"visible_name\":\"JSX-1065.pdf\",\n        \"name\":\"0XRfhozurgQF0leTBS5xP2KmItyHRlEH_23e73fede45c381d3ebfdc30bf9dcd917401f36e2c10d33c9f83f8ece6e65807.pdf\",\n        \"size\":112771,\n        \"mime_type\":\"application/pdf\",\n        \"is_image\":false,\n        \"image_width\":null,\n        \"image_height\":null,\n        \"uploaded_at\":\"2025-06-09T11:35:24.264761+00:00\"\n      }\n    ],\n    \"Part of a set\":[],\n    \"State\":{\n      \"id\":3001,\n      \"value\":\"Unknown\",\n      \"color\":\"dark-orange\"\n    },\n    \"Part Number\":\"20-00020\",\n    \"Revision\":\"A\",\n    \"Notes\":null,\n    \"Sourced By\":null,\n    \"Containing\":[],\n    \"Contained by\":[]\n  },\n  {\n    \"id\":182,\n    \"order\":\"85.00000000000000000000\",\n    \"Full PN\":\"20-00021 Rev.A\",\n    \"External Part Number\":\"40-9709HS\",\n    \"Manufacturer\":[\n      {\n        \"id\":59,\n        \"value\":\"Cinch Connectivity Solutions AIM-Cambridge\",\n        \"order\":\"27.00000000000000000000\"\n      }\n    ],\n    \"System\":{\n      \"id\":2993,\n      \"value\":\"Controller\",\n      \"color\":\"darker-green\"\n    },\n    \"Item description\":\"9 Position Two Piece Backshell Connector Chrome 180° Shielded\",\n    \"Price per unit\":\"1.50\",\n    \"Image\":[\n      {\n        \"url\":\"http://localhost/media/user_files/2MJmTQGmyN3b0HrnetWrpzHLScQGVslD_3145166edb7258f927ab08c789118f8d400f6f2a3f9513bb5bf5d147c71701f0.png\",\n        \"thumbnails\":{\n          \"tiny\":{\n            \"url\":\"http://localhost/media/thumbnails/tiny/2MJmTQGmyN3b0HrnetWrpzHLScQGVslD_3145166edb7258f927ab08c789118f8d400f6f2a3f9513bb5bf5d147c71701f0.png\",\n            \"width\":null,\n            \"height\":21\n          },\n          \"small\":{\n            \"url\":\"http://localhost/media/thumbnails/small/2MJmTQGmyN3b0HrnetWrpzHLScQGVslD_3145166edb7258f927ab08c789118f8d400f6f2a3f9513bb5bf5d147c71701f0.png\",\n            \"width\":48,\n            \"height\":48\n          },\n          \"card_cover\":{\n            \"url\":\"http://localhost/media/thumbnails/card_cover/2MJmTQGmyN3b0HrnetWrpzHLScQGVslD_3145166edb7258f927ab08c789118f8d400f6f2a3f9513bb5bf5d147c71701f0.png\",\n            \"width\":300,\n            \"height\":160\n          }\n        },\n        \"visible_name\":\"image.png\",\n        \"name\":\"2MJmTQGmyN3b0HrnetWrpzHLScQGVslD_3145166edb7258f927ab08c789118f8d400f6f2a3f9513bb5bf5d147c71701f0.png\",\n        \"size\":60920,\n        \"mime_type\":\"image/png\",\n        \"is_image\":true,\n        \"image_width\":200,\n        \"image_height\":200,\n        \"uploaded_at\":\"2025-06-09T12:02:37.683427+00:00\"\n      }\n    ],\n    \"Source\":\"https://www.digikey.co.il/en/products/detail/cinch-connectivity-solutions/40-9709HS/3830343\",\n    \"Order Items\":[],\n    \"Datasheet\":[\n      {\n        \"url\":\"http://localhost/media/user_files/jL7KBUpBJk8EfdDxQ6I4f3gSHHLzcA8h_05d44e80eeec6ddf61d58d2d3c384f47bb243381c35123ae03e1b64d581bd1c9.pdf\",\n        \"thumbnails\":null,\n        \"visible_name\":\"dr-ccs-aim-40-9709h.pdf\",\n        \"name\":\"jL7KBUpBJk8EfdDxQ6I4f3gSHHLzcA8h_05d44e80eeec6ddf61d58d2d3c384f47bb243381c35123ae03e1b64d581bd1c9.pdf\",\n        \"size\":670918,\n        \"mime_type\":\"application/pdf\",\n        \"is_image\":false,\n        \"image_width\":null,\n        \"image_height\":null,\n        \"uploaded_at\":\"2025-06-09T12:02:53.460245+00:00\"\n      }\n    ],\n    \"Part of a set\":[],\n    \"State\":{\n      \"id\":3004,\n      \"value\":\"Not Used\",\n      \"color\":\"darker-red\"\n    },\n    \"Part Number\":\"20-00021\",\n    \"Revision\":\"A\",\n    \"Notes\":null,\n    \"Sourced By\":null,\n    \"Containing\":[],\n    \"Contained by\":[]\n  },\n  {\n    \"id\":184,\n    \"order\":\"87.00000000000000000000\",\n    \"Full PN\":\"40-00011 Rev.A\",\n    \"External Part Number\":\"FCE17A15SA450\",\n    \"Manufacturer\":[\n      {\n        \"id\":60,\n        \"value\":\"Amphenol ICC (Commercial Products)\",\n        \"order\":\"28.00000000000000000000\"\n      }\n    ],\n    \"System\":{\n      \"id\":2993,\n      \"value\":\"Controller\",\n      \"color\":\"darker-green\"\n    },\n    \"Item description\":\"CONN D-SUB RCPT 15POS R/A SOLDER FILTERED\",\n    \"Price per unit\":\"22.00\",\n    \"Image\":[\n      {\n        \"url\":\"http://localhost/media/user_files/plwVXl73DDYWadeCGNXSsbsPPbnpRxiO_927859d9451e1e9fdf7bf7c05a41522fdaca180f93ec0d35a3206bd95f415276.jpeg\",\n        \"thumbnails\":{\n          \"tiny\":{\n            \"url\":\"http://localhost/media/thumbnails/tiny/plwVXl73DDYWadeCGNXSsbsPPbnpRxiO_927859d9451e1e9fdf7bf7c05a41522fdaca180f93ec0d35a3206bd95f415276.jpeg\",\n            \"width\":null,\n            \"height\":21\n          },\n          \"small\":{\n            \"url\":\"http://localhost/media/thumbnails/small/plwVXl73DDYWadeCGNXSsbsPPbnpRxiO_927859d9451e1e9fdf7bf7c05a41522fdaca180f93ec0d35a3206bd95f415276.jpeg\",\n            \"width\":48,\n            \"height\":48\n          },\n          \"card_cover\":{\n            \"url\":\"http://localhost/media/thumbnails/card_cover/plwVXl73DDYWadeCGNXSsbsPPbnpRxiO_927859d9451e1e9fdf7bf7c05a41522fdaca180f93ec0d35a3206bd95f415276.jpeg\",\n            \"width\":300,\n            \"height\":160\n          }\n        },\n        \"visible_name\":\"FCE17-A15SA-450.jpeg\",\n        \"name\":\"plwVXl73DDYWadeCGNXSsbsPPbnpRxiO_927859d9451e1e9fdf7bf7c05a41522fdaca180f93ec0d35a3206bd95f415276.jpeg\",\n        \"size\":148105,\n        \"mime_type\":\"image/jpeg\",\n        \"is_image\":true,\n        \"image_width\":640,\n        \"image_height\":640,\n        \"uploaded_at\":\"2025-06-22T07:58:12.526579+00:00\"\n      }\n    ],\n    \"Source\":\"https://www.digikey.co.il/en/products/detail/amphenol-cs-commercial-products/FCE17A15SA450/1968930\",\n    \"Order Items\":[\n      {\n        \"id\":33,\n        \"value\":\"e648f54b-63c3-40b0-823f-19daafe2fd84\",\n        \"order\":\"28.00000000000000000000\"\n      }\n    ],\n    \"Datasheet\":[\n      {\n        \"url\":\"http://localhost/media/user_files/Q42GFzppy8bKpNqpnEHG2aMQ7ri00yTl_087f54dc3d16141afcd2975bb39702faa328bedc0ed14c7a1cdab4feb36b97d3.pdf\",\n        \"thumbnails\":null,\n        \"visible_name\":\"fce17xxxxaxx0x.pdf\",\n        \"name\":\"Q42GFzppy8bKpNqpnEHG2aMQ7ri00yTl_087f54dc3d16141afcd2975bb39702faa328bedc0ed14c7a1cdab4feb36b97d3.pdf\",\n        \"size\":131902,\n        \"mime_type\":\"application/pdf\",\n        \"is_image\":false,\n        \"image_width\":null,\n        \"image_height\":null,\n        \"uploaded_at\":\"2025-06-22T08:00:56.931616+00:00\"\n      }\n    ],\n    \"Part of a set\":[],\n    \"State\":{\n      \"id\":3002,\n      \"value\":\"Production & Used\",\n      \"color\":\"darker-green\"\n    },\n    \"Part Number\":\"40-00011\",\n    \"Revision\":\"A\",\n    \"Notes\":null,\n    \"Sourced By\":null,\n    \"Containing\":[],\n    \"Contained by\":[]\n  },\n  {\n    \"id\":185,\n    \"order\":\"88.00000000000000000000\",\n    \"Full PN\":\"40-00013 Rev.A\",\n    \"External Part Number\":\"17E165715\",\n    \"Manufacturer\":[\n      {\n        \"id\":60,\n        \"value\":\"Amphenol ICC (Commercial Products)\",\n        \"order\":\"28.00000000000000000000\"\n      }\n    ],\n    \"System\":{\n      \"id\":2993,\n      \"value\":\"Controller\",\n      \"color\":\"darker-green\"\n    },\n    \"Item description\":\"CONN BACKSHELL 15POS 180DEG SHLD\",\n    \"Price per unit\":\"6.10\",\n    \"Image\":[\n      {\n        \"url\":\"http://localhost/media/user_files/apUhjblmrmo4aFJq7FruH1jXkEJjGS51_d612191c9e38f9b18ec832beb926e9ad526359ec04104d775632b41682f6b3b4.jpg\",\n        \"thumbnails\":{\n          \"tiny\":{\n            \"url\":\"http://localhost/media/thumbnails/tiny/apUhjblmrmo4aFJq7FruH1jXkEJjGS51_d612191c9e38f9b18ec832beb926e9ad526359ec04104d775632b41682f6b3b4.jpg\",\n            \"width\":null,\n            \"height\":21\n          },\n          \"small\":{\n            \"url\":\"http://localhost/media/thumbnails/small/apUhjblmrmo4aFJq7FruH1jXkEJjGS51_d612191c9e38f9b18ec832beb926e9ad526359ec04104d775632b41682f6b3b4.jpg\",\n            \"width\":48,\n            \"height\":48\n          },\n          \"card_cover\":{\n            \"url\":\"http://localhost/media/thumbnails/card_cover/apUhjblmrmo4aFJq7FruH1jXkEJjGS51_d612191c9e38f9b18ec832beb926e9ad526359ec04104d775632b41682f6b3b4.jpg\",\n            \"width\":300,\n            \"height\":160\n          }\n        },\n        \"visible_name\":\"17E-1657-15.jpg\",\n        \"name\":\"apUhjblmrmo4aFJq7FruH1jXkEJjGS51_d612191c9e38f9b18ec832beb926e9ad526359ec04104d775632b41682f6b3b4.jpg\",\n        \"size\":155258,\n        \"mime_type\":\"image/jpeg\",\n        \"is_image\":true,\n        \"image_width\":640,\n        \"image_height\":640,\n        \"uploaded_at\":\"2025-06-22T07:58:39.522232+00:00\"\n      }\n    ],\n    \"Source\":\"https://www.digikey.co.il/en/products/detail/amphenol-cs-commercial-products/17E165715/1242535\",\n    \"Order Items\":[\n      {\n        \"id\":32,\n        \"value\":\"b71b0a1e-c7c0-45e7-9080-90009f358acd\",\n        \"order\":\"27.00000000000000000000\"\n      }\n    ],\n    \"Datasheet\":[],\n    \"Part of a set\":[\n      {\n        \"id\":186,\n        \"value\":\"40-00012 Rev.A\",\n        \"order\":\"89.00000000000000000000\"\n      }\n    ],\n    \"State\":{\n      \"id\":3002,\n      \"value\":\"Production & Used\",\n      \"color\":\"darker-green\"\n    },\n    \"Part Number\":\"40-00013\",\n    \"Revision\":\"A\",\n    \"Notes\":null,\n    \"Sourced By\":null,\n    \"Containing\":[],\n    \"Contained by\":[]\n  },\n  {\n    \"id\":186,\n    \"order\":\"89.00000000000000000000\",\n    \"Full PN\":\"40-00012 Rev.A\",\n    \"External Part Number\":\"171-015-103L001\",\n    \"Manufacturer\":[\n      {\n        \"id\":61,\n        \"value\":\"NorComp Inc.\",\n        \"order\":\"29.00000000000000000000\"\n      }\n    ],\n    \"System\":{\n      \"id\":2993,\n      \"value\":\"Controller\",\n      \"color\":\"darker-green\"\n    },\n    \"Item description\":\"CONN D-SUB PLUG 15POS PNL MNT\",\n    \"Price per unit\":\"1.41\",\n    \"Image\":[\n      {\n        \"url\":\"http://localhost/media/user_files/pxwBzfwwoyEPnCKwn3ZhCKbacRR4h3n6_05d3cd83cb9e6df11ee08b32ac3e5d77fcb7d0dcb05690ac56f0229301ec72d7.jpg\",\n        \"thumbnails\":{\n          \"tiny\":{\n            \"url\":\"http://localhost/media/thumbnails/tiny/pxwBzfwwoyEPnCKwn3ZhCKbacRR4h3n6_05d3cd83cb9e6df11ee08b32ac3e5d77fcb7d0dcb05690ac56f0229301ec72d7.jpg\",\n            \"width\":null,\n            \"height\":21\n          },\n          \"small\":{\n            \"url\":\"http://localhost/media/thumbnails/small/pxwBzfwwoyEPnCKwn3ZhCKbacRR4h3n6_05d3cd83cb9e6df11ee08b32ac3e5d77fcb7d0dcb05690ac56f0229301ec72d7.jpg\",\n            \"width\":48,\n            \"height\":48\n          },\n          \"card_cover\":{\n            \"url\":\"http://localhost/media/thumbnails/card_cover/pxwBzfwwoyEPnCKwn3ZhCKbacRR4h3n6_05d3cd83cb9e6df11ee08b32ac3e5d77fcb7d0dcb05690ac56f0229301ec72d7.jpg\",\n            \"width\":300,\n            \"height\":160\n          }\n        },\n        \"visible_name\":\"171-015-103L001 .jpg\",\n        \"name\":\"pxwBzfwwoyEPnCKwn3ZhCKbacRR4h3n6_05d3cd83cb9e6df11ee08b32ac3e5d77fcb7d0dcb05690ac56f0229301ec72d7.jpg\",\n        \"size\":158943,\n        \"mime_type\":\"image/jpeg\",\n        \"is_image\":true,\n        \"image_width\":640,\n        \"image_height\":640,\n        \"uploaded_at\":\"2025-06-22T07:59:20.506353+00:00\"\n      }\n    ],\n    \"Source\":\"https://www.digikey.co.il/en/products/detail/norcomp-inc/171-015-103L001/858117\",\n    \"Order Items\":[],\n    \"Datasheet\":[\n      {\n        \"url\":\"http://localhost/media/user_files/gP0AkiExM5uI07fsppZYE5XO3OiFrz77_c3d442b76ac402258ef5df6afb9e9bb28e10cb839bc512da4d73cc6783515e3c.pdf\",\n        \"thumbnails\":null,\n        \"visible_name\":\"171-YYY-10YLYY1.pdf\",\n        \"name\":\"gP0AkiExM5uI07fsppZYE5XO3OiFrz77_c3d442b76ac402258ef5df6afb9e9bb28e10cb839bc512da4d73cc6783515e3c.pdf\",\n        \"size\":91180,\n        \"mime_type\":\"application/pdf\",\n        \"is_image\":false,\n        \"image_width\":null,\n        \"image_height\":null,\n        \"uploaded_at\":\"2025-06-22T08:10:13.654650+00:00\"\n      }\n    ],\n    \"Part of a set\":[\n      {\n        \"id\":185,\n        \"value\":\"40-00013 Rev.A\",\n        \"order\":\"88.00000000000000000000\"\n      }\n    ],\n    \"State\":{\n      \"id\":3004,\n      \"value\":\"Not Used\",\n      \"color\":\"darker-red\"\n    },\n    \"Part Number\":\"40-00012\",\n    \"Revision\":\"A\",\n    \"Notes\":null,\n    \"Sourced By\":null,\n    \"Containing\":[],\n    \"Contained by\":[]\n  },\n  {\n    \"id\":187,\n    \"order\":\"90.00000000000000000000\",\n    \"Full PN\":\"40-00014 Rev.A\",\n    \"External Part Number\":\"CFM-8015V-230-347\",\n    \"Manufacturer\":[\n      {\n        \"id\":62,\n        \"value\":\"Same Sky\",\n        \"order\":\"30.00000000000000000000\"\n      }\n    ],\n    \"System\":{\n      \"id\":2994,\n      \"value\":\"Generic\",\n      \"color\":\"dark-gray\"\n    },\n    \"Item description\":\"Cooling Fan 24v 80mm\",\n    \"Price per unit\":\"8.50\",\n    \"Image\":[\n      {\n        \"url\":\"http://localhost/media/user_files/03mkTbJQv3mtHcwAzExRKsVLw8ApSuGw_ce28a2ec36504c3158614a3fb9c00ce78e0a6b6626379f2021117a226b9864b4.jpg\",\n        \"thumbnails\":{\n          \"tiny\":{\n            \"url\":\"http://localhost/media/thumbnails/tiny/03mkTbJQv3mtHcwAzExRKsVLw8ApSuGw_ce28a2ec36504c3158614a3fb9c00ce78e0a6b6626379f2021117a226b9864b4.jpg\",\n            \"width\":null,\n            \"height\":21\n          },\n          \"small\":{\n            \"url\":\"http://localhost/media/thumbnails/small/03mkTbJQv3mtHcwAzExRKsVLw8ApSuGw_ce28a2ec36504c3158614a3fb9c00ce78e0a6b6626379f2021117a226b9864b4.jpg\",\n            \"width\":48,\n            \"height\":48\n          },\n          \"card_cover\":{\n            \"url\":\"http://localhost/media/thumbnails/card_cover/03mkTbJQv3mtHcwAzExRKsVLw8ApSuGw_ce28a2ec36504c3158614a3fb9c00ce78e0a6b6626379f2021117a226b9864b4.jpg\",\n            \"width\":300,\n            \"height\":160\n          }\n        },\n        \"visible_name\":\"cfm-8015v-124-308_SPL[1].jpg\",\n        \"name\":\"03mkTbJQv3mtHcwAzExRKsVLw8ApSuGw_ce28a2ec36504c3158614a3fb9c00ce78e0a6b6626379f2021117a226b9864b4.jpg\",\n        \"size\":5922,\n        \"mime_type\":\"image/jpeg\",\n        \"is_image\":true,\n        \"image_width\":150,\n        \"image_height\":150,\n        \"uploaded_at\":\"2025-07-09T09:27:07.962093+00:00\"\n      }\n    ],\n    \"Source\":\"https://www.mouser.co.il/ProductDetail/Same-Sky/CFM-8015V-230-347?qs=YCa%2FAAYMW00nDPxH0jNKkQ%3D%3D\",\n    \"Order Items\":[],\n    \"Datasheet\":[\n      {\n        \"url\":\"http://localhost/media/user_files/LM3h3JuJkGlkdtYqtVOMFzdAyYPYixTW_5649d0c7160e42efe8ab72db82d618d92b3a4510a0bece0811ac771f9a7a3d54.pdf\",\n        \"thumbnails\":null,\n        \"visible_name\":\"cfm_80v-3507196[1].pdf\",\n        \"name\":\"LM3h3JuJkGlkdtYqtVOMFzdAyYPYixTW_5649d0c7160e42efe8ab72db82d618d92b3a4510a0bece0811ac771f9a7a3d54.pdf\",\n        \"size\":1040405,\n        \"mime_type\":\"application/pdf\",\n        \"is_image\":false,\n        \"image_width\":null,\n        \"image_height\":null,\n        \"uploaded_at\":\"2025-07-09T09:27:40.845309+00:00\"\n      }\n    ],\n    \"Part of a set\":[\n      {\n        \"id\":188,\n        \"value\":\"20-00022 Rev.A\",\n        \"order\":\"91.00000000000000000000\"\n      }\n    ],\n    \"State\":{\n      \"id\":3003,\n      \"value\":\"EOL\",\n      \"color\":\"darker-red\"\n    },\n    \"Part Number\":\"40-00014\",\n    \"Revision\":\"A\",\n    \"Notes\":null,\n    \"Sourced By\":{\n      \"id\":2998,\n      \"value\":\"ERA\",\n      \"color\":\"darker-gray\"\n    },\n    \"Containing\":[],\n    \"Contained by\":[]\n  },\n  {\n    \"id\":188,\n    \"order\":\"91.00000000000000000000\",\n    \"Full PN\":\"20-00022 Rev.A\",\n    \"External Part Number\":\"08132\",\n    \"Manufacturer\":[\n      {\n        \"id\":58,\n        \"value\":\"Qualtek\",\n        \"order\":\"26.00000000000000000000\"\n      }\n    ],\n    \"System\":{\n      \"id\":2994,\n      \"value\":\"Generic\",\n      \"color\":\"dark-gray\"\n    },\n    \"Item description\":\"Fan Guard\",\n    \"Price per unit\":\"0.63\",\n    \"Image\":[\n      {\n        \"url\":\"http://localhost/media/user_files/LXe66q2LhA3ZLinwVfI0PW6SDEfB4NHK_0fb494fbd7b2f60a3b8a9cfe55384f78b2f6818bfd102b397e6c932daee91b12.jpg\",\n        \"thumbnails\":{\n          \"tiny\":{\n            \"url\":\"http://localhost/media/thumbnails/tiny/LXe66q2LhA3ZLinwVfI0PW6SDEfB4NHK_0fb494fbd7b2f60a3b8a9cfe55384f78b2f6818bfd102b397e6c932daee91b12.jpg\",\n            \"width\":null,\n            \"height\":21\n          },\n          \"small\":{\n            \"url\":\"http://localhost/media/thumbnails/small/LXe66q2LhA3ZLinwVfI0PW6SDEfB4NHK_0fb494fbd7b2f60a3b8a9cfe55384f78b2f6818bfd102b397e6c932daee91b12.jpg\",\n            \"width\":48,\n            \"height\":48\n          },\n          \"card_cover\":{\n            \"url\":\"http://localhost/media/thumbnails/card_cover/LXe66q2LhA3ZLinwVfI0PW6SDEfB4NHK_0fb494fbd7b2f60a3b8a9cfe55384f78b2f6818bfd102b397e6c932daee91b12.jpg\",\n            \"width\":300,\n            \"height\":160\n          }\n        },\n        \"visible_name\":\"08132[1].jpg\",\n        \"name\":\"LXe66q2LhA3ZLinwVfI0PW6SDEfB4NHK_0fb494fbd7b2f60a3b8a9cfe55384f78b2f6818bfd102b397e6c932daee91b12.jpg\",\n        \"size\":4981,\n        \"mime_type\":\"image/jpeg\",\n        \"is_image\":true,\n        \"image_width\":150,\n        \"image_height\":150,\n        \"uploaded_at\":\"2025-07-09T14:50:51.038820+00:00\"\n      }\n    ],\n    \"Source\":\"https://www.mouser.co.il/ProductDetail/Qualtek/08132?qs=258DH3jk4Ve3rqLLi7LhYQ%3D%3D\",\n    \"Order Items\":[],\n    \"Datasheet\":[\n      {\n        \"url\":\"http://localhost/media/user_files/VQMg3c6DFPskdPcZM64KpK8e8BUL7K7l_c98e7a28a529478b0d40bd698c689db78eda99a7af6399d3d3c6ae376c8703b1.pdf\",\n        \"thumbnails\":null,\n        \"visible_name\":\"08132-40010[1].pdf\",\n        \"name\":\"VQMg3c6DFPskdPcZM64KpK8e8BUL7K7l_c98e7a28a529478b0d40bd698c689db78eda99a7af6399d3d3c6ae376c8703b1.pdf\",\n        \"size\":168183,\n        \"mime_type\":\"application/pdf\",\n        \"is_image\":false,\n        \"image_width\":null,\n        \"image_height\":null,\n        \"uploaded_at\":\"2025-07-09T14:51:12.671410+00:00\"\n      }\n    ],\n    \"Part of a set\":[\n      {\n        \"id\":187,\n        \"value\":\"40-00014 Rev.A\",\n        \"order\":\"90.00000000000000000000\"\n      }\n    ],\n    \"State\":{\n      \"id\":3001,\n      \"value\":\"Unknown\",\n      \"color\":\"dark-orange\"\n    },\n    \"Part Number\":\"20-00022\",\n    \"Revision\":\"A\",\n    \"Notes\":null,\n    \"Sourced By\":null,\n    \"Containing\":[],\n    \"Contained by\":[]\n  },\n  {\n    \"id\":189,\n    \"order\":\"92.00000000000000000000\",\n    \"Full PN\":\"20-00000 Rev.A\",\n    \"External Part Number\":\"TBD\",\n    \"Manufacturer\":[],\n    \"System\":{\n      \"id\":2995,\n      \"value\":\"Handle\",\n      \"color\":\"light-brown\"\n    },\n    \"Item description\":\"M3 Barbed Fitting\",\n    \"Price per unit\":null,\n    \"Image\":[\n      {\n        \"url\":\"http://localhost/media/user_files/7vJqMHiZ195rmkTtQ0JOHcAikLs4AKAq_568c0d738c4092d301b5e09774981f784002207f83bbb2810880a5e2dbcff71a.png\",\n        \"thumbnails\":{\n          \"tiny\":{\n            \"url\":\"http://localhost/media/thumbnails/tiny/7vJqMHiZ195rmkTtQ0JOHcAikLs4AKAq_568c0d738c4092d301b5e09774981f784002207f83bbb2810880a5e2dbcff71a.png\",\n            \"width\":null,\n            \"height\":21\n          },\n          \"small\":{\n            \"url\":\"http://localhost/media/thumbnails/small/7vJqMHiZ195rmkTtQ0JOHcAikLs4AKAq_568c0d738c4092d301b5e09774981f784002207f83bbb2810880a5e2dbcff71a.png\",\n            \"width\":48,\n            \"height\":48\n          },\n          \"card_cover\":{\n            \"url\":\"http://localhost/media/thumbnails/card_cover/7vJqMHiZ195rmkTtQ0JOHcAikLs4AKAq_568c0d738c4092d301b5e09774981f784002207f83bbb2810880a5e2dbcff71a.png\",\n            \"width\":300,\n            \"height\":160\n          }\n        },\n        \"visible_name\":\"image.png\",\n        \"name\":\"7vJqMHiZ195rmkTtQ0JOHcAikLs4AKAq_568c0d738c4092d301b5e09774981f784002207f83bbb2810880a5e2dbcff71a.png\",\n        \"size\":491415,\n        \"mime_type\":\"image/png\",\n        \"is_image\":true,\n        \"image_width\":400,\n        \"image_height\":710,\n        \"uploaded_at\":\"2025-08-31T08:52:22.530128+00:00\"\n      },\n      {\n        \"url\":\"http://localhost/media/user_files/ZiZcUT4pq6WdkUZ8JK4yRdbLnPgYYzJ8_969b6454c3a3418f9889c73b4e0e99254171a08f1e33f619782f1571c21dba69.png\",\n        \"thumbnails\":{\n          \"tiny\":{\n            \"url\":\"http://localhost/media/thumbnails/tiny/ZiZcUT4pq6WdkUZ8JK4yRdbLnPgYYzJ8_969b6454c3a3418f9889c73b4e0e99254171a08f1e33f619782f1571c21dba69.png\",\n            \"width\":null,\n            \"height\":21\n          },\n          \"small\":{\n            \"url\":\"http://localhost/media/thumbnails/small/ZiZcUT4pq6WdkUZ8JK4yRdbLnPgYYzJ8_969b6454c3a3418f9889c73b4e0e99254171a08f1e33f619782f1571c21dba69.png\",\n            \"width\":48,\n            \"height\":48\n          },\n          \"card_cover\":{\n            \"url\":\"http://localhost/media/thumbnails/card_cover/ZiZcUT4pq6WdkUZ8JK4yRdbLnPgYYzJ8_969b6454c3a3418f9889c73b4e0e99254171a08f1e33f619782f1571c21dba69.png\",\n            \"width\":300,\n            \"height\":160\n          }\n        },\n        \"visible_name\":\"image.png\",\n        \"name\":\"ZiZcUT4pq6WdkUZ8JK4yRdbLnPgYYzJ8_969b6454c3a3418f9889c73b4e0e99254171a08f1e33f619782f1571c21dba69.png\",\n        \"size\":495118,\n        \"mime_type\":\"image/png\",\n        \"is_image\":true,\n        \"image_width\":400,\n        \"image_height\":710,\n        \"uploaded_at\":\"2025-08-31T08:52:35.614150+00:00\"\n      }\n    ],\n    \"Source\":\"\",\n    \"Order Items\":[],\n    \"Datasheet\":[],\n    \"Part of a set\":[],\n    \"State\":{\n      \"id\":3001,\n      \"value\":\"Unknown\",\n      \"color\":\"dark-orange\"\n    },\n    \"Part Number\":\"20-00000\",\n    \"Revision\":\"A\",\n    \"Notes\":null,\n    \"Sourced By\":null,\n    \"Containing\":[],\n    \"Contained by\":[]\n  },\n  {\n    \"id\":190,\n    \"order\":\"93.00000000000000000000\",\n    \"Full PN\":\"20-00001 Rev.A\",\n    \"External Part Number\":\"TBD\",\n    \"Manufacturer\":[],\n    \"System\":{\n      \"id\":2994,\n      \"value\":\"Generic\",\n      \"color\":\"dark-gray\"\n    },\n    \"Item description\":\"M3x6 Cone Screw\",\n    \"Price per unit\":null,\n    \"Image\":[\n      {\n        \"url\":\"http://localhost/media/user_files/HlpU9Zr2mPtNQCDZCgLROC8TVgl1S7TE_16316c313725d49553bcdb8d7929c2c681568fbe97bd92d442c8f8041616e493.png\",\n        \"thumbnails\":{\n          \"tiny\":{\n            \"url\":\"http://localhost/media/thumbnails/tiny/HlpU9Zr2mPtNQCDZCgLROC8TVgl1S7TE_16316c313725d49553bcdb8d7929c2c681568fbe97bd92d442c8f8041616e493.png\",\n            \"width\":null,\n            \"height\":21\n          },\n          \"small\":{\n            \"url\":\"http://localhost/media/thumbnails/small/HlpU9Zr2mPtNQCDZCgLROC8TVgl1S7TE_16316c313725d49553bcdb8d7929c2c681568fbe97bd92d442c8f8041616e493.png\",\n            \"width\":48,\n            \"height\":48\n          },\n          \"card_cover\":{\n            \"url\":\"http://localhost/media/thumbnails/card_cover/HlpU9Zr2mPtNQCDZCgLROC8TVgl1S7TE_16316c313725d49553bcdb8d7929c2c681568fbe97bd92d442c8f8041616e493.png\",\n            \"width\":300,\n            \"height\":160\n          }\n        },\n        \"visible_name\":\"image.png\",\n        \"name\":\"HlpU9Zr2mPtNQCDZCgLROC8TVgl1S7TE_16316c313725d49553bcdb8d7929c2c681568fbe97bd92d442c8f8041616e493.png\",\n        \"size\":521268,\n        \"mime_type\":\"image/png\",\n        \"is_image\":true,\n        \"image_width\":400,\n        \"image_height\":710,\n        \"uploaded_at\":\"2025-08-31T08:55:35.777101+00:00\"\n      }\n    ],\n    \"Source\":\"\",\n    \"Order Items\":[],\n    \"Datasheet\":[],\n    \"Part of a set\":[],\n    \"State\":{\n      \"id\":3001,\n      \"value\":\"Unknown\",\n      \"color\":\"dark-orange\"\n    },\n    \"Part Number\":\"20-00001\",\n    \"Revision\":\"A\",\n    \"Notes\":null,\n    \"Sourced By\":null,\n    \"Containing\":[],\n    \"Contained by\":[]\n  },\n  {\n    \"id\":191,\n    \"order\":\"94.00000000000000000000\",\n    \"Full PN\":\"20-00002 Rev.A\",\n    \"External Part Number\":\"TBD\",\n    \"Manufacturer\":[],\n    \"System\":null,\n    \"Item description\":\"M2x8\",\n    \"Price per unit\":null,\n    \"Image\":[],\n    \"Source\":\"\",\n    \"Order Items\":[],\n    \"Datasheet\":[],\n    \"Part of a set\":[],\n    \"State\":{\n      \"id\":3001,\n      \"value\":\"Unknown\",\n      \"color\":\"dark-orange\"\n    },\n    \"Part Number\":\"20-00002\",\n    \"Revision\":\"A\",\n    \"Notes\":null,\n    \"Sourced By\":null,\n    \"Containing\":[],\n    \"Contained by\":[]\n  },\n  {\n    \"id\":192,\n    \"order\":\"95.00000000000000000000\",\n    \"Full PN\":\"20-00003 Rev.A\",\n    \"External Part Number\":\"TBD\",\n    \"Manufacturer\":[],\n    \"System\":null,\n    \"Item description\":\"M3x8 Hex Head Cap Screw\",\n    \"Price per unit\":null,\n    \"Image\":[],\n    \"Source\":\"\",\n    \"Order Items\":[],\n    \"Datasheet\":[],\n    \"Part of a set\":[],\n    \"State\":{\n      \"id\":3001,\n      \"value\":\"Unknown\",\n      \"color\":\"dark-orange\"\n    },\n    \"Part Number\":\"20-00003\",\n    \"Revision\":\"A\",\n    \"Notes\":null,\n    \"Sourced By\":null,\n    \"Containing\":[],\n    \"Contained by\":[]\n  },\n  {\n    \"id\":193,\n    \"order\":\"96.00000000000000000000\",\n    \"Full PN\":\"20-00004 Rev.A\",\n    \"External Part Number\":\"TBD\",\n    \"Manufacturer\":[],\n    \"System\":null,\n    \"Item description\":\"M3x6 Small Button Head Hex Cap Screw\",\n    \"Price per unit\":null,\n    \"Image\":[],\n    \"Source\":\"\",\n    \"Order Items\":[],\n    \"Datasheet\":[],\n    \"Part of a set\":[],\n    \"State\":{\n      \"id\":3001,\n      \"value\":\"Unknown\",\n      \"color\":\"dark-orange\"\n    },\n    \"Part Number\":\"20-00004\",\n    \"Revision\":\"A\",\n    \"Notes\":null,\n    \"Sourced By\":null,\n    \"Containing\":[],\n    \"Contained by\":[]\n  },\n  {\n    \"id\":204,\n    \"order\":\"107.00000000000000000000\",\n    \"Full PN\":\"30-00000 Rev.A\",\n    \"External Part Number\":\"N/A\",\n    \"Manufacturer\":[\n      {\n        \"id\":63,\n        \"value\":\"ERA\",\n        \"order\":\"31.00000000000000000000\"\n      }\n    ],\n    \"System\":null,\n    \"Item description\":\"Nova Complete Handle & Umbilical Cord Assembly\",\n    \"Price per unit\":null,\n    \"Image\":[],\n    \"Source\":\"\",\n    \"Order Items\":[],\n    \"Datasheet\":[],\n    \"Part of a set\":[],\n    \"State\":{\n      \"id\":3001,\n      \"value\":\"Unknown\",\n      \"color\":\"dark-orange\"\n    },\n    \"Part Number\":\"30-00000\",\n    \"Revision\":\"A\",\n    \"Notes\":null,\n    \"Sourced By\":null,\n    \"Containing\":[],\n    \"Contained by\":[]\n  },\n  {\n    \"id\":205,\n    \"order\":\"108.00000000000000000000\",\n    \"Full PN\":\"30-00001 Rev.A\",\n    \"External Part Number\":\"N/A\",\n    \"Manufacturer\":[],\n    \"System\":null,\n    \"Item description\":\"Nova Handle Bottom Plastic Enclosure\",\n    \"Price per unit\":null,\n    \"Image\":[],\n    \"Source\":\"\",\n    \"Order Items\":[],\n    \"Datasheet\":[],\n    \"Part of a set\":[],\n    \"State\":{\n      \"id\":3001,\n      \"value\":\"Unknown\",\n      \"color\":\"dark-orange\"\n    },\n    \"Part Number\":\"30-00001\",\n    \"Revision\":\"A\",\n    \"Notes\":null,\n    \"Sourced By\":null,\n    \"Containing\":[],\n    \"Contained by\":[]\n  },\n  {\n    \"id\":206,\n    \"order\":\"109.00000000000000000000\",\n    \"Full PN\":\"30-00002 Rev.A\",\n    \"External Part Number\":\"N/A\",\n    \"Manufacturer\":[],\n    \"System\":null,\n    \"Item description\":\"Nova Handle Strain Relief\",\n    \"Price per unit\":null,\n    \"Image\":[],\n    \"Source\":\"\",\n    \"Order Items\":[],\n    \"Datasheet\":[],\n    \"Part of a set\":[],\n    \"State\":{\n      \"id\":3001,\n      \"value\":\"Unknown\",\n      \"color\":\"dark-orange\"\n    },\n    \"Part Number\":\"30-00002\",\n    \"Revision\":\"A\",\n    \"Notes\":null,\n    \"Sourced By\":null,\n    \"Containing\":[],\n    \"Contained by\":[]\n  },\n  {\n    \"id\":207,\n    \"order\":\"110.00000000000000000000\",\n    \"Full PN\":\"30-00003 Rev.A\",\n    \"External Part Number\":\"N/A\",\n    \"Manufacturer\":[],\n    \"System\":null,\n    \"Item description\":\"Nova Handle Right Orange Plastic Enclosure\",\n    \"Price per unit\":null,\n    \"Image\":[],\n    \"Source\":\"\",\n    \"Order Items\":[],\n    \"Datasheet\":[],\n    \"Part of a set\":[],\n    \"State\":{\n      \"id\":3001,\n      \"value\":\"Unknown\",\n      \"color\":\"dark-orange\"\n    },\n    \"Part Number\":\"30-00003\",\n    \"Revision\":\"A\",\n    \"Notes\":null,\n    \"Sourced By\":null,\n    \"Containing\":[],\n    \"Contained by\":[]\n  },\n  {\n    \"id\":208,\n    \"order\":\"111.00000000000000000000\",\n    \"Full PN\":\"30-00004 Rev.A\",\n    \"External Part Number\":\"N/A\",\n    \"Manufacturer\":[],\n    \"System\":null,\n    \"Item description\":\"Nova Handle Left Orange Plastic Enclosure\",\n    \"Price per unit\":null,\n    \"Image\":[],\n    \"Source\":\"\",\n    \"Order Items\":[],\n    \"Datasheet\":[],\n    \"Part of a set\":[],\n    \"State\":{\n      \"id\":3001,\n      \"value\":\"Unknown\",\n      \"color\":\"dark-orange\"\n    },\n    \"Part Number\":\"30-00004\",\n    \"Revision\":\"A\",\n    \"Notes\":null,\n    \"Sourced By\":null,\n    \"Containing\":[],\n    \"Contained by\":[]\n  },\n  {\n    \"id\":209,\n    \"order\":\"112.00000000000000000000\",\n    \"Full PN\":\"30-00005 Rev.A\",\n    \"External Part Number\":\"N/A\",\n    \"Manufacturer\":[],\n    \"System\":null,\n    \"Item description\":\"Nova Handle Top Plastic Enclosure\",\n    \"Price per unit\":null,\n    \"Image\":[],\n    \"Source\":\"\",\n    \"Order Items\":[],\n    \"Datasheet\":[],\n    \"Part of a set\":[],\n    \"State\":{\n      \"id\":3001,\n      \"value\":\"Unknown\",\n      \"color\":\"dark-orange\"\n    },\n    \"Part Number\":\"30-00005\",\n    \"Revision\":\"A\",\n    \"Notes\":null,\n    \"Sourced By\":null,\n    \"Containing\":[],\n    \"Contained by\":[]\n  },\n  {\n    \"id\":210,\n    \"order\":\"113.00000000000000000000\",\n    \"Full PN\":\"50-00003 Rev.A\",\n    \"External Part Number\":\"N/A\",\n    \"Manufacturer\":[\n      {\n        \"id\":63,\n        \"value\":\"ERA\",\n        \"order\":\"31.00000000000000000000\"\n      }\n    ],\n    \"System\":{\n      \"id\":2996,\n      \"value\":\"Umbilical Cord\",\n      \"color\":\"yellow\"\n    },\n    \"Item description\":\"Umbilical Cord Assembly\",\n    \"Price per unit\":null,\n    \"Image\":[],\n    \"Source\":\"\",\n    \"Order Items\":[],\n    \"Datasheet\":[],\n    \"Part of a set\":[],\n    \"State\":{\n      \"id\":3001,\n      \"value\":\"Unknown\",\n      \"color\":\"dark-orange\"\n    },\n    \"Part Number\":\"50-00003\",\n    \"Revision\":\"A\",\n    \"Notes\":null,\n    \"Sourced By\":null,\n    \"Containing\":[\n      {\n        \"id\":2,\n        \"value\":\"2\",\n        \"order\":\"2.00000000000000000000\"\n      },\n      {\n        \"id\":3,\n        \"value\":\"3\",\n        \"order\":\"3.00000000000000000000\"\n      },\n      {\n        \"id\":4,\n        \"value\":\"4\",\n        \"order\":\"4.00000000000000000000\"\n      },\n      {\n        \"id\":5,\n        \"value\":\"5\",\n        \"order\":\"5.00000000000000000000\"\n      },\n      {\n        \"id\":6,\n        \"value\":\"6\",\n        \"order\":\"6.00000000000000000000\"\n      }\n    ],\n    \"Contained by\":[]\n  },\n  {\n    \"id\":211,\n    \"order\":\"114.00000000000000000000\",\n    \"Full PN\":\"30-00007 Rev.A\",\n    \"External Part Number\":\"N/A\",\n    \"Manufacturer\":[],\n    \"System\":null,\n    \"Item description\":\"Nova Handle Hot Electrode\",\n    \"Price per unit\":null,\n    \"Image\":[],\n    \"Source\":\"\",\n    \"Order Items\":[],\n    \"Datasheet\":[],\n    \"Part of a set\":[],\n    \"State\":{\n      \"id\":3001,\n      \"value\":\"Unknown\",\n      \"color\":\"dark-orange\"\n    },\n    \"Part Number\":\"30-00007\",\n    \"Revision\":\"A\",\n    \"Notes\":null,\n    \"Sourced By\":null,\n    \"Containing\":[],\n    \"Contained by\":[]\n  },\n  {\n    \"id\":212,\n    \"order\":\"115.00000000000000000000\",\n    \"Full PN\":\"30-00009 Rev.A\",\n    \"External Part Number\":\"N/A\",\n    \"Manufacturer\":[],\n    \"System\":null,\n    \"Item description\":\"Nova Handle Electrode Bridge\",\n    \"Price per unit\":null,\n    \"Image\":[],\n    \"Source\":\"\",\n    \"Order Items\":[],\n    \"Datasheet\":[],\n    \"Part of a set\":[],\n    \"State\":{\n      \"id\":3001,\n      \"value\":\"Unknown\",\n      \"color\":\"dark-orange\"\n    },\n    \"Part Number\":\"30-00009\",\n    \"Revision\":\"A\",\n    \"Notes\":null,\n    \"Sourced By\":null,\n    \"Containing\":[],\n    \"Contained by\":[]\n  },\n  {\n    \"id\":213,\n    \"order\":\"116.00000000000000000000\",\n    \"Full PN\":\"30-00010 Rev.A\",\n    \"External Part Number\":\"N/A\",\n    \"Manufacturer\":[],\n    \"System\":null,\n    \"Item description\":\"Nova Handle Coax Cable Retention Bracket\",\n    \"Price per unit\":null,\n    \"Image\":[],\n    \"Source\":\"\",\n    \"Order Items\":[],\n    \"Datasheet\":[],\n    \"Part of a set\":[],\n    \"State\":{\n      \"id\":3001,\n      \"value\":\"Unknown\",\n      \"color\":\"dark-orange\"\n    },\n    \"Part Number\":\"30-00010\",\n    \"Revision\":\"A\",\n    \"Notes\":null,\n    \"Sourced By\":null,\n    \"Containing\":[],\n    \"Contained by\":[]\n  },\n  {\n    \"id\":214,\n    \"order\":\"117.00000000000000000000\",\n    \"Full PN\":\"30-00011 Rev.A\",\n    \"External Part Number\":\"N/A\",\n    \"Manufacturer\":[],\n    \"System\":null,\n    \"Item description\":\"Nova Handle Final Retention Bracket\",\n    \"Price per unit\":null,\n    \"Image\":[],\n    \"Source\":\"\",\n    \"Order Items\":[],\n    \"Datasheet\":[],\n    \"Part of a set\":[],\n    \"State\":{\n      \"id\":3001,\n      \"value\":\"Unknown\",\n      \"color\":\"dark-orange\"\n    },\n    \"Part Number\":\"30-00011\",\n    \"Revision\":\"A\",\n    \"Notes\":null,\n    \"Sourced By\":null,\n    \"Containing\":[],\n    \"Contained by\":[]\n  },\n  {\n    \"id\":215,\n    \"order\":\"118.00000000000000000000\",\n    \"Full PN\":\"30-00012 Rev.A\",\n    \"External Part Number\":\"N/A\",\n    \"Manufacturer\":[],\n    \"System\":null,\n    \"Item description\":\"Nova Handle LED PCBA Offsetting Mount\",\n    \"Price per unit\":null,\n    \"Image\":[],\n    \"Source\":\"\",\n    \"Order Items\":[],\n    \"Datasheet\":[],\n    \"Part of a set\":[],\n    \"State\":{\n      \"id\":3001,\n      \"value\":\"Unknown\",\n      \"color\":\"dark-orange\"\n    },\n    \"Part Number\":\"30-00012\",\n    \"Revision\":\"A\",\n    \"Notes\":null,\n    \"Sourced By\":null,\n    \"Containing\":[],\n    \"Contained by\":[]\n  },\n  {\n    \"id\":216,\n    \"order\":\"119.00000000000000000000\",\n    \"Full PN\":\"30-00013 Rev.A\",\n    \"External Part Number\":\"N/A\",\n    \"Manufacturer\":[],\n    \"System\":null,\n    \"Item description\":\"Nova Handle LED PCBA Large Standoff\",\n    \"Price per unit\":null,\n    \"Image\":[],\n    \"Source\":\"\",\n    \"Order Items\":[],\n    \"Datasheet\":[],\n    \"Part of a set\":[],\n    \"State\":{\n      \"id\":3001,\n      \"value\":\"Unknown\",\n      \"color\":\"dark-orange\"\n    },\n    \"Part Number\":\"30-00013\",\n    \"Revision\":\"A\",\n    \"Notes\":null,\n    \"Sourced By\":null,\n    \"Containing\":[],\n    \"Contained by\":[]\n  },\n  {\n    \"id\":217,\n    \"order\":\"120.00000000000000000000\",\n    \"Full PN\":\"30-00014 Rev.A\",\n    \"External Part Number\":\"N/A\",\n    \"Manufacturer\":[],\n    \"System\":null,\n    \"Item description\":\"Nova Handle LED PCBA Small Standoff\",\n    \"Price per unit\":null,\n    \"Image\":[],\n    \"Source\":\"\",\n    \"Order Items\":[],\n    \"Datasheet\":[],\n    \"Part of a set\":[],\n    \"State\":{\n      \"id\":3001,\n      \"value\":\"Unknown\",\n      \"color\":\"dark-orange\"\n    },\n    \"Part Number\":\"30-00014\",\n    \"Revision\":\"A\",\n    \"Notes\":null,\n    \"Sourced By\":null,\n    \"Containing\":[],\n    \"Contained by\":[]\n  },\n  {\n    \"id\":218,\n    \"order\":\"121.00000000000000000000\",\n    \"Full PN\":\"50-00000 Rev.A\",\n    \"External Part Number\":\"N/A\",\n    \"Manufacturer\":[],\n    \"System\":{\n      \"id\":2995,\n      \"value\":\"Handle\",\n      \"color\":\"light-brown\"\n    },\n    \"Item description\":\"Nova Handle LED PCBA Right\",\n    \"Price per unit\":null,\n    \"Image\":[],\n    \"Source\":\"\",\n    \"Order Items\":[],\n    \"Datasheet\":[],\n    \"Part of a set\":[\n      {\n        \"id\":218,\n        \"value\":\"50-00000 Rev.A\",\n        \"order\":\"121.00000000000000000000\"\n      },\n      {\n        \"id\":219,\n        \"value\":\"50-00001 Rev.A\",\n        \"order\":\"122.00000000000000000000\"\n      }\n    ],\n    \"State\":{\n      \"id\":3001,\n      \"value\":\"Unknown\",\n      \"color\":\"dark-orange\"\n    },\n    \"Part Number\":\"50-00000\",\n    \"Revision\":\"A\",\n    \"Notes\":null,\n    \"Sourced By\":null,\n    \"Containing\":[],\n    \"Contained by\":[]\n  },\n  {\n    \"id\":219,\n    \"order\":\"122.00000000000000000000\",\n    \"Full PN\":\"50-00001 Rev.A\",\n    \"External Part Number\":\"N/A\",\n    \"Manufacturer\":[],\n    \"System\":{\n      \"id\":2995,\n      \"value\":\"Handle\",\n      \"color\":\"light-brown\"\n    },\n    \"Item description\":\"Nova Handle LED PCBA Left\",\n    \"Price per unit\":null,\n    \"Image\":[],\n    \"Source\":\"\",\n    \"Order Items\":[],\n    \"Datasheet\":[],\n    \"Part of a set\":[\n      {\n        \"id\":218,\n        \"value\":\"50-00000 Rev.A\",\n        \"order\":\"121.00000000000000000000\"\n      },\n      {\n        \"id\":219,\n        \"value\":\"50-00001 Rev.A\",\n        \"order\":\"122.00000000000000000000\"\n      }\n    ],\n    \"State\":{\n      \"id\":3001,\n      \"value\":\"Unknown\",\n      \"color\":\"dark-orange\"\n    },\n    \"Part Number\":\"50-00001\",\n    \"Revision\":\"A\",\n    \"Notes\":null,\n    \"Sourced By\":null,\n    \"Containing\":[],\n    \"Contained by\":[]\n  },\n  {\n    \"id\":221,\n    \"order\":\"124.00000000000000000000\",\n    \"Full PN\":\"40-00073 Rev.A\",\n    \"External Part Number\":\"031-320\",\n    \"Manufacturer\":[\n      {\n        \"id\":64,\n        \"value\":\"Amphenol RF\",\n        \"order\":\"32.00000000000000000000\"\n      }\n    ],\n    \"System\":{\n      \"id\":2996,\n      \"value\":\"Umbilical Cord\",\n      \"color\":\"yellow\"\n    },\n    \"Item description\":\"RF Connector BNC Straight Crimp Plug RG-55 RG-142 RG-223 RG-400 50 Ohm\",\n    \"Price per unit\":\"7.93\",\n    \"Image\":[\n      {\n        \"url\":\"http://localhost/media/user_files/lUgdyZZPuT3xWnnB3bLBpcrLgcWX17Pb_9558af6ebe4955ce9f3e2e251a033f4152eea8363fecebb12b738c12d913836f.png\",\n        \"thumbnails\":{\n          \"tiny\":{\n            \"url\":\"http://localhost/media/thumbnails/tiny/lUgdyZZPuT3xWnnB3bLBpcrLgcWX17Pb_9558af6ebe4955ce9f3e2e251a033f4152eea8363fecebb12b738c12d913836f.png\",\n            \"width\":null,\n            \"height\":21\n          },\n          \"small\":{\n            \"url\":\"http://localhost/media/thumbnails/small/lUgdyZZPuT3xWnnB3bLBpcrLgcWX17Pb_9558af6ebe4955ce9f3e2e251a033f4152eea8363fecebb12b738c12d913836f.png\",\n            \"width\":48,\n            \"height\":48\n          },\n          \"card_cover\":{\n            \"url\":\"http://localhost/media/thumbnails/card_cover/lUgdyZZPuT3xWnnB3bLBpcrLgcWX17Pb_9558af6ebe4955ce9f3e2e251a033f4152eea8363fecebb12b738c12d913836f.png\",\n            \"width\":300,\n            \"height\":160\n          }\n        },\n        \"visible_name\":\"image.png\",\n        \"name\":\"lUgdyZZPuT3xWnnB3bLBpcrLgcWX17Pb_9558af6ebe4955ce9f3e2e251a033f4152eea8363fecebb12b738c12d913836f.png\",\n        \"size\":533238,\n        \"mime_type\":\"image/png\",\n        \"is_image\":true,\n        \"image_width\":1264,\n        \"image_height\":697,\n        \"uploaded_at\":\"2025-09-03T17:31:23.969627+00:00\"\n      }\n    ],\n    \"Source\":\"https://mou.sr/4p3PyXR\",\n    \"Order Items\":[],\n    \"Datasheet\":[\n      {\n        \"url\":\"http://localhost/media/user_files/UxO6oXfw863NZ1eYNSHkBJjoLuqOL4Oa_9aad5955858e5165df5a785c1ebba35244f1d38457383cd8eb216a00b226de9f.pdf\",\n        \"thumbnails\":null,\n        \"visible_name\":\"C31-320.pdf\",\n        \"name\":\"UxO6oXfw863NZ1eYNSHkBJjoLuqOL4Oa_9aad5955858e5165df5a785c1ebba35244f1d38457383cd8eb216a00b226de9f.pdf\",\n        \"size\":136234,\n        \"mime_type\":\"application/pdf\",\n        \"is_image\":false,\n        \"image_width\":null,\n        \"image_height\":null,\n        \"uploaded_at\":\"2025-09-03T17:29:42.168492+00:00\"\n      }\n    ],\n    \"Part of a set\":[],\n    \"State\":{\n      \"id\":3001,\n      \"value\":\"Unknown\",\n      \"color\":\"dark-orange\"\n    },\n    \"Part Number\":\"40-00073\",\n    \"Revision\":\"A\",\n    \"Notes\":\"Harness ordered at Telem\",\n    \"Sourced By\":{\n      \"id\":3000,\n      \"value\":\"TBD\",\n      \"color\":\"darker-orange\"\n    },\n    \"Containing\":[],\n    \"Contained by\":[]\n  },\n  {\n    \"id\":222,\n    \"order\":\"125.00000000000000000000\",\n    \"Full PN\":\"10-00002 Rev.A\",\n    \"External Part Number\":\"RW-175-3/4-X-STK\",\n    \"Manufacturer\":[\n      {\n        \"id\":19,\n        \"value\":\"TE Connectivity\",\n        \"order\":\"19.00000000000000000000\"\n      }\n    ],\n    \"System\":{\n      \"id\":2996,\n      \"value\":\"Umbilical Cord\",\n      \"color\":\"yellow\"\n    },\n    \"Item description\":\"Heat Shrink Tubing & Sleeves HS-TBG 19.1MM 2:1 CL PRICE PER STICK\",\n    \"Price per unit\":\"32.45\",\n    \"Image\":[\n      {\n        \"url\":\"http://localhost/media/user_files/xagdklncG9hyxNKJZP4n1ugAdRKwgWqv_fe7dc83fd19686709f16e7d1773ccc909b9595c6b8d007ca19e28f07920b2f48.png\",\n        \"thumbnails\":{\n          \"tiny\":{\n            \"url\":\"http://localhost/media/thumbnails/tiny/xagdklncG9hyxNKJZP4n1ugAdRKwgWqv_fe7dc83fd19686709f16e7d1773ccc909b9595c6b8d007ca19e28f07920b2f48.png\",\n            \"width\":null,\n            \"height\":21\n          },\n          \"small\":{\n            \"url\":\"http://localhost/media/thumbnails/small/xagdklncG9hyxNKJZP4n1ugAdRKwgWqv_fe7dc83fd19686709f16e7d1773ccc909b9595c6b8d007ca19e28f07920b2f48.png\",\n            \"width\":48,\n            \"height\":48\n          },\n          \"card_cover\":{\n            \"url\":\"http://localhost/media/thumbnails/card_cover/xagdklncG9hyxNKJZP4n1ugAdRKwgWqv_fe7dc83fd19686709f16e7d1773ccc909b9595c6b8d007ca19e28f07920b2f48.png\",\n            \"width\":300,\n            \"height\":160\n          }\n        },\n        \"visible_name\":\"image.png\",\n        \"name\":\"xagdklncG9hyxNKJZP4n1ugAdRKwgWqv_fe7dc83fd19686709f16e7d1773ccc909b9595c6b8d007ca19e28f07920b2f48.png\",\n        \"size\":14166,\n        \"mime_type\":\"image/png\",\n        \"is_image\":true,\n        \"image_width\":300,\n        \"image_height\":225,\n        \"uploaded_at\":\"2025-09-03T17:45:04.692078+00:00\"\n      }\n    ],\n    \"Source\":\"https://mou.sr/4g9C35d\",\n    \"Order Items\":[],\n    \"Datasheet\":[\n      {\n        \"url\":\"http://localhost/media/user_files/TTVPtr0IUYdS17vSm9JCQDD1hCMgmOFg_72b170499620c77c1807ef73a752f9e633f7f80dcce1507facaa59029bb85f38.pdf\",\n        \"thumbnails\":null,\n        \"visible_name\":\"ENG_CD_RW-175_A.pdf\",\n        \"name\":\"TTVPtr0IUYdS17vSm9JCQDD1hCMgmOFg_72b170499620c77c1807ef73a752f9e633f7f80dcce1507facaa59029bb85f38.pdf\",\n        \"size\":100517,\n        \"mime_type\":\"application/pdf\",\n        \"is_image\":false,\n        \"image_width\":null,\n        \"image_height\":null,\n        \"uploaded_at\":\"2025-09-03T17:46:10.564931+00:00\"\n      }\n    ],\n    \"Part of a set\":[],\n    \"State\":{\n      \"id\":3001,\n      \"value\":\"Unknown\",\n      \"color\":\"dark-orange\"\n    },\n    \"Part Number\":\"10-00002\",\n    \"Revision\":\"A\",\n    \"Notes\":\"\",\n    \"Sourced By\":null,\n    \"Containing\":[],\n    \"Contained by\":[]\n  },\n  {\n    \"id\":227,\n    \"order\":\"128.00000000000000000000\",\n    \"Full PN\":\"10-00005 Rev.A\",\n    \"External Part Number\":\"FIT221B1/4 BK100\",\n    \"Manufacturer\":[\n      {\n        \"id\":68,\n        \"value\":\"Alpha Wire\",\n        \"order\":\"36.00000000000000000000\"\n      }\n    ],\n    \"System\":{\n      \"id\":2996,\n      \"value\":\"Umbilical Cord\",\n      \"color\":\"yellow\"\n    },\n    \"Item description\":\"Heat Shrink Tubing & Sleeves 1/4in ID SHRNK TUBN 4ft LTHS BLACK\",\n    \"Price per unit\":\"3.30\",\n    \"Image\":[\n      {\n        \"url\":\"http://localhost/media/user_files/1RkmcpkN9DKJIG2xmGj0QGwMLXhOthXV_37efbdaf29c2da42eee20887a4327f7f3447bd278b68d555b600385babca641b.png\",\n        \"thumbnails\":{\n          \"tiny\":{\n            \"url\":\"http://localhost/media/thumbnails/tiny/1RkmcpkN9DKJIG2xmGj0QGwMLXhOthXV_37efbdaf29c2da42eee20887a4327f7f3447bd278b68d555b600385babca641b.png\",\n            \"width\":null,\n            \"height\":21\n          },\n          \"small\":{\n            \"url\":\"http://localhost/media/thumbnails/small/1RkmcpkN9DKJIG2xmGj0QGwMLXhOthXV_37efbdaf29c2da42eee20887a4327f7f3447bd278b68d555b600385babca641b.png\",\n            \"width\":48,\n            \"height\":48\n          },\n          \"card_cover\":{\n            \"url\":\"http://localhost/media/thumbnails/card_cover/1RkmcpkN9DKJIG2xmGj0QGwMLXhOthXV_37efbdaf29c2da42eee20887a4327f7f3447bd278b68d555b600385babca641b.png\",\n            \"width\":300,\n            \"height\":160\n          }\n        },\n        \"visible_name\":\"image.png\",\n        \"name\":\"1RkmcpkN9DKJIG2xmGj0QGwMLXhOthXV_37efbdaf29c2da42eee20887a4327f7f3447bd278b68d555b600385babca641b.png\",\n        \"size\":962017,\n        \"mime_type\":\"image/png\",\n        \"is_image\":true,\n        \"image_width\":1200,\n        \"image_height\":803,\n        \"uploaded_at\":\"2025-09-03T18:17:04.159592+00:00\"\n      }\n    ],\n    \"Source\":\"https://mou.sr/3I4NFtn\",\n    \"Order Items\":[],\n    \"Datasheet\":[\n      {\n        \"url\":\"http://localhost/media/user_files/5dIGA1YxEQpKY5wl9uzZUDog1oYYfPqo_2de4ef693f2418c4d504964a04ba55d56a4bdecf3bf6c3773c22c8e39b82964f.pdf\",\n        \"thumbnails\":null,\n        \"visible_name\":\"Alpha Wire FIT-221B-1_4 Tech Data.pdf\",\n        \"name\":\"5dIGA1YxEQpKY5wl9uzZUDog1oYYfPqo_2de4ef693f2418c4d504964a04ba55d56a4bdecf3bf6c3773c22c8e39b82964f.pdf\",\n        \"size\":396741,\n        \"mime_type\":\"application/pdf\",\n        \"is_image\":false,\n        \"image_width\":null,\n        \"image_height\":null,\n        \"uploaded_at\":\"2025-09-03T18:17:36.591876+00:00\"\n      }\n    ],\n    \"Part of a set\":[],\n    \"State\":{\n      \"id\":3001,\n      \"value\":\"Unknown\",\n      \"color\":\"dark-orange\"\n    },\n    \"Part Number\":\"10-00005\",\n    \"Revision\":\"A\",\n    \"Notes\":\"\",\n    \"Sourced By\":null,\n    \"Containing\":[],\n    \"Contained by\":[]\n  },\n  {\n    \"id\":229,\n    \"order\":\"130.00000000000000000000\",\n    \"Full PN\":\"50-00002 Rev.A\",\n    \"External Part Number\":\"N/A\",\n    \"Manufacturer\":[],\n    \"System\":{\n      \"id\":2996,\n      \"value\":\"Umbilical Cord\",\n      \"color\":\"yellow\"\n    },\n    \"Item description\":\"Nova Umbilical Feedthrough Harness\",\n    \"Price per unit\":null,\n    \"Image\":[],\n    \"Source\":\"\",\n    \"Order Items\":[],\n    \"Datasheet\":[],\n    \"Part of a set\":[],\n    \"State\":{\n      \"id\":3001,\n      \"value\":\"Unknown\",\n      \"color\":\"dark-orange\"\n    },\n    \"Part Number\":\"50-00002\",\n    \"Revision\":\"A\",\n    \"Notes\":\"\",\n    \"Sourced By\":{\n      \"id\":2998,\n      \"value\":\"ERA\",\n      \"color\":\"darker-gray\"\n    },\n    \"Containing\":[],\n    \"Contained by\":[]\n  },\n  {\n    \"id\":230,\n    \"order\":\"131.00000000000000000000\",\n    \"Full PN\":\"40-00074 Rev.A\",\n    \"External Part Number\":\"39-01-2060\",\n    \"Manufacturer\":[\n      {\n        \"id\":102,\n        \"value\":\"Molex\",\n        \"order\":\"38.00000000000000000000\"\n      }\n    ],\n    \"System\":{\n      \"id\":2999,\n      \"value\":\"Wiring\",\n      \"color\":\"dark-purple\"\n    },\n    \"Item description\":\"Headers & Wire Housings 6 CKT RCPT HOUSING\",\n    \"Price per unit\":\"0.32\",\n    \"Image\":[\n      {\n        \"url\":\"http://localhost/media/user_files/YULRk0i3hBMzEF6nwU3XnuuDc16w7qOC_b455563172d17629b9575a25ff87e4cb86f2b7934687ba8af7cf9a4886b8ad8c.png\",\n        \"thumbnails\":{\n          \"tiny\":{\n            \"url\":\"http://localhost/media/thumbnails/tiny/YULRk0i3hBMzEF6nwU3XnuuDc16w7qOC_b455563172d17629b9575a25ff87e4cb86f2b7934687ba8af7cf9a4886b8ad8c.png\",\n            \"width\":null,\n            \"height\":21\n          },\n          \"small\":{\n            \"url\":\"http://localhost/media/thumbnails/small/YULRk0i3hBMzEF6nwU3XnuuDc16w7qOC_b455563172d17629b9575a25ff87e4cb86f2b7934687ba8af7cf9a4886b8ad8c.png\",\n            \"width\":48,\n            \"height\":48\n          },\n          \"card_cover\":{\n            \"url\":\"http://localhost/media/thumbnails/card_cover/YULRk0i3hBMzEF6nwU3XnuuDc16w7qOC_b455563172d17629b9575a25ff87e4cb86f2b7934687ba8af7cf9a4886b8ad8c.png\",\n            \"width\":300,\n            \"height\":160\n          }\n        },\n        \"visible_name\":\"image.png\",\n        \"name\":\"YULRk0i3hBMzEF6nwU3XnuuDc16w7qOC_b455563172d17629b9575a25ff87e4cb86f2b7934687ba8af7cf9a4886b8ad8c.png\",\n        \"size\":239237,\n        \"mime_type\":\"image/png\",\n        \"is_image\":true,\n        \"image_width\":987,\n        \"image_height\":701,\n        \"uploaded_at\":\"2025-09-04T07:36:06.021848+00:00\"\n      }\n    ],\n    \"Source\":\"https://mou.sr/4njuJpX\",\n    \"Order Items\":[],\n    \"Datasheet\":[\n      {\n        \"url\":\"http://localhost/media/user_files/XSVvqTHvqpN16tAIOop6Nk4BB6Nvfjzp_7e9586b95923b4f9801ecf7f9f37df5ea16e7d2af5c9037accd8c43f632f1117.pdf\",\n        \"thumbnails\":null,\n        \"visible_name\":\"download.pdf\",\n        \"name\":\"XSVvqTHvqpN16tAIOop6Nk4BB6Nvfjzp_7e9586b95923b4f9801ecf7f9f37df5ea16e7d2af5c9037accd8c43f632f1117.pdf\",\n        \"size\":66270,\n        \"mime_type\":\"application/pdf\",\n        \"is_image\":false,\n        \"image_width\":null,\n        \"image_height\":null,\n        \"uploaded_at\":\"2025-09-04T07:36:33.136917+00:00\"\n      }\n    ],\n    \"Part of a set\":[],\n    \"State\":{\n      \"id\":3001,\n      \"value\":\"Unknown\",\n      \"color\":\"dark-orange\"\n    },\n    \"Part Number\":\"40-00074\",\n    \"Revision\":\"A\",\n    \"Notes\":\"\",\n    \"Sourced By\":{\n      \"id\":2997,\n      \"value\":\"Contractor\",\n      \"color\":\"darker-brown\"\n    },\n    \"Containing\":[],\n    \"Contained by\":[]\n  },\n  {\n    \"id\":232,\n    \"order\":\"133.00000000000000000000\",\n    \"Full PN\":\"70-00001 Rev.A\",\n    \"External Part Number\":\"N/A\",\n    \"Manufacturer\":[\n      {\n        \"id\":63,\n        \"value\":\"ERA\",\n        \"order\":\"31.00000000000000000000\"\n      }\n    ],\n    \"System\":{\n      \"id\":2996,\n      \"value\":\"Umbilical Cord\",\n      \"color\":\"yellow\"\n    },\n    \"Item description\":\"Umbilical Cord Label\",\n    \"Price per unit\":null,\n    \"Image\":[],\n    \"Source\":\"\",\n    \"Order Items\":[],\n    \"Datasheet\":[],\n    \"Part of a set\":[],\n    \"State\":{\n      \"id\":3001,\n      \"value\":\"Unknown\",\n      \"color\":\"dark-orange\"\n    },\n    \"Part Number\":\"70-00001\",\n    \"Revision\":\"A\",\n    \"Notes\":\"\",\n    \"Sourced By\":null,\n    \"Containing\":[],\n    \"Contained by\":[]\n  },\n  {\n    \"id\":233,\n    \"order\":\"134.00000000000000000000\",\n    \"Full PN\":\"50-00005 Rev.A\",\n    \"External Part Number\":\"N/A\",\n    \"Manufacturer\":[\n      {\n        \"id\":63,\n        \"value\":\"ERA\",\n        \"order\":\"31.00000000000000000000\"\n      }\n    ],\n    \"System\":{\n      \"id\":2996,\n      \"value\":\"Umbilical Cord\",\n      \"color\":\"yellow\"\n    },\n    \"Item description\":\"Umbilical Cord Coax Cable\",\n    \"Price per unit\":null,\n    \"Image\":[],\n    \"Source\":\"\",\n    \"Order Items\":[],\n    \"Datasheet\":[],\n    \"Part of a set\":[],\n    \"State\":{\n      \"id\":3001,\n      \"value\":\"Unknown\",\n      \"color\":\"dark-orange\"\n    },\n    \"Part Number\":\"50-00005\",\n    \"Revision\":\"A\",\n    \"Notes\":\"\",\n    \"Sourced By\":null,\n    \"Containing\":[\n      {\n        \"id\":7,\n        \"value\":\"7\",\n        \"order\":\"7.00000000000000000000\"\n      }\n    ],\n    \"Contained by\":[]\n  },\n  {\n    \"id\":234,\n    \"order\":\"135.00000000000000000000\",\n    \"Full PN\":\"50-00006 Rev.A\",\n    \"External Part Number\":\"N/A\",\n    \"Manufacturer\":[\n      {\n        \"id\":63,\n        \"value\":\"ERA\",\n        \"order\":\"31.00000000000000000000\"\n      }\n    ],\n    \"System\":{\n      \"id\":2993,\n      \"value\":\"Controller\",\n      \"color\":\"darker-green\"\n    },\n    \"Item description\":\"Controller Unit\",\n    \"Price per unit\":null,\n    \"Image\":[],\n    \"Source\":\"\",\n    \"Order Items\":[],\n    \"Datasheet\":[],\n    \"Part of a set\":[],\n    \"State\":{\n      \"id\":3001,\n      \"value\":\"Unknown\",\n      \"color\":\"dark-orange\"\n    },\n    \"Part Number\":\"50-00006\",\n    \"Revision\":\"A\",\n    \"Notes\":\"Includes a Controller Enclosure Assembly and a Controller Board\",\n    \"Sourced By\":{\n      \"id\":2998,\n      \"value\":\"ERA\",\n      \"color\":\"darker-gray\"\n    },\n    \"Containing\":[],\n    \"Contained by\":[]\n  },\n  {\n    \"id\":235,\n    \"order\":\"136.00000000000000000000\",\n    \"Full PN\":\"80-00000 Rev.A\",\n    \"External Part Number\":\"N/A\",\n    \"Manufacturer\":[\n      {\n        \"id\":63,\n        \"value\":\"ERA\",\n        \"order\":\"31.00000000000000000000\"\n      }\n    ],\n    \"System\":{\n      \"id\":2994,\n      \"value\":\"Generic\",\n      \"color\":\"dark-gray\"\n    },\n    \"Item description\":\"ERA Nova Device\",\n    \"Price per unit\":null,\n    \"Image\":[],\n    \"Source\":\"\",\n    \"Order Items\":[],\n    \"Datasheet\":[],\n    \"Part of a set\":[],\n    \"State\":{\n      \"id\":3001,\n      \"value\":\"Unknown\",\n      \"color\":\"dark-orange\"\n    },\n    \"Part Number\":\"80-00000\",\n    \"Revision\":\"A\",\n    \"Notes\":\"Deliverable\",\n    \"Sourced By\":null,\n    \"Containing\":[],\n    \"Contained by\":[]\n  },\n  {\n    \"id\":237,\n    \"order\":\"137.00000000000000000000\",\n    \"Full PN\":\"40-00075 Rev.A\",\n    \"External Part Number\":\"51110-1056\",\n    \"Manufacturer\":[\n      {\n        \"id\":102,\n        \"value\":\"Molex\",\n        \"order\":\"38.00000000000000000000\"\n      }\n    ],\n    \"System\":{\n      \"id\":2963,\n      \"value\":\"DC Power Supply\",\n      \"color\":\"orange\"\n    },\n    \"Item description\":\"2.00mm Pitch, Milli-Grid Receptacle Housing, 10 Circuits, with Center Locking Ramp and Side Polarization Keys, Lead-Free.\",\n    \"Price per unit\":\"0.18\",\n    \"Image\":[\n      {\n        \"url\":\"http://localhost/media/user_files/ZXIO0Hgfm2is5meC00dFsgrOk0jtdSmy_1160750161a612de44b389059a54cedc4e922dc39be873eede55e37b35fc2fa8.png\",\n        \"thumbnails\":{\n          \"tiny\":{\n            \"url\":\"http://localhost/media/thumbnails/tiny/ZXIO0Hgfm2is5meC00dFsgrOk0jtdSmy_1160750161a612de44b389059a54cedc4e922dc39be873eede55e37b35fc2fa8.png\",\n            \"width\":null,\n            \"height\":21\n          },\n          \"small\":{\n            \"url\":\"http://localhost/media/thumbnails/small/ZXIO0Hgfm2is5meC00dFsgrOk0jtdSmy_1160750161a612de44b389059a54cedc4e922dc39be873eede55e37b35fc2fa8.png\",\n            \"width\":48,\n            \"height\":48\n          },\n          \"card_cover\":{\n            \"url\":\"http://localhost/media/thumbnails/card_cover/ZXIO0Hgfm2is5meC00dFsgrOk0jtdSmy_1160750161a612de44b389059a54cedc4e922dc39be873eede55e37b35fc2fa8.png\",\n            \"width\":300,\n            \"height\":160\n          }\n        },\n        \"visible_name\":\"image.png\",\n        \"name\":\"ZXIO0Hgfm2is5meC00dFsgrOk0jtdSmy_1160750161a612de44b389059a54cedc4e922dc39be873eede55e37b35fc2fa8.png\",\n        \"size\":465822,\n        \"mime_type\":\"image/png\",\n        \"is_image\":true,\n        \"image_width\":996,\n        \"image_height\":748,\n        \"uploaded_at\":\"2025-09-21T07:40:39.751688+00:00\"\n      }\n    ],\n    \"Source\":\"https://www.mouser.co.il/ProductDetail/Molex/51110-1056?qs=39WuQm6e6OmwmDPLAER7sA%3D%3D\",\n    \"Order Items\":[],\n    \"Datasheet\":[\n      {\n        \"url\":\"http://localhost/media/user_files/SW0HFPad77KnKeGy7hv6YGEysbLuJ3Lw_4300ea312f0dd59e98d650f20afa95d072778fc901ba8c973f67a81b6dbcbf93.pdf\",\n        \"thumbnails\":null,\n        \"visible_name\":\"download (1).pdf\",\n        \"name\":\"SW0HFPad77KnKeGy7hv6YGEysbLuJ3Lw_4300ea312f0dd59e98d650f20afa95d072778fc901ba8c973f67a81b6dbcbf93.pdf\",\n        \"size\":83876,\n        \"mime_type\":\"application/pdf\",\n        \"is_image\":false,\n        \"image_width\":null,\n        \"image_height\":null,\n        \"uploaded_at\":\"2025-09-21T07:41:24.155475+00:00\"\n      }\n    ],\n    \"Part of a set\":[],\n    \"State\":{\n      \"id\":3002,\n      \"value\":\"Production & Used\",\n      \"color\":\"darker-green\"\n    },\n    \"Part Number\":\"40-00075\",\n    \"Revision\":\"A\",\n    \"Notes\":\"Jack for Lambda MU6F PS Control\",\n    \"Sourced By\":{\n      \"id\":2998,\n      \"value\":\"ERA\",\n      \"color\":\"darker-gray\"\n    },\n    \"Containing\":[],\n    \"Contained by\":[]\n  },\n  {\n    \"id\":241,\n    \"order\":\"138.00000000000000000000\",\n    \"Full PN\":\"40-00076 Rev.A\",\n    \"External Part Number\":\"LCR 084M-RSI\",\n    \"Manufacturer\":[\n      {\n        \"id\":103,\n        \"value\":\"Astrodyne TDI\",\n        \"order\":\"39.00000000000000000000\"\n      }\n    ],\n    \"System\":{\n      \"id\":2963,\n      \"value\":\"DC Power Supply\",\n      \"color\":\"orange\"\n    },\n    \"Item description\":\"Low Leakage Filtered Power Entry Modules with Double Fuse Holder and Red Illuminated Switch (Medical)\",\n    \"Price per unit\":\"19.53\",\n    \"Image\":[\n      {\n        \"url\":\"http://localhost/media/user_files/HgmKkT4PcUZB0YjqUZXf58k4NW6nTWDm_523ad844edb9a4dd60654460fe76350a1581222bee42de21023a8c019a14df6d.png\",\n        \"thumbnails\":{\n          \"tiny\":{\n            \"url\":\"http://localhost/media/thumbnails/tiny/HgmKkT4PcUZB0YjqUZXf58k4NW6nTWDm_523ad844edb9a4dd60654460fe76350a1581222bee42de21023a8c019a14df6d.png\",\n            \"width\":null,\n            \"height\":21\n          },\n          \"small\":{\n            \"url\":\"http://localhost/media/thumbnails/small/HgmKkT4PcUZB0YjqUZXf58k4NW6nTWDm_523ad844edb9a4dd60654460fe76350a1581222bee42de21023a8c019a14df6d.png\",\n            \"width\":48,\n            \"height\":48\n          },\n          \"card_cover\":{\n            \"url\":\"http://localhost/media/thumbnails/card_cover/HgmKkT4PcUZB0YjqUZXf58k4NW6nTWDm_523ad844edb9a4dd60654460fe76350a1581222bee42de21023a8c019a14df6d.png\",\n            \"width\":300,\n            \"height\":160\n          }\n        },\n        \"visible_name\":\"image.png\",\n        \"name\":\"HgmKkT4PcUZB0YjqUZXf58k4NW6nTWDm_523ad844edb9a4dd60654460fe76350a1581222bee42de21023a8c019a14df6d.png\",\n        \"size\":15300,\n        \"mime_type\":\"image/png\",\n        \"is_image\":true,\n        \"image_width\":150,\n        \"image_height\":149,\n        \"uploaded_at\":\"2025-10-12T13:56:28.836708+00:00\"\n      }\n    ],\n    \"Source\":\"https://mou.sr/3VYY2CD\",\n    \"Order Items\":[],\n    \"Datasheet\":[\n      {\n        \"url\":\"http://localhost/media/user_files/8wmeFLiwXPFCd5rQtSDIdCV5ZsTHxIpp_27d0193a4735db3da3e82a1a225af37cd2c5de64a8e1359630202784ef5fc726.pdf\",\n        \"thumbnails\":null,\n        \"visible_name\":\"Astrodyne TDI_09272018_LCR 084M-RSI.pdf\",\n        \"name\":\"8wmeFLiwXPFCd5rQtSDIdCV5ZsTHxIpp_27d0193a4735db3da3e82a1a225af37cd2c5de64a8e1359630202784ef5fc726.pdf\",\n        \"size\":576080,\n        \"mime_type\":\"application/pdf\",\n        \"is_image\":false,\n        \"image_width\":null,\n        \"image_height\":null,\n        \"uploaded_at\":\"2025-10-12T14:01:37.990398+00:00\"\n      }\n    ],\n    \"Part of a set\":[],\n    \"State\":{\n      \"id\":3002,\n      \"value\":\"Production & Used\",\n      \"color\":\"darker-green\"\n    },\n    \"Part Number\":\"40-00076\",\n    \"Revision\":\"A\",\n    \"Notes\":\"Fuses not included\",\n    \"Sourced By\":{\n      \"id\":2998,\n      \"value\":\"ERA\",\n      \"color\":\"darker-gray\"\n    },\n    \"Containing\":[],\n    \"Contained by\":[]\n  },\n  {\n    \"id\":242,\n    \"order\":\"139.00000000000000000000\",\n    \"Full PN\":\"xx-nnnnn Rev.A\",\n    \"External Part Number\":\"N/A\",\n    \"Manufacturer\":[],\n    \"System\":null,\n    \"Item description\":\"Low Leakage Filtered Power Entry Modules with\",\n    \"Price per unit\":null,\n    \"Image\":[],\n    \"Source\":\"\",\n    \"Order Items\":[],\n    \"Datasheet\":[],\n    \"Part of a set\":[],\n    \"State\":null,\n    \"Part Number\":\"xx-nnnnn\",\n    \"Revision\":\"A\",\n    \"Notes\":\"\",\n    \"Sourced By\":null,\n    \"Containing\":[],\n    \"Contained by\":[]\n  },\n  {\n    \"id\":243,\n    \"order\":\"140.00000000000000000000\",\n    \"Full PN\":\"xx-nnnnn Rev.A\",\n    \"External Part Number\":\"N/A\",\n    \"Manufacturer\":[],\n    \"System\":null,\n    \"Item description\":\"Double Fuse Holder and Red Illuminated Switch (Medical)\",\n    \"Price per unit\":null,\n    \"Image\":[],\n    \"Source\":\"\",\n    \"Order Items\":[],\n    \"Datasheet\":[],\n    \"Part of a set\":[],\n    \"State\":null,\n    \"Part Number\":\"xx-nnnnn\",\n    \"Revision\":\"A\",\n    \"Notes\":\"\",\n    \"Sourced By\":null,\n    \"Containing\":[],\n    \"Contained by\":[]\n  },\n  {\n    \"id\":244,\n    \"order\":\"141.00000000000000000000\",\n    \"Full PN\":\"xx-nnnnn Rev.A\",\n    \"External Part Number\":\"N/A\",\n    \"Manufacturer\":[],\n    \"System\":null,\n    \"Item description\":\"\",\n    \"Price per unit\":null,\n    \"Image\":[],\n    \"Source\":\"\",\n    \"Order Items\":[],\n    \"Datasheet\":[],\n    \"Part of a set\":[],\n    \"State\":null,\n    \"Part Number\":\"xx-nnnnn\",\n    \"Revision\":\"A\",\n    \"Notes\":\"\",\n    \"Sourced By\":null,\n    \"Containing\":[],\n    \"Contained by\":[]\n  },\n  {\n    \"id\":245,\n    \"order\":\"142.00000000000000000000\",\n    \"Full PN\":\"40-00077 Rev.A\",\n    \"External Part Number\":\"PSG01278\",\n    \"Manufacturer\":[\n      {\n        \"id\":104,\n        \"value\":\"Pro Signal (Farnell OEM)\",\n        \"order\":\"40.00000000000000000000\"\n      }\n    ],\n    \"System\":{\n      \"id\":2965,\n      \"value\":\"Foot Switch\",\n      \"color\":\"deep-dark-orange\"\n    },\n    \"Item description\":\"XLR Connector, 3 Contacts, Socket, Panel Mount, Nickel Plated Contacts, Metal Body\",\n    \"Price per unit\":\"1.85\",\n    \"Image\":[\n      {\n        \"url\":\"http://localhost/media/user_files/BRiqXZVbXIHVCO6TdFfacD6SNrCUQPAn_a72b59afd95ca9a21bb021b5266531df26b7914bc5cdeb4232bf84c631cbc63d.png\",\n        \"thumbnails\":{\n          \"tiny\":{\n            \"url\":\"http://localhost/media/thumbnails/tiny/BRiqXZVbXIHVCO6TdFfacD6SNrCUQPAn_a72b59afd95ca9a21bb021b5266531df26b7914bc5cdeb4232bf84c631cbc63d.png\",\n            \"width\":null,\n            \"height\":21\n          },\n          \"small\":{\n            \"url\":\"http://localhost/media/thumbnails/small/BRiqXZVbXIHVCO6TdFfacD6SNrCUQPAn_a72b59afd95ca9a21bb021b5266531df26b7914bc5cdeb4232bf84c631cbc63d.png\",\n            \"width\":48,\n            \"height\":48\n          },\n          \"card_cover\":{\n            \"url\":\"http://localhost/media/thumbnails/card_cover/BRiqXZVbXIHVCO6TdFfacD6SNrCUQPAn_a72b59afd95ca9a21bb021b5266531df26b7914bc5cdeb4232bf84c631cbc63d.png\",\n            \"width\":300,\n            \"height\":160\n          }\n        },\n        \"visible_name\":\"image.png\",\n        \"name\":\"BRiqXZVbXIHVCO6TdFfacD6SNrCUQPAn_a72b59afd95ca9a21bb021b5266531df26b7914bc5cdeb4232bf84c631cbc63d.png\",\n        \"size\":555834,\n        \"mime_type\":\"image/png\",\n        \"is_image\":true,\n        \"image_width\":1033,\n        \"image_height\":1262,\n        \"uploaded_at\":\"2025-10-15T07:39:02.928518+00:00\"\n      },\n      {\n        \"url\":\"http://localhost/media/user_files/cD4DiZernLg1IcMgN7upCwtZS2FtKAIu_c8924d17789bc244d08a1b25431cd60c6879a8a97d97b88ef7395165ca5288f5.webp\",\n        \"thumbnails\":{\n          \"tiny\":{\n            \"url\":\"http://localhost/media/thumbnails/tiny/cD4DiZernLg1IcMgN7upCwtZS2FtKAIu_c8924d17789bc244d08a1b25431cd60c6879a8a97d97b88ef7395165ca5288f5.webp\",\n            \"width\":null,\n            \"height\":21\n          },\n          \"small\":{\n            \"url\":\"http://localhost/media/thumbnails/small/cD4DiZernLg1IcMgN7upCwtZS2FtKAIu_c8924d17789bc244d08a1b25431cd60c6879a8a97d97b88ef7395165ca5288f5.webp\",\n            \"width\":48,\n            \"height\":48\n          },\n          \"card_cover\":{\n            \"url\":\"http://localhost/media/thumbnails/card_cover/cD4DiZernLg1IcMgN7upCwtZS2FtKAIu_c8924d17789bc244d08a1b25431cd60c6879a8a97d97b88ef7395165ca5288f5.webp\",\n            \"width\":300,\n            \"height\":160\n          }\n        },\n        \"visible_name\":\"1280896-500.webp\",\n        \"name\":\"cD4DiZernLg1IcMgN7upCwtZS2FtKAIu_c8924d17789bc244d08a1b25431cd60c6879a8a97d97b88ef7395165ca5288f5.webp\",\n        \"size\":2992,\n        \"mime_type\":\"image/webp\",\n        \"is_image\":true,\n        \"image_width\":170,\n        \"image_height\":200,\n        \"uploaded_at\":\"2025-10-15T07:41:19.058322+00:00\"\n      }\n    ],\n    \"Source\":\"https://il.farnell.com/pro-signal/psg01278/socket-xlr-chassis-black-metal/dp/1280896\",\n    \"Order Items\":[],\n    \"Datasheet\":[\n      {\n        \"url\":\"http://localhost/media/user_files/Uyf7t4tZZzrzP57iXYrswansEokoFFZg_2a5d2a180063cfe1f33c25b479c5b7619473aeec8531d10543112d049600bd2d.pdf\",\n        \"thumbnails\":null,\n        \"visible_name\":\"1671429.pdf\",\n        \"name\":\"Uyf7t4tZZzrzP57iXYrswansEokoFFZg_2a5d2a180063cfe1f33c25b479c5b7619473aeec8531d10543112d049600bd2d.pdf\",\n        \"size\":113525,\n        \"mime_type\":\"application/pdf\",\n        \"is_image\":false,\n        \"image_width\":null,\n        \"image_height\":null,\n        \"uploaded_at\":\"2025-10-15T07:43:25.126439+00:00\"\n      }\n    ],\n    \"Part of a set\":[],\n    \"State\":{\n      \"id\":3002,\n      \"value\":\"Production & Used\",\n      \"color\":\"darker-green\"\n    },\n    \"Part Number\":\"40-00077\",\n    \"Revision\":\"A\",\n    \"Notes\":\"\",\n    \"Sourced By\":{\n      \"id\":2998,\n      \"value\":\"ERA\",\n      \"color\":\"darker-gray\"\n    },\n    \"Containing\":[],\n    \"Contained by\":[]\n  },\n  {\n    \"id\":246,\n    \"order\":\"143.00000000000000000000\",\n    \"Full PN\":\"xx-nnnnn Rev.A\",\n    \"External Part Number\":\"N/A\",\n    \"Manufacturer\":[],\n    \"System\":null,\n    \"Item description\":\"\",\n    \"Price per unit\":null,\n    \"Image\":[],\n    \"Source\":\"\",\n    \"Order Items\":[],\n    \"Datasheet\":[],\n    \"Part of a set\":[],\n    \"State\":null,\n    \"Part Number\":\"xx-nnnnn\",\n    \"Revision\":\"A\",\n    \"Notes\":\"\",\n    \"Sourced By\":null,\n    \"Containing\":[],\n    \"Contained by\":[]\n  }\n]") -> (0 "Error out":errorcluster, 3 "BOM Items Raw Data":T1[](array[typedef]))   [LabVIEW 2018]
uses:
  TypeDef/BOM Table Raw Items.ctl
  <vilib>/JDP Science/JSONtext/JSONtext.lvlib
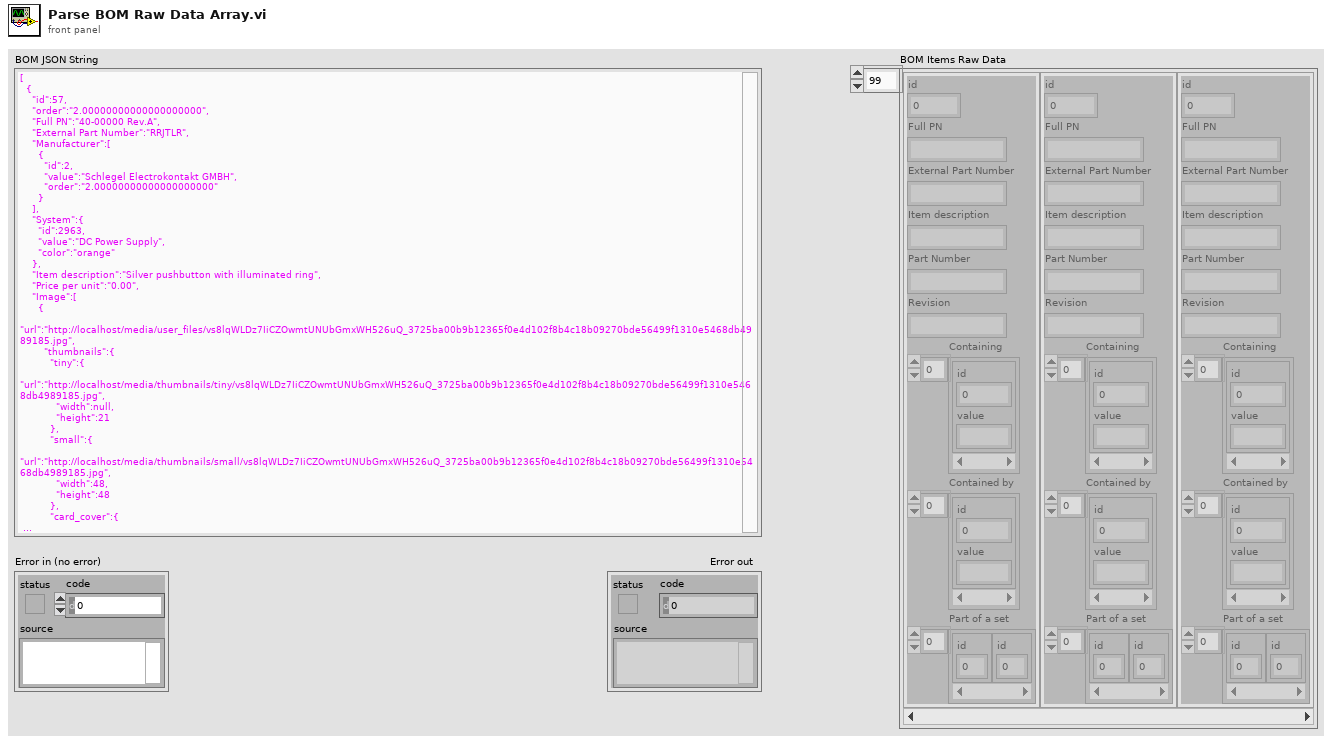
[diagram p1: front panel]
types:
  T1 = typedef "BOM Table Raw Items.ctl" = cluster{"id":i32, "Full PN":string, "External Part Number":string, "Item description":string, "Part Number":string, "Revision":string, "Containing":cluster{"id":i32, "value":string}[], "Contained by":cluster{"id":i32, "value":string}[], "Part of a set":cluster{"id":i32}[]}
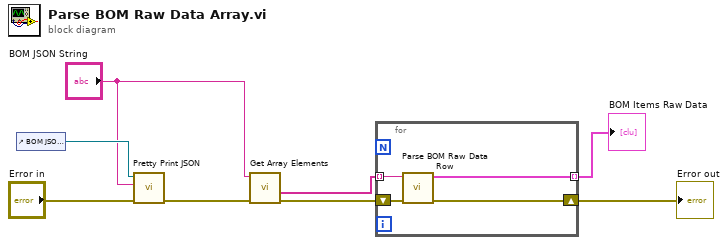
[diagram p0: block diagram]
diagram:
  n1 = control-ref of="BOM JSON String"() -> (w4:refnum<vi>)
  n2 = call "Pretty Print JSON.vi"("error in (no error)"="Error in", "JSON in"="BOM JSON String", "String in"=w4) -> ("error out"=w1:errorcluster)  [unwired: 8 in]
  n3 = call <vilib>:"Get Array Elements.vi"("error in (no error)"=w1, "JSON"="BOM JSON String") -> ("error out"=w7:errorcluster, "<JSON>"=w8:string[])  [unwired: 7 in, 1 out]
  n4 = for {
    tunnel: w8 -> [w12] mode=indexing
    tunnel: [w9] -> w5 mode=indexing
    shift-right: [w10] -> w6
    shift-left: w7 -> [w11]
    n5 = call "Parse BOM Raw Data Row.vi"("error in (no error)"=w11, "BOM Table Row JSON"=w12) -> ("error out"=w10:errorcluster, "BOM Table Raw Items"=w9:T1)  [unwired: 8 in]
  }
  "Error out" <- w6
  "BOM Items Raw Data" <- w5
